vi "scanner v1.9.3.vi"() -> ()   [LabVIEW 2015]
uses:
  <vilib>/Analysis/Matrix/Datatypes/RealMatrix.ctl
  libs/Controls/String.ctl
  libs/Controls/Number.ctl
  libs/Controls/outofrange.ctl
  libs/Controls/loopclock.ctl
  libs/Controls/AcquisitionModuleStates.ctl
  <vilib>/Analysis/6fits.llb/Curve Fitting Criteria.ctl
  <vilib>/Utility/miscctls.llb/LVFormatAndPrecisionTypeDef.ctl
  <vilib>/Utility/file.llb/Write To Spreadsheet File (string).vi
  <vilib>/Utility/file.llb/Write Delimited Spreadsheet (I64).vi
  <vilib>/Utility/file.llb/Write To Spreadsheet File (DBL).vi
  libs/GlobalParameters/SpectraData2.vi
  <vilib>/Utility/file.llb/Read From Spreadsheet File (string).vi
  <vilib>/Analysis/Matrix/NI_Matrix.lvlib
  <vilib>/Analysis/NI_AALPro.lvlib
  Zaber A Series/Zaber A Series.lvlib
  libs/XGL_DPP.lvlib
panel:
  out "Error code 2":i32
  out "x/y":dbl
  out "Waveform Graph":dbl[][](graph)
  out "DPP Configuration":T1={"reset_recovery_time"=300, "edge_peaking_time"=5, "flat_top"=5, "peaking_time"=25, "gain"=1.0, "max_risetime"=35.0, "fast_filter_thr"=100, "zero_peak_freq"=5.0, "inverted_input"=0, "base_offset"=0, "reset_threshold"=1000, "overflow_recovery"=0, "tail_coefficient"=0.0, "energy_filter_thr"=25, "energy_baseline_thr"=25, "max_peaking_time"=0, "edge_flat_top"=1, "time_constant"=0.0, "baseline_samples"=64, "other_param"=0}
  in  "Precision [mm]":dbl=0.1
  out "Port":refnum<visa-resource-name>
  out "MotorsReady":bool
  out "Enum":T2=enum."SaveSpectra"
  out "init1Dset":dbl[][](array[numeric])
  out "3D":bool
  out "MAP":bool
  out "queue mode":bool
  out "scan mode":bool
  in  "Data folder path":path=path "d:/Users/XRF/Desktop/Scan DATA"
  out "Speed 2":T3 scale=0.0..30.0
  in  "Tab Control":T4(tab)
  in  "StopMotion":bool
  in  "GoToZ":bool
  in  "GoToY":bool
  in  "GoToX":bool
  in  "GoTo Z [mm]":dbl format="%#.8g"
  in  "GoTo Y [mm]":dbl format="%#.8g"
  in  "GoTo X [mm]":dbl format="%#.8g"
  out "ZnotEqual":bool
  out "ScanReady?":bool
  in  "OpenScanBuilder":bool
  in  "Clear":bool
  in  "LowerRight":bool
  in  "LowerLeft":bool
  in  "UpperRight":bool
  in  "UpperLeft":bool
  in  "Reduced Speed":bool
  in  "Speed Z [mm/s]":dbl(slide) caption="Z Speed\n[mm/s]" min=0.5 max=10.0 step=0.5 scale=0.5..10.0
  in  "XY Speed\n[mm/s]":dbl(slide)=1.0 min=1.0 max=75.0 step=1.0 scale=1.0..20.0
  in  "Away":bool
  in  "Closer":bool
  in  "Right":bool
  in  "Left":bool
  in  "Down":bool
  in  "Up":bool
  out "X [mm]":dbl format="%#.8g"
  out "Y [mm]":dbl format="%#.8g"
  out "Z [mm]":dbl format="%#.3g"
  out "Scan\nCorners":dbl[][](array[numeric])
  in  "QUICKSCAN_Start 2":bool
  in  "Add To Queue 2":bool
  out "Assignment":cluster{"Microstep Size":dbl, "Device":string}[](array[cluster])
  in  "Acceleration [mm/s^2]":dbl=1.0 min=1.0 max=488.0
  out "SpectraPlot":u64[](graph) caption="Waveform Graph"
  in  "APPEARANCE_CursorVis":bool
  in  "APPEARANCE_E/CH":bool
  in  "APPEARANCE_Log/Lin":bool=TRUE
  in  "Tab":enum32{"ACQUISITION", "ROIS", "CALIBRATION"}(tab)
  in  "Configure":bool
  in  "Time per spectrum [ms]":u32=10 max=1000000
  in  "Map points":u32=10
  in  "Acquisition mode":u16(ring) items=["Single spectrum", "Multiple spectra"]
  in  "Acquisition time [s]":fxp<+,64,32>=10.0
  out "Acq. in progress":bool
  in  "Stop":bool
  in  "Get connected":bool
  out "identifier out":string
  in  "IP Address":string="10.96.0.110"
  in  "Add IP":bool
  in  "Init":bool
  out "Real Time [s]":dbl=1.0 min=0.2 step=0.1
  out "Live Time [s]":dbl=1.0 min=0.2 step=0.1
  in  "MEASUREMENT_Start":bool
  out "Elapsed Time":dbl caption="Elapsed Time [s]" format="%#_4g"
  in  "Preset Time [s]":dbl=1.0 min=0.2 step=0.1
  out "Progress":u32 caption="%" min=1 step=1
  out "Library state":bool
  in  "?":bool
  in  "Config. file path":path=path "Configuration files/DefaultParameters.xml"
  out "Error code":i32
  in  "ROI_Load":bool
  in  "ROI_Save":bool
  in  "ROI_Cancel":bool
  in  "ROI_LowCh":u32=1800 caption="Lower Channel"
  in  "ROI_Set":bool
  in  "ROI_Add":bool
  in  "ROI_Remove":bool
  in  "ROI_RemoveAll":bool
  in  "ROI_UpCh":u32=2000 caption="Upper Channel"
  out "ROI_Array":T7(array[cluster]) {"ROI begin channel" step=0.001; "ROI end channel" step=0.001; "Intensity" step=0.001; "Net Intensity" step=0.001; "Gauss Fit" step=0.001; "FWHM [keV]" step=0.001; "Center [keV]" step=0.001}
  out "Intercept":dbl=-0.03941267387944358 caption="Intercept (keV)" format="%#_6f"
  out "Slope":dbl=0.010046367851622875 caption="Slope (keV/channel)" format="%#.6f"
  in  "CALIB_ClearPoints":bool
  in  "CALIB_AddPoint":bool
  in  "CalibArray":T8
  in  "CALIB_Execute":bool
  in  "SpectrumType":u16(ring) items=["Cumulative Spectra", "Max Spectra", "Last Spectra"]
  out "Cumul. LT[s]":dbl=1.0 min=0.0 step=1.0
  in  "Lin/Log":u16(ring) items=["Lin", "Log"]
  in  "Stop Button":bool
  out "/":i32=1 min=0 step=1
  out "current point":i32=1 min=0 step=1
  out "1D graph 1":dbl[](graph) caption="Map2"
  in  "MAP-L":u16(ring) items=["Cu-Ka", "All"]
  out "2D graph 2":dbl[][](graph) caption="A"
  out "2D graph 1":dbl[][](graph) caption="A"
  in  "MAP-R":u16(ring) items=["Cu-Ka", "All"]
  out "1D graph 2":dbl[](graph) caption="Map2"
  out "last point movement duration [ms]":u32
  in  "Free running":bool
  in  "PresetROI":u16(ring)
  in  "Preset type:":enum32{"Live time [s]", "Counts"}(radio)
  in  "Add To Queue":bool
  in  "ScanName:":string caption="Scan Name:"
  in  "Snake?":bool
  in  "PresetVal":dbl caption="Time Preset [s]"
  in  "QUICKSCAN_Start":bool
  in  "Scan order":u16(ring)=1 items=["X->Z->Y"=6, "Y->Z->X"=5, "Z->X->Y"=3, "Y->X->Z"=2, "Z->Y->X"=4, "X->Y->Z"=1]
  out "Z error":T9
  out "Y error":T9
  out "X error":T9
  out "total # of points":i32=1 min=0 step=1
  in  "Scan definition by":T10(radio)
  in  "Z steps":i32=1 min=1 step=1
  in  "step Z [mm]":dbl=1.0 min=0.0 step=0.1
  in  "Z end [mm]":dbl
  in  "Z start [mm]":dbl
  in  "Y steps":i32=1 min=1 step=1
  in  "X steps":i32=1 min=1 step=1
  in  "step Y [mm]":dbl=1.0 min=0.0 step=0.1
  in  "Y end [mm]":dbl=1.0
  in  "Y start [mm]":dbl
  in  "step X [mm]":dbl=1.0 min=0.0 step=0.1
  in  "X end [mm]":dbl=1.0
  in  "X start [mm]":dbl
  in  "Delete":bool
  in  "Text Ring":u16(ring)
  out "estimated duration":string caption="Estimated duration:"
  out "NoOfScans":i32=1 min=0 step=1
  in  "QUEUE_Stop":bool
  in  "QUEUE_Run":bool
  out "ScanQueue":T11(array[cluster])
  in  "Clear_Queue":bool
  out "SumSpectra":u64[](array[numeric])
  out "MaxSpectra":u64[](array[numeric])
  out "Array of positions":dbl[][](array[numeric])
  out "LastSpectra":u32[](graph) caption="Waveform Graph"
  out "maps folder":path
  out "spectra folder":path
  out "roi intensities 2d":dbl[](array[numeric])
  out "Array":dbl[](array[numeric])
  out "2DSet":dbl[][][](array[numeric])
  out "1DSet":dbl[][](array[numeric])
  out "1DPosArray":dbl[](array[numeric])
  out "appended path":path
  out "Numeric":i32
  out "ScanData":T12
  out "ZaberError":errorcluster
  out "ReadoutTiming":u32[](array[numeric])
  out "Loop Speed [1/s]":dbl caption="Elapsed Time [s]" format="%#_2f"
  # "This is for debugging purposes"
  # "Capture position as:"
  # "ROI  Name       Begin           End         Intensity    Net intnsity   Gauss Fit      FWHM         Center\n                         channel      channel                                                              [keV]            [keV]"
  # "Point               Channel      Energy (keV)"
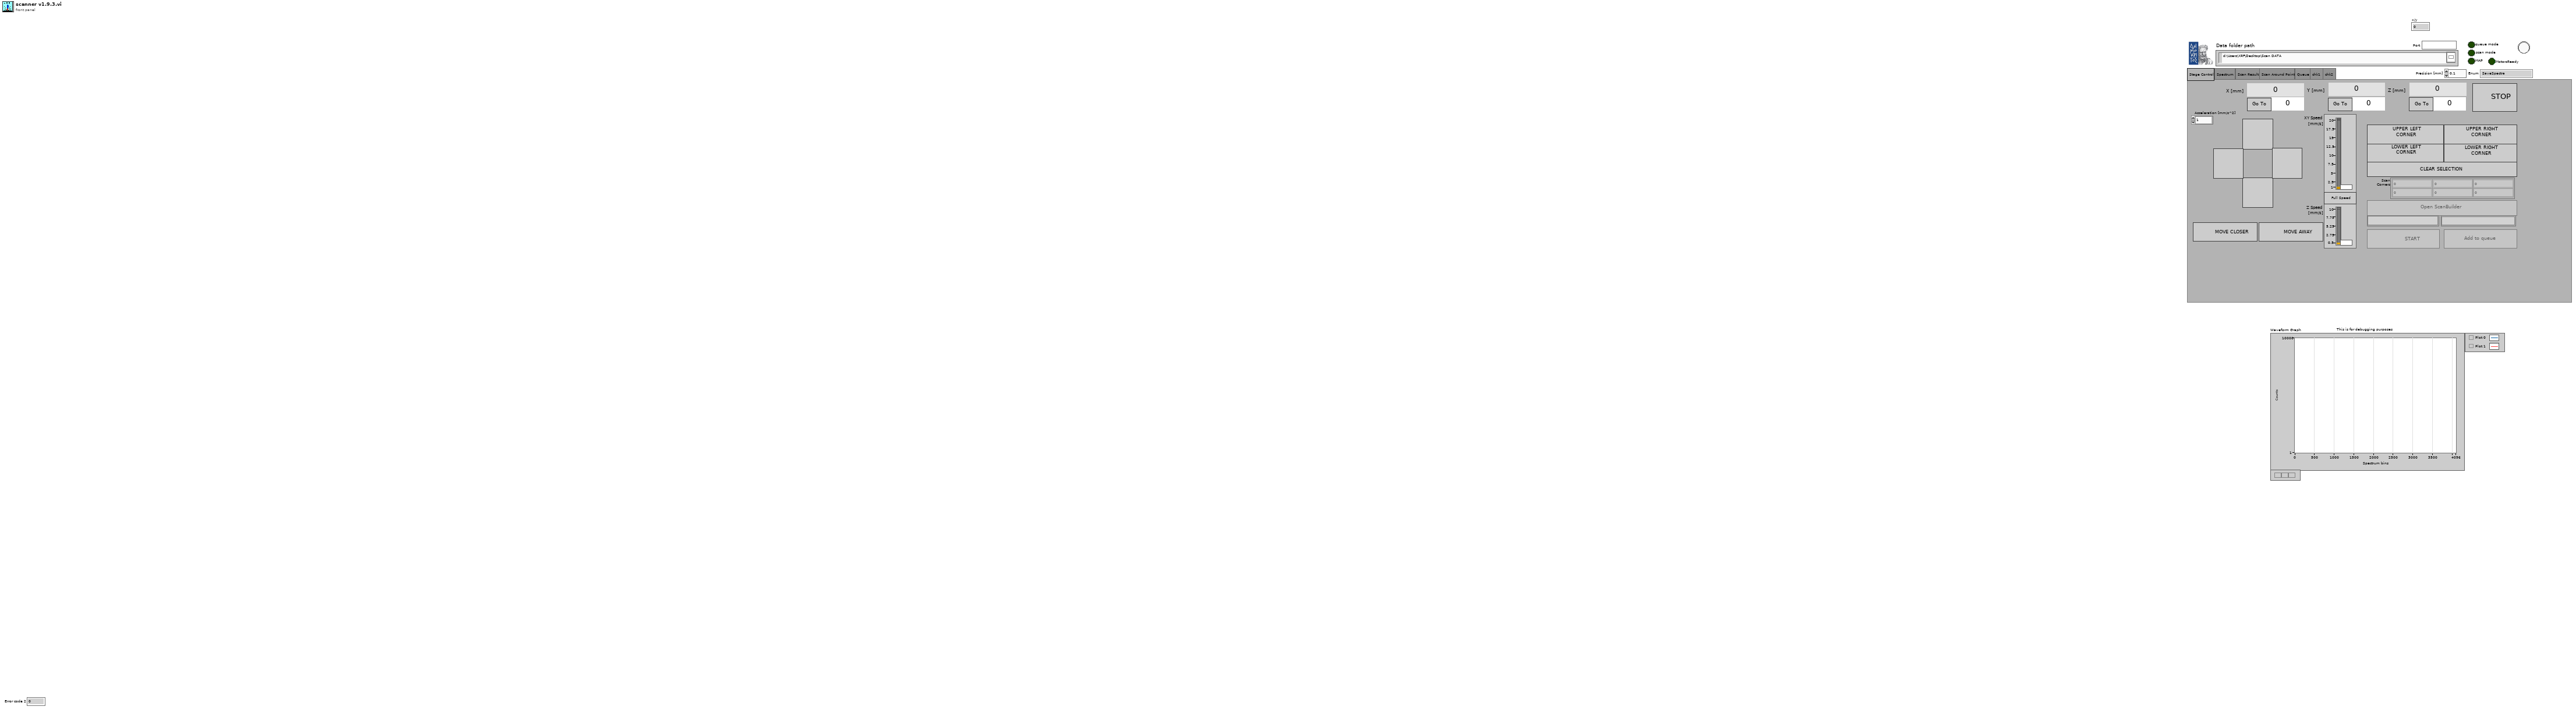
[diagram p1: front panel]
types:
  T1 = cluster{"reset_recovery_time":u32, "edge_peaking_time":u32, "flat_top":u32, "peaking_time":u32, "gain":dbl, "max_risetime":dbl, "fast_filter_thr":u32, "zero_peak_freq":dbl, "inverted_input":u8, "base_offset":u32, "reset_threshold":u32, "overflow_recovery":u32, "tail_coefficient":dbl, "energy_filter_thr":u32, "energy_baseline_thr":u32, "max_peaking_time":u32, "edge_flat_top":u32, "time_constant":dbl, "baseline_samples":u32, "other_param":u32}
  T2 = typedef "AcquisitionModuleStates.ctl" = enum16{"Close", "PrepareMap", "MoveToPoint", "DisplayData", "SaveSpectra", "Acquire", "IDLE", "Initialisation"}
  T3 = typedef "loopclock.ctl" = dbl
  T4 = enum32{"Stage Control", "Spectrum", "Scan Result", "Scan Around Point", "Queue", "chk1", "chk2"}
  T5 = typedef "String.ctl" = string
  T6 = typedef "Number.ctl" = dbl
  T7 = cluster{"ROI name":T5, "ROI begin channel":T6, "ROI end channel":T6, "Intensity":T6, "Net Intensity":T6, "Gauss Fit":T6, "FWHM [keV]":T6, "Center [keV]":T6}[]
  T8 = typedef "NI_Matrix.lvlib/RealMatrix.ctl" = dbl[][]
  T9 = typedef "outofrange.ctl" = bool
  T10 = enum32{"Step size and step number", "Scan boundaries and step size", "Scan boundaries and number of steps"}
  T11 = cluster{"Scan\nCoords \n[mm]":cluster{"X abs start":dbl, "X abs end":dbl, "Y abs start":dbl, "Y abs end":dbl, "Z abs start":dbl, "Z abs end":dbl, "X step":dbl, "Y step":dbl, "Z step":dbl}, "PresetVal":dbl, "Order":u16, "Snake?":bool, "Name":string, "#points":i32, "CtsPreset?":bool, "CtPsetROI":i32}[]
  T12 = cluster{"ScanCoords [mm]":cluster{"X abs start":dbl, "X abs end":dbl, "Y abs start":dbl, "Y abs end":dbl, "Z abs start":dbl, "Z abs end":dbl, "X step":dbl, "Y step":dbl, "Z step":dbl}, "PresetVal":dbl, "Order":u16, "Snake?":bool, "Name":string, "#points":i32, "CtPreset?":bool, "CtPsetROI":i32}
  T13 = cluster{"X min":dbl, "X max":dbl, "Y min":dbl, "Y max":dbl, "Z min":dbl, "Z max":dbl}
  T14 = enum32{"Size Tabs To Contents", "Size All Tabs to Largest Tab", "Fixed Tab Size"}
  T15 = enum8{"Enabled", "Disabled", "Disabled and Grayed Out"}
  T16 = cluster{"ScanCoords [mm]":cluster{"X abs start":dbl, "X abs end":dbl, "Y abs start":dbl, "Y abs end":dbl, "Z abs start":dbl, "Z abs end":dbl, "X step":dbl, "Y step":dbl, "Z step":dbl}, "PresetVal":dbl, "Order":u16, "Snake?":bool, "Name":string, "#points":i32, "ChrgPreset?":bool, "CtPrstROI":i32}
  T17 = cluster{"ROI name":string, "ROI begin channel":i64, "ROI end channel":i64, "Intensity":i64, "Net Intensity":i64, "Gauss Fit":dbl, "FWHM [keV]":dbl, "Center [keV]":dbl}
  T18 = typedef "LVFormatAndPrecisionTypeDef.ctl" = cluster{"Format":u8, "Precision":u8}
  T19 = cluster{"Scan\nCoords \n[mm]":cluster{"X abs start":dbl, "X abs end":dbl, "Y abs start":dbl, "Y abs end":dbl, "Z abs start":dbl, "Z abs end":dbl, "X step":dbl, "Y step":dbl, "Z step":dbl}, "PresetVal":dbl, "Order":u16, "Snake?":bool, "Name":string, "#points":i32, "CtsPreset?":bool, "CtPsetROI":i32}
  T20 = cluster{"X abs start":dbl, "X abs end":dbl, "Y abs start":dbl, "Y abs end":dbl, "Z abs start":dbl, "Z abs end":dbl, "X step":dbl, "Y step":dbl, "Z step":dbl}
  T21 = cluster{"ScanCoords [mm]":cluster{"X abs start":dbl, "X abs end":dbl, "Y abs start":dbl, "Y abs end":dbl, "Z abs start":dbl, "Z abs end":dbl, "X step":dbl, "Y step":dbl, "Z step":dbl}, "PresetVal":dbl, "Order":u16, "Snake?":bool, "Name":string, "#points":i32, "CtPreset?":bool, "CtPsetROI":i32}[]
  T22 = enum16{"Left Button", "Center Button", "Right Button", "Window Close"}
  T23 = cluster{"ScanCoords [mm]":cluster{"X abs start":dbl, "X abs end":dbl, "Y abs start":dbl, "Y abs end":dbl, "Z abs start":dbl, "Z abs end":dbl, "X step":dbl, "Y step":dbl, "Z step":dbl}, "PresetVal":dbl, "Order":u16, "Snake?":bool, "Name":string, "#points":i32, "ChrgPreset?":bool, "CtPsetROI":u16}
  T24 = typedef "LVMinMaxIncTypeDef.ctl" = cluster{"Minimum":dbl, "Maximum":dbl, "Increment":dbl}
  T25 = typedef "LVRangeTypeDef.ctl" = cluster{"Minimum":dbl, "Maximum":dbl, "Increment":dbl, "Minor Increment":dbl, "Start":dbl}
  T26 = typedef "ConfigurationDPP.ctl" = cluster{"reset_recovery_time":u32, "edge_peaking_time":u32, "flat_top":u32, "peaking_time":u32, "gain":dbl, "max_risetime":dbl, "fast_filter_thr":u32, "zero_peak_freq":dbl, "inverted_input":u8, "base_offset":u32, "reset_threshold":u32, "overflow_recovery":u32, "tail_coefficient":dbl, "energy_filter_thr":u32, "energy_baseline_thr":u32, "max_peaking_time":u32, "edge_flat_top":u32, "time_constant":dbl, "baseline_samples":u32, "other_param":u32}
  T27 = cluster{"ROI name":string, "ROI begin channel":i64, "ROI end channel":i64, "Intensity":i64, "Net Intensity":i64, "Gauss Fit":dbl, "FWHM [keV]":dbl, "Center [keV]":dbl}[]
  T28 = typedef "NI_AALPro.lvlib/Curve Fitting Criteria.ctl" = u16
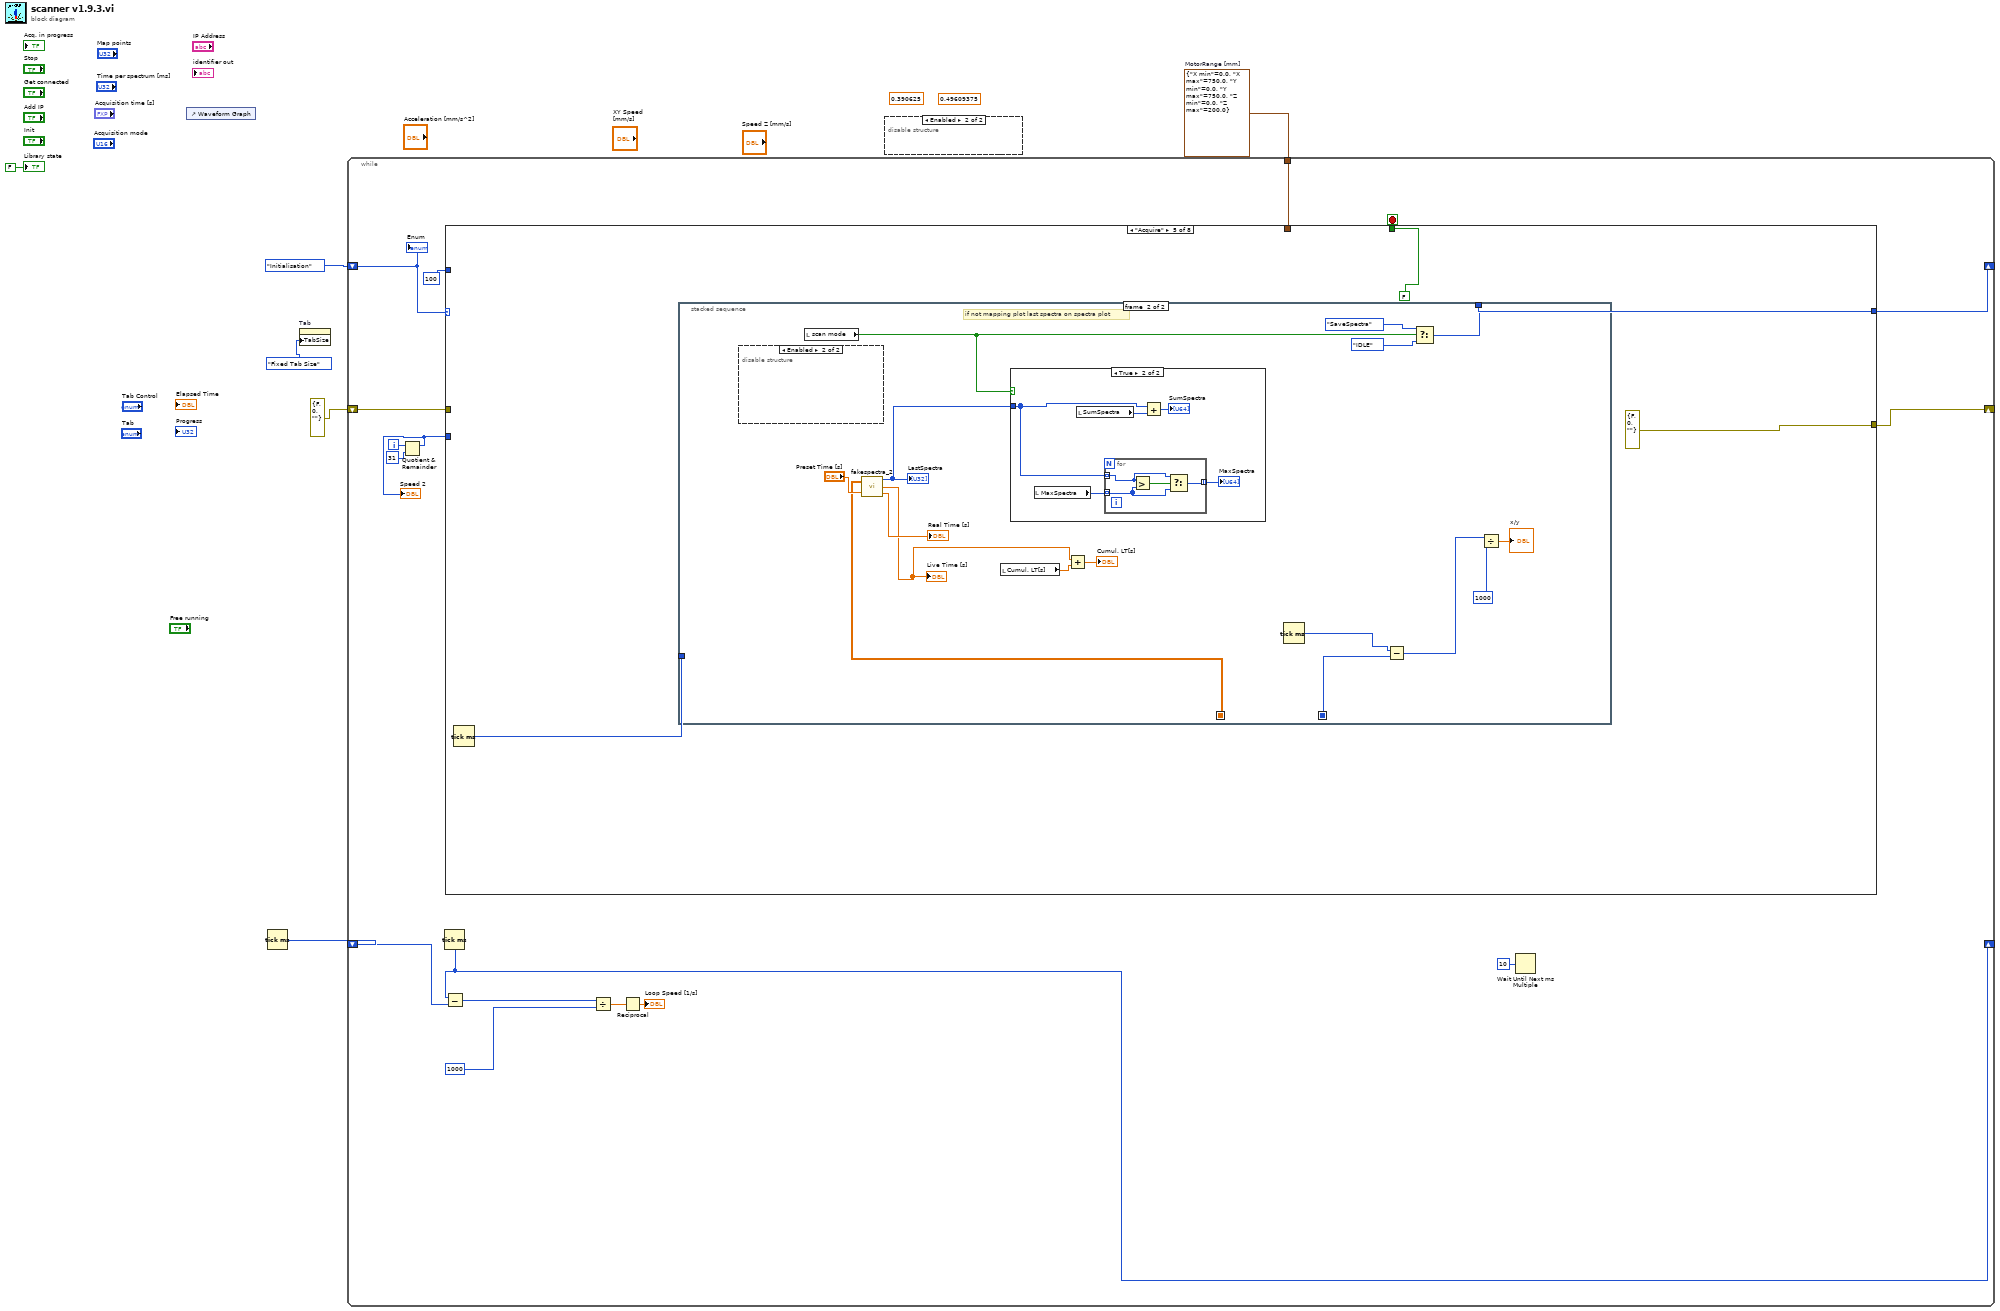
[diagram p0: block diagram]
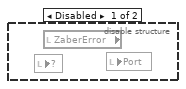
[diagram p2: hidden frame]
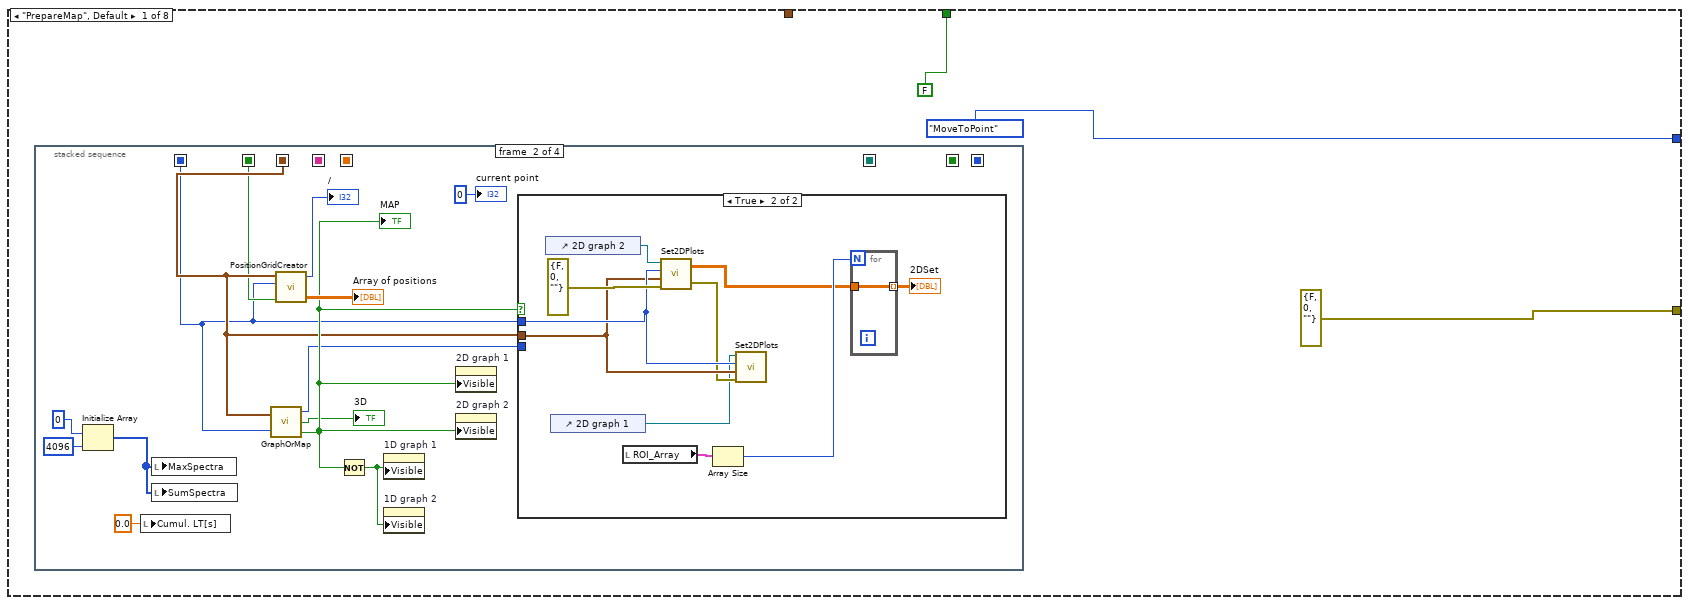
[diagram p3: hidden frame]
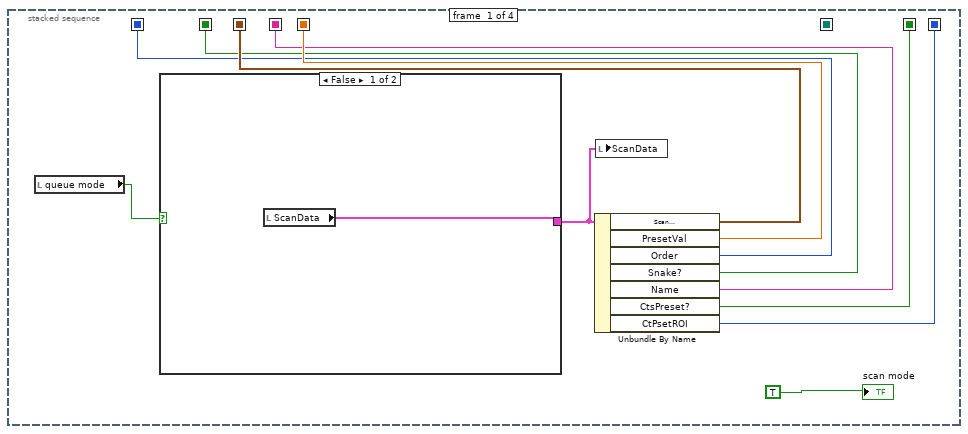
[diagram p4: hidden frame]
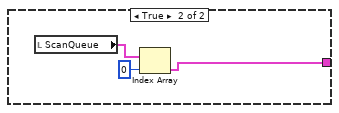
[diagram p5: hidden frame]
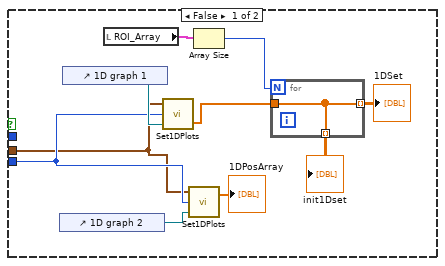
[diagram p6: hidden frame]
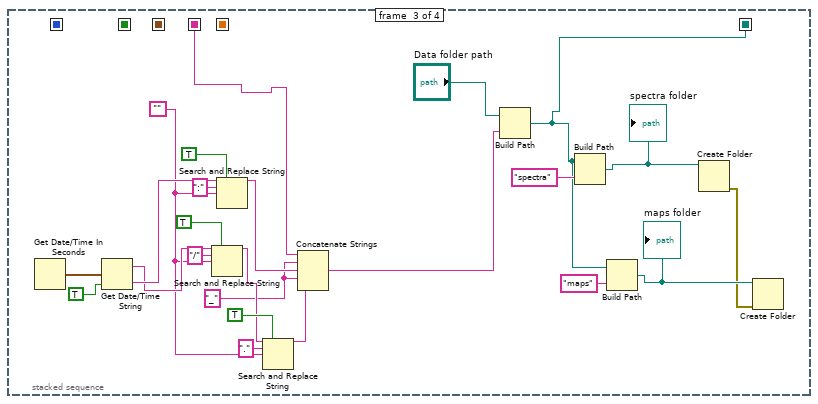
[diagram p7: hidden frame]
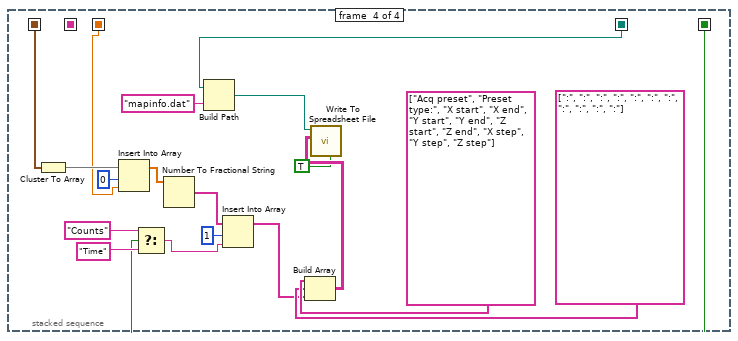
[diagram p8: hidden frame]
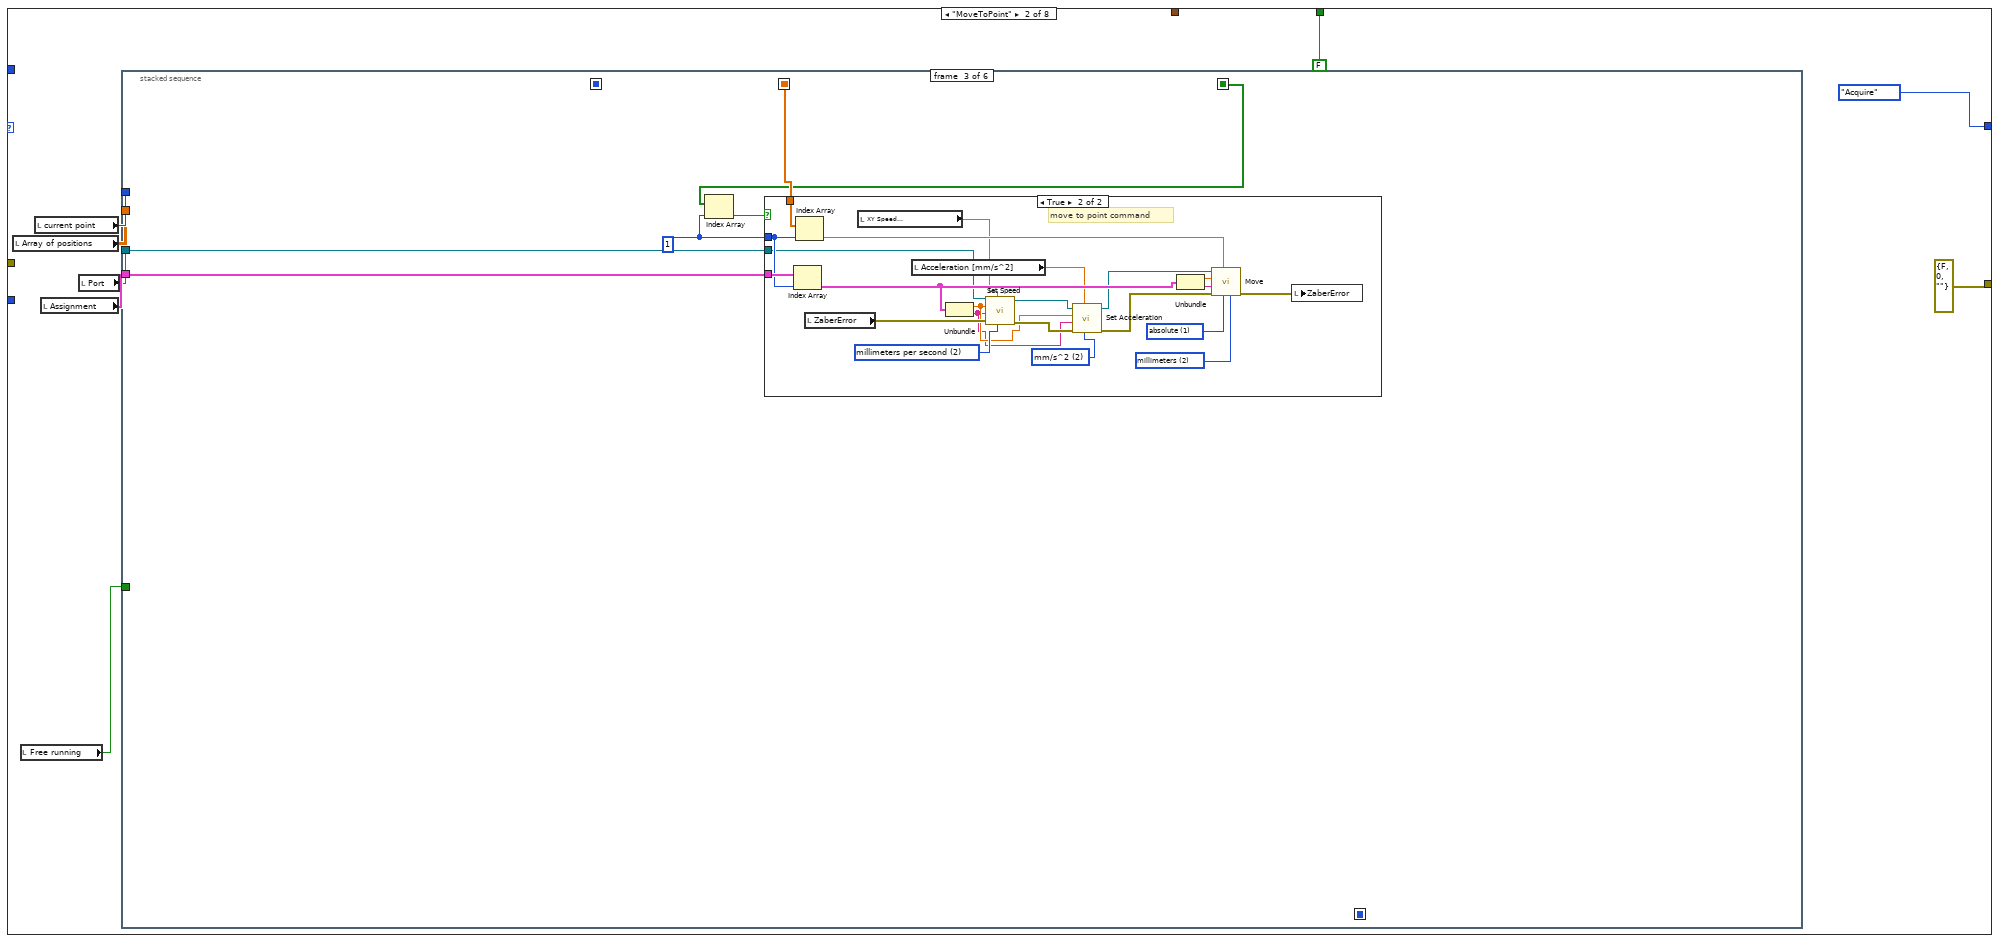
[diagram p9: hidden frame]
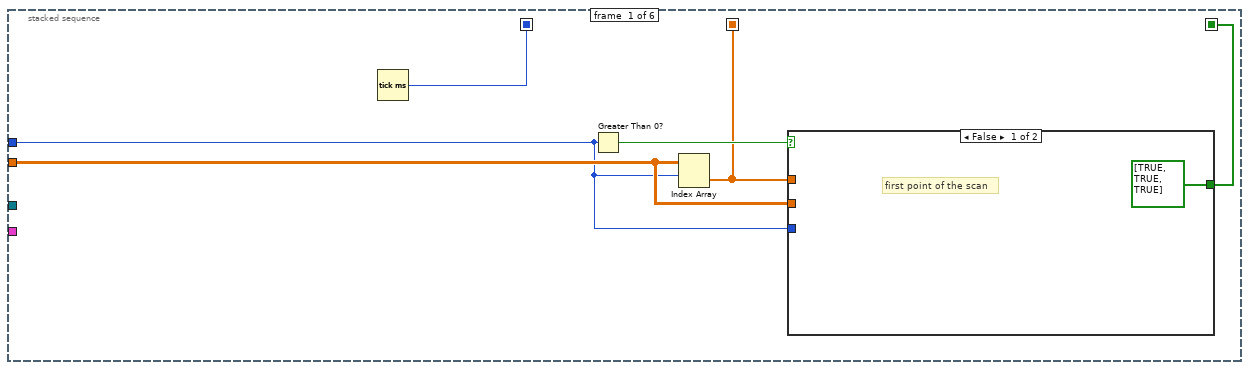
[diagram p10: hidden frame]
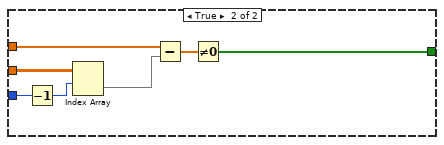
[diagram p11: hidden frame]
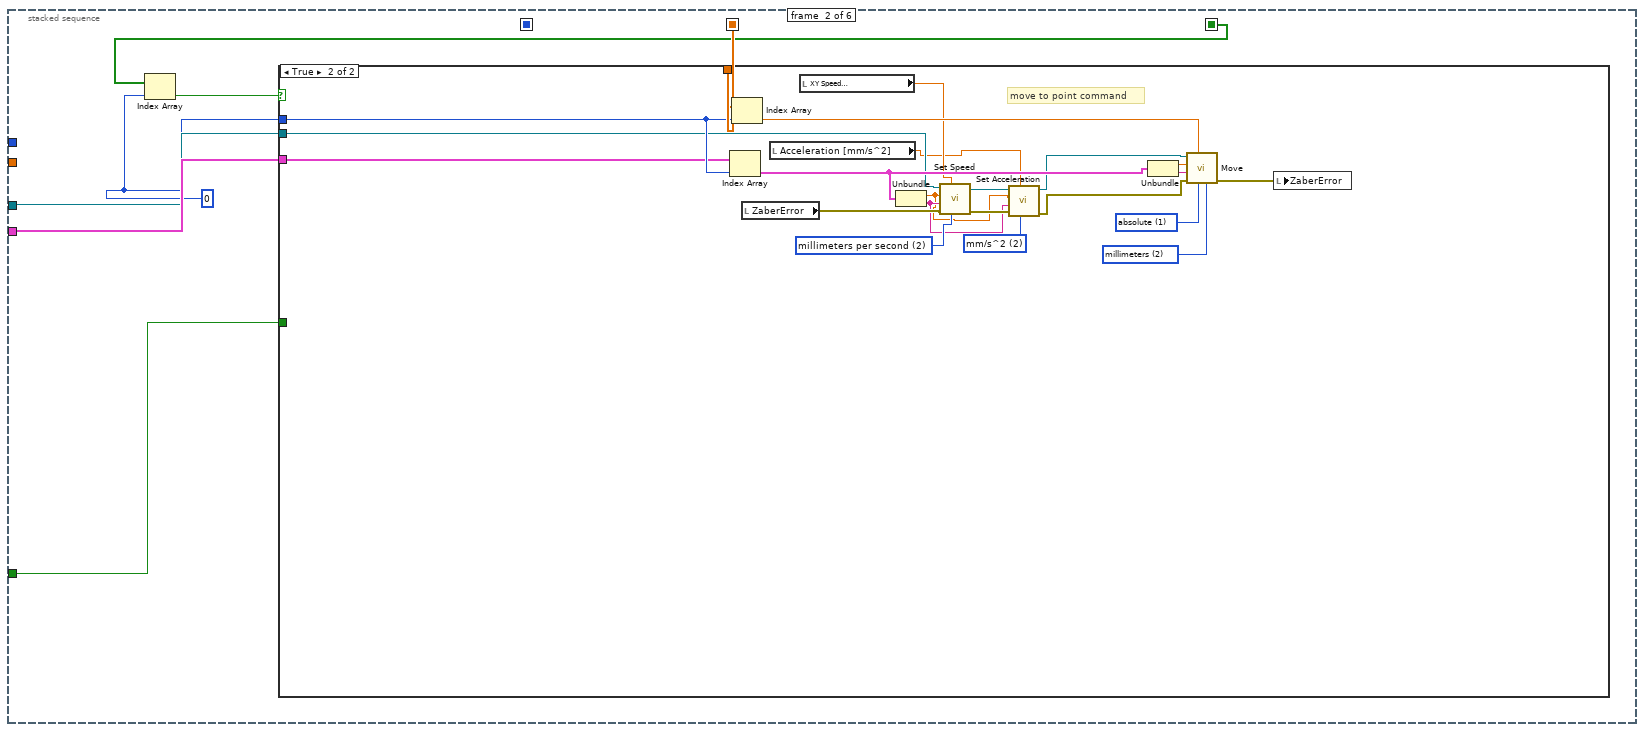
[diagram p12: hidden frame]
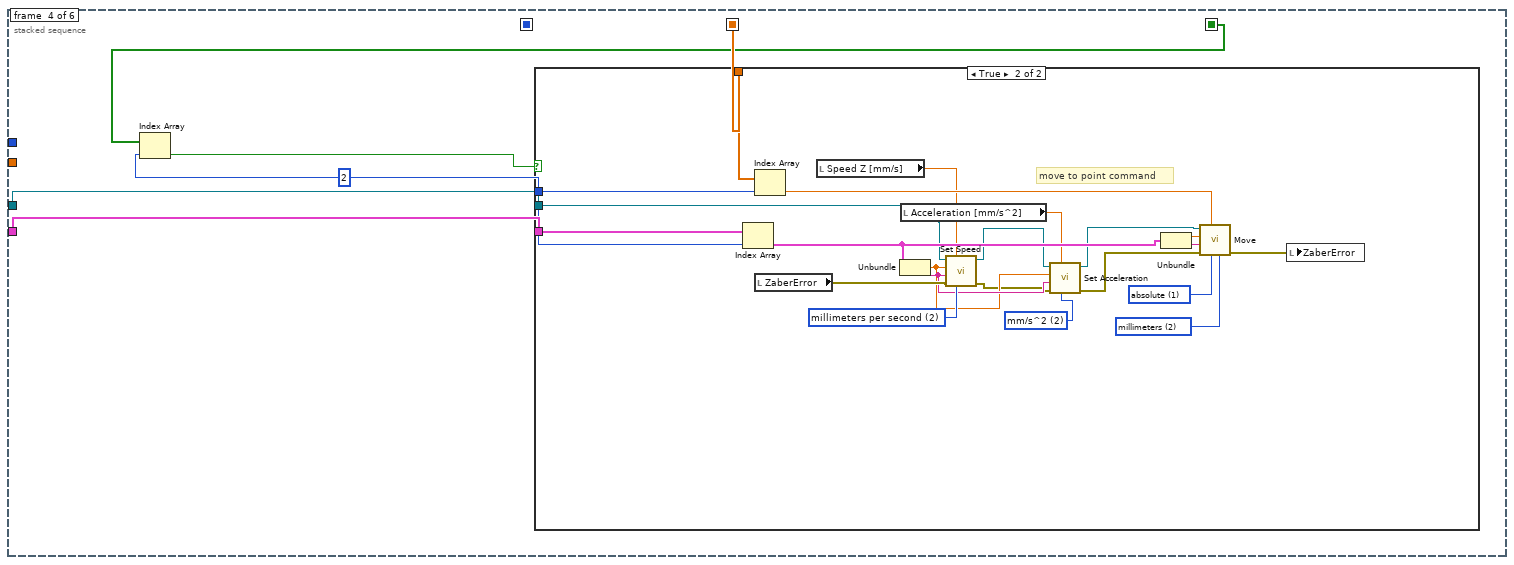
[diagram p15: hidden frame]
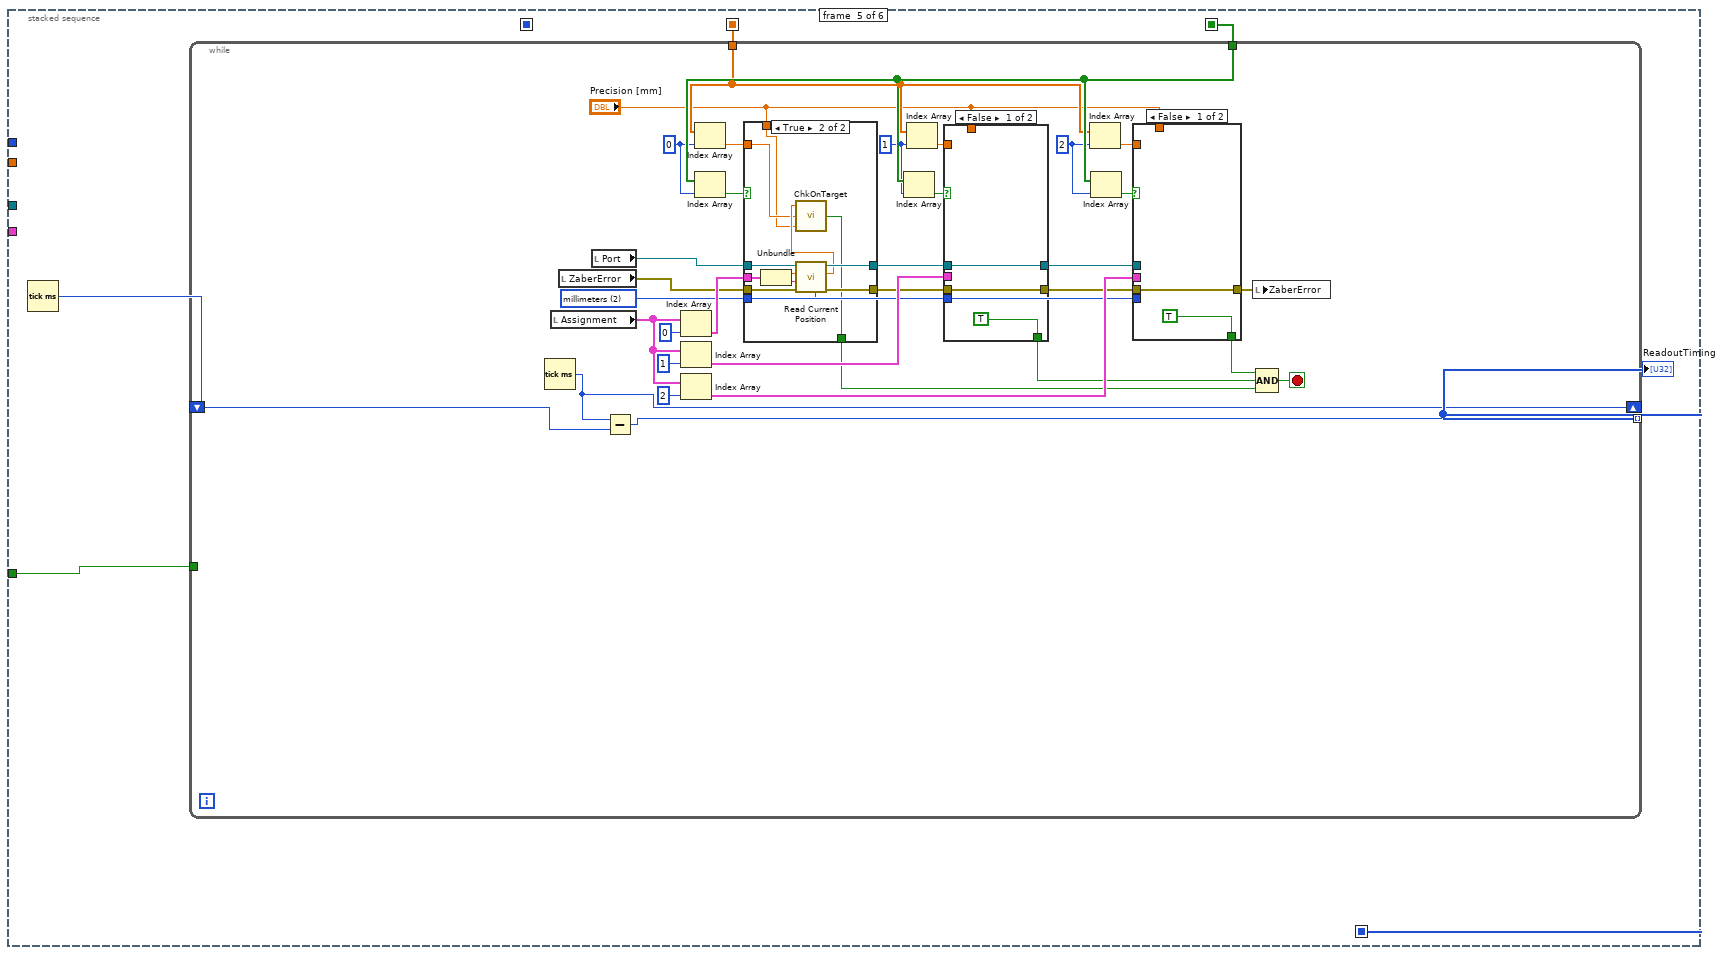
[diagram p17: hidden frame]
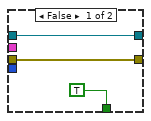
[diagram p18: hidden frame]
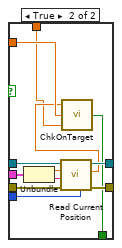
[diagram p19: hidden frame]
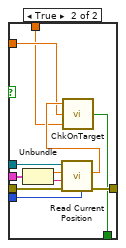
[diagram p20: hidden frame]
diagram:
  (unwired) 0.49609375 ("Microstep Size (0)")
  (unwired) 0.390625 ("Microstep Size (0)")
  w3 = T13 {"X min"=0.0, "X max"=750.0, "Y min"=0.0, "Y max"=750.0, "Z min"=0.0, "Z max"=200.0}  # MotorRange [mm]
  n1 = control-ref of="Waveform Graph"() -> ()  [unwired: 1 out]
  n2 = Tick Count (ms)() -> (millisecond timer value=w6:u32)
  n3 = property on="Tab" class="TabCtl (strict)"("TabSize"=T14."Fixed Tab Size" ("Tab Size")) -> ()  [unwired: 2 in, 2 out]
  n4 = while {
    shift-right: [w11] -> _
    shift-left: AcquisitionModuleStates."Initialisation" ("Enum") -> [w12]
    shift-right: [w19] -> _
    shift-left: w6 -> [w23]
    tunnel: w3 -> [w10]
    shift-right: [w7] -> _
    shift-left: errorcluster {"status"=FALSE, "code"=0, "source"=""} ("error out") -> [w8]
    i -> [w16]
    stop <- w17 stop-if-true
    n5 = Quotient & Remainder(x=w16, y=31) -> (x-y*floor(x/y)=w9:i32)  [unwired: 1 out]
    "Speed 2" <- w9
    n6 = Tick Count (ms)() -> (millisecond timer value=w19:u32)
    n7 = case shown="\"Acquire\"" w12 {
      tunnel: 100 ("LoopTimer [ms]") -> [_ _ _ _ _ w646 _ _]
      tunnel: [FALSE ("VI stop") FALSE ("VI stop") FALSE ("VI stop") FALSE ("VI stop") FALSE ("VI stop") w645 FALSE ("VI stop") TRUE ("VI stop")] -> w17
      tunnel: w9 -> [_ _ _ _ _ _ _ _]
      tunnel: [AcquisitionModuleStates."MoveToPoint" ("Enum") AcquisitionModuleStates."Acquire" ("Enum") AcquisitionModuleStates."IDLE" ("Enum") w556 w589 w644 AcquisitionModuleStates."IDLE" ("Enum") AcquisitionModuleStates."Close" ("Enum")] -> w11
      tunnel: w10 -> [_ _ _ _ _ w642 _ _]
      tunnel: w8 -> [_ _ _ _ _ w641 _ _]
      tunnel: [errorcluster {"status"=FALSE, "code"=0, "source"=""} ("error out") errorcluster {"status"=FALSE, "code"=0, "source"=""} ("error out") errorcluster {"status"=FALSE, "code"=0, "source"=""} ("error out") errorcluster {"status"=FALSE, "code"=0, "source"=""} ("error out") errorcluster {"status"=FALSE, "code"=0, "source"=""} ("error out") w640 errorcluster {"status"=FALSE, "code"=0, "source"=""} ("error out") errorcluster {"status"=FALSE, "code"=0, "source"=""} ("error out")] -> w7
      frame "PrepareMap", Default {
        n8 = stacked-sequence {
          seq-local: [w35 _ _ _] -> [_ w43 _ w114]
          seq-local: [_ _ w78 _] -> [_ _ _ w116]
          seq-local: [w32 _ _ _] -> [_ w42 _ _]
          seq-local: [w30 _ _ _] -> [_ w41 _ _]
          seq-local: [w31 _ _ _] -> [_ _ w77 _]
          seq-local: [w34 _ _ _] -> [_ _ _ w109]
          seq-local: [w28 _ _ _] -> [_ _ _ w101]
          seq-local: [w27 _ _ _] -> [_ _ _ _]
          frame #0 {
            n9 = local read "queue mode"() -> (w36:bool)
            n10 = case shown="False" w36 {
              tunnel: [w37 w38] -> w29
              frame False {
                n11 = local read "ScanData"() -> (w37:T12)
              }
              frame True {
                n12 = local read "ScanQueue"() -> (w40:T11)
                n13 = Index Array(array=w40, index=0) -> (element=w38:T19)
              }
            }
            n14 = Unbundle By Name(w29) -> ("Scan\nCoords \n[mm]"=w35:T20, "PresetVal"=w34:dbl, "Order"=w30:u16, "Snake?"=w32:bool, "Name"=w31:string, "CtsPreset?"=w28:bool, "CtPsetROI"=w27:i32)
            n15 = local write "ScanData"(w29) -> ()
            "scan mode" <- TRUE
          }
          frame #1 {
            n16 = Initialize Array(u64 0, 4096 ("dimension size")) -> (w46:u64[])
            n17 = local write "Cumul. LT[s]"(0.0 ("Cumul. LT[s]")) -> ()
            n18 = local write "MaxSpectra"(w46) -> ()
            n19 = local write "SumSpectra"(w46) -> ()
            n20 = call "GraphOrMap.vi"("ScanCoords [mm]"=w43, "Order selection"=w41) -> ("Axis for graph"=w51:i32, "3D"=→"3D":bool, "MAP"=w52:bool)
            "MAP" <- w52
            n21 = call "PositionGridCreator.vi"("invert?"=w42, "Select order"=w41, "ScanCoords [mm]"=w43) -> ("Array of positions"=→"Array of positions":dbl[][], "total number of steps"=→"/":i32)  [unwired: 1 in, 1 out]
            n22 = Not(x=w52) -> (.not. x?=w53:bool)
            n23 = property on="1D graph 1" class="WFGraph (strict)"("Visible"=w53) -> ()  [unwired: 2 in, 2 out]
            n24 = property on="1D graph 2" class="WFGraph (strict)"("Visible"=w53) -> ()  [unwired: 2 in, 2 out]
            n25 = property on="2D graph 1" class="IntGraph (strict)"("Visible"=w52) -> ()  [unwired: 2 in, 2 out]
            n26 = property on="2D graph 2" class="IntGraph (strict)"("Visible"=w52) -> ()  [unwired: 2 in, 2 out]
            n27 = case shown="True" w52 {
              tunnel: w41 -> [_ w70]
              tunnel: w43 -> [w62 w69]
              tunnel: w51 -> [w63 _]
              frame False {
                n28 = control-ref of="1D graph 2"() -> (w61:refnum<vi>)
                n29 = control-ref of="1D graph 1"() -> (w64:refnum<vi>)
                n30 = local read "ROI_Array"() -> (w60:T7)
                n31 = call "Set1DPlots.vi"("1D graph"=w64, "Axis for graph"=w63, "ScanCoords [mm]"=w62) -> ("InitArray"=w58:dbl[])  [unwired: 1 out]
                n32 = call "Set1DPlots.vi"("1D graph"=w61, "Axis for graph"=w63, "ScanCoords [mm]"=w62) -> ("PosArray"=→"1DPosArray":dbl[])  [unwired: 1 out]
                n33 = Array Size(array=w60) -> (size(s)=w59:i32)
                n34 = for {
                  N: w59 -> [_]
                  tunnel: [w65] -> w57 mode=indexing
                  tunnel: w58 -> [w65]
                  tunnel: [w65] -> w55 mode=indexing
                }
                "1DSet" <- w57
                "init1Dset" <- w55
              }
              frame True {
                n35 = control-ref of="2D graph 2"() -> (w67:refnum<vi>)
                n36 = control-ref of="2D graph 1"() -> (w66:refnum<vi>)
                n37 = local read "ROI_Array"() -> (w75:T7)
                n38 = call "Set2DPlots.vi"("error in (no error)"=errorcluster {"status"=FALSE, "code"=0, "source"=""}, "ScanCoords [mm]"=w69, "Order selection"=w70, "2D graph 3"=w67) -> ("error out"=w68:errorcluster, "initialized array"=w73:dbl[][])
                n39 = Array Size(array=w75) -> (size(s)=w74:i32)
                n40 = call "Set2DPlots.vi"("error in (no error)"=w68, "ScanCoords [mm]"=w69, "Order selection"=w70, "2D graph 3"=w66) -> ()  [unwired: 2 out]
                n41 = for {
                  N: w74 -> [_]
                  tunnel: w73 -> [w76]
                  tunnel: [w76] -> w72 mode=indexing
                }
                "2DSet" <- w72
              }
            }
            "current point" <- 0 ("current point")
          }
          frame #2 {
            w81 = "_"
            w82 = ""
            n42 = Get Date/Time In Seconds() -> (seconds since 1Jan1904=w95:timestamp)
            n43 = Get Date/Time String(seconds (now)=w95, want seconds? (F)=TRUE) -> (date string=w90:string, time string=w93:string)  [unwired: 1 in]
            n44 = Search and Replace String(replace all?=TRUE ("replace all? (F)"), input string=w90, search string="/", replace string=w82) -> (result string=w84:string)  [unwired: 4 in, 3 out]
            n45 = Search and Replace String(replace all?=TRUE ("replace all? (F)"), input string=w93, search string=":", replace string=w82) -> (result string=w92:string)  [unwired: 4 in, 3 out]
            n46 = Search and Replace String(replace all?=TRUE ("replace all? (F)"), input string=w84, search string=".", replace string=w82) -> (result string=w83:string)  [unwired: 4 in, 3 out]
            n47 = Concatenate Strings(w77, w81, w92, w81, w83) -> (w80:string)
            n48 = Build Path(base path="Data folder path", name or relative path=w80) -> (appended path=w78:path)
            n49 = Build Path(base path=w78, name or relative path="spectra") -> (appended path=w97:path)
            "spectra folder" <- w97
            n50 = Build Path(base path=w78, name or relative path="maps") -> (appended path=w96:path)
            "maps folder" <- w96
            n51 = Create Folder(path (use dialog)=w97) -> (error out=w79:errorcluster)  [unwired: 2 in, 2 out]
            n52 = Create Folder(path (use dialog)=w96, error in=w79) -> ()  [unwired: 1 in, 3 out]
          }
          frame #3 {
            n53 = Cluster To Array(cluster=w114) -> (array=w119:dbl[])
            n54 = Insert Into Array(array=w119, index=0, new element=w109) -> (w108:dbl[])
            n55 = Select(t="Counts", s=w101, f="Time") -> (s? t:f=w102:string)
            n56 = Number To Fractional String(number=w108) -> (F-format string=w106:string[])  [unwired: 3 in]
            n57 = Build Path(base path=w116, name or relative path="mapinfo.dat") -> (appended path=w117:path)
            n58 = Insert Into Array(array=w106, index=1, new element=w102) -> (w105:string[])
            n59 = Build Array(string[] ["Acq preset", "Preset type:", "X start", "X end", "Y start", "Y end", "Z start", "Z end", "X step", "Y step", "Z step"], string[] [":", ":", ":", ":", ":", ":", ":", ":", ":", ":", ":"], w105) -> (w113:string[][])
            n60 = call-poly <vilib>:"Write To Spreadsheet File.vi"("transpose? (no:F)"=TRUE, "2D data"=w113, "file path (dialog if empty)"=w117) -> ()  [unwired: 5 in, 1 out]
          }
        }
      }
      frame "MoveToPoint" {
        n61 = local read "Array of positions"() -> (w123:dbl[][])
        n62 = local read "Free running"() -> (w120:bool)
        n63 = local read "current point"() -> (w124:i32)
        n64 = local read "Assignment"() -> (w126:cluster{"Microstep Size":dbl, "Device":string}[])
        n65 = local read "Port"() -> (w125:refnum<visa-resource-name>)
        n66 = stacked-sequence {
          seq-local: [w130 _ _ _ _ _] -> [_ w146 w174 w202 w230 _]
          seq-local: [w129 _ _ _ _ _] -> [_ w145 w172 w200 w231 _]
          seq-local: [_ _ _ _ w228 _] -> [_ _ _ _ _ w323]
          seq-local: [w128 _ _ _ _ _] -> [_ _ _ _ _ w321]
          tunnel: w126 -> [_ w148 w176 w204 _ _]
          tunnel: w125 -> [_ w147 w175 w203 _ _]
          tunnel: w124 -> [w131 _ _ _ _ _]
          tunnel: w123 -> [w132 _ _ _ _ _]
          tunnel: w120 -> [_ w142 _ _ w227 _]
          frame #0 {
            n67 = Tick Count (ms)() -> (millisecond timer value=w128:u32)
            n68 = Greater Than 0?(x=w131) -> (x > 0?=w133:bool)
            n69 = Index Array(array=w132, index (row)=w131) -> (element=w130:dbl[])  [unwired: 1 in]
            n70 = case shown="False" w133 {
              tunnel: w132 -> [_ w141]
              tunnel: w131 -> [_ w140]
              tunnel: w130 -> [_ w137]
              tunnel: [bool[] [TRUE, TRUE, TRUE] w135] -> w129
              frame False {
                # "first point of the scan"
              }
              frame True {
                n71 = Decrement(x=w140) -> (x-1=w139:i32)
                n72 = Index Array(array=w141, index (row)=w139) -> (element=w138:dbl[])  [unwired: 1 in]
                n73 = Subtract(x=w137, y=w138) -> (x-y=w136:dbl[])
                n74 = Not Equal To 0?(x=w136) -> (x != 0?=w135:bool[])
              }
            }
          }
          frame #1 {
            w143 = 0 ("index")
            n75 = Index Array(array=w145, index=w143) -> (element=w144:bool)
            n76 = case shown="True" w144 {
              tunnel: w143 -> [_ w163]
              tunnel: w148 -> [_ w162]
              tunnel: w147 -> [_ w160]
              tunnel: w146 -> [_ w161]
              tunnel: w142 -> [_ _]
              frame False {
              }
              frame True {
                w150 = u16 2 items=["device units", "microns/s^2", "mm/s^2", "inches/s^2", "degrees/s^2"] ("Units (0: data)")
                w158 = u16 2 items=["device speed units", "microns per second", "millimeters per second", "inches per second", "degrees per second"] ("Units (0: device speed units)")
                w168 = u16 2 items=["microsteps", "microns", "millimeters", "inches", "degrees"] ("Units (0: microsteps)")
                w170 = u16 1 items=["relative", "absolute"] ("Movement Type (0: relative)")
                # "move to point command"
                n77 = Index Array(array=w162, index=w163) -> (element=w165:cluster{"Microstep Size":dbl, "Device":string})
                n78 = Index Array(array=w161, index=w163) -> (element=w164:dbl)
                n79 = local read "ZaberError"() -> (w159:errorcluster)
                n80 = local read "Acceleration [mm/s^2]"() -> (w149:dbl)
                n81 = local read "XY Speed\n[mm/s]"() -> (w157:dbl)
                n82 = Unbundle(w165) -> ("Microstep Size"=w151:dbl, "Device"=w152:string)
                n83 = call "Set Speed.vi"("Units (0: data)"=w158, "New Speed"=w157, "error in (no error)"=w159, "Device and Axis"=w152, "Microstep Size (0)"=w151, "VISA resource name"=w160) -> ("error out"=w154:errorcluster, "VISA resource name out"=w156:refnum<visa-resource-name>)  [unwired: 4 in]
                n84 = call "Set Acceleration.vi"("Units (0: data)"=w150, "New Acceleration"=w149, "error in (no error)"=w154, "Device and Axis"=w152, "Microstep Size (0)"=w151, "VISA resource name"=w156) -> ("error out"=w153:errorcluster, "VISA resource name out"=w155:refnum<visa-resource-name>)  [unwired: 4 in]
                n85 = Unbundle(w165) -> ("Microstep Size"=w167:dbl, "Device"=w166:string)
                n86 = call "Move.vi"("Units (0: microsteps)"=w168, "Movement Type (0: relative)"=w170, "Move Distance (0)"=w164, "error in (no error)"=w153, "Device and Axis"=w166, "Microstep Size (0)"=w167, "VISA resource name"=w155) -> ("error out"=w169:errorcluster)  [unwired: 3 in, 1 out]
                n87 = local write "ZaberError"(w169) -> ()
              }
            }
          }
          frame #2 {
            w173 = 1 ("index")
            n88 = Index Array(array=w172, index=w173) -> (element=w171:bool)
            n89 = case shown="True" w171 {
              tunnel: w176 -> [_ w191]
              tunnel: w175 -> [_ w188]
              tunnel: w174 -> [_ w190]
              tunnel: w173 -> [_ w189]
              frame False {
              }
              frame True {
                w178 = u16 2 items=["device units", "microns/s^2", "mm/s^2", "inches/s^2", "degrees/s^2"] ("Units (0: data)")
                w186 = u16 2 items=["device speed units", "microns per second", "millimeters per second", "inches per second", "degrees per second"] ("Units (0: device speed units)")
                w196 = u16 2 items=["microsteps", "microns", "millimeters", "inches", "degrees"] ("Units (0: microsteps)")
                w198 = u16 1 items=["relative", "absolute"] ("Movement Type (0: relative)")
                # "move to point command"
                n90 = Index Array(array=w191, index=w189) -> (element=w193:cluster{"Microstep Size":dbl, "Device":string})
                n91 = Index Array(array=w190, index=w189) -> (element=w192:dbl)
                n92 = local read "ZaberError"() -> (w187:errorcluster)
                n93 = local read "XY Speed\n[mm/s]"() -> (w185:dbl)
                n94 = local read "Acceleration [mm/s^2]"() -> (w177:dbl)
                n95 = Unbundle(w193) -> ("Microstep Size"=w180:dbl, "Device"=w179:string)
                n96 = call "Set Speed.vi"("Units (0: data)"=w186, "New Speed"=w185, "error in (no error)"=w187, "Device and Axis"=w179, "Microstep Size (0)"=w180, "VISA resource name"=w188) -> ("error out"=w184:errorcluster, "VISA resource name out"=w182:refnum<visa-resource-name>)  [unwired: 4 in]
                n97 = call "Set Acceleration.vi"("Units (0: data)"=w178, "New Acceleration"=w177, "error in (no error)"=w184, "Device and Axis"=w179, "Microstep Size (0)"=w180, "VISA resource name"=w182) -> ("error out"=w183:errorcluster, "VISA resource name out"=w181:refnum<visa-resource-name>)  [unwired: 4 in]
                n98 = Unbundle(w193) -> ("Microstep Size"=w195:dbl, "Device"=w194:string)
                n99 = call "Move.vi"("Units (0: microsteps)"=w196, "Movement Type (0: relative)"=w198, "Move Distance (0)"=w192, "error in (no error)"=w183, "Device and Axis"=w194, "Microstep Size (0)"=w195, "VISA resource name"=w181) -> ("error out"=w197:errorcluster)  [unwired: 3 in, 1 out]
                n100 = local write "ZaberError"(w197) -> ()
              }
            }
          }
          frame #3 {
            w201 = 2 ("index")
            n101 = Index Array(array=w200, index=w201) -> (element=w199:bool)
            n102 = case shown="True" w199 {
              tunnel: w204 -> [_ w219]
              tunnel: w203 -> [_ w213]
              tunnel: w202 -> [_ w218]
              tunnel: w201 -> [_ w217]
              frame False {
              }
              frame True {
                w212 = u16 2 items=["device units", "microns/s^2", "mm/s^2", "inches/s^2", "degrees/s^2"] ("Units (0: data)")
                w215 = u16 2 items=["device speed units", "microns per second", "millimeters per second", "inches per second", "degrees per second"] ("Units (0: device speed units)")
                w224 = u16 2 items=["microsteps", "microns", "millimeters", "inches", "degrees"] ("Units (0: microsteps)")
                w226 = u16 1 items=["relative", "absolute"] ("Movement Type (0: relative)")
                # "move to point command"
                n103 = Index Array(array=w219, index=w217) -> (element=w221:cluster{"Microstep Size":dbl, "Device":string})
                n104 = Index Array(array=w218, index=w217) -> (element=w220:dbl)
                n105 = local read "ZaberError"() -> (w216:errorcluster)
                n106 = local read "Speed Z [mm/s]"() -> (w214:dbl)
                n107 = Unbundle(w221) -> ("Microstep Size"=w210:dbl, "Device"=w211:string)
                n108 = local read "Acceleration [mm/s^2]"() -> (w205:dbl)
                n109 = call "Set Speed.vi"("Units (0: data)"=w215, "New Speed"=w214, "error in (no error)"=w216, "Device and Axis"=w211, "Microstep Size (0)"=w210, "VISA resource name"=w213) -> ("error out"=w207:errorcluster, "VISA resource name out"=w209:refnum<visa-resource-name>)  [unwired: 4 in]
                n110 = call "Set Acceleration.vi"("Units (0: data)"=w212, "New Acceleration"=w205, "error in (no error)"=w207, "Device and Axis"=w211, "Microstep Size (0)"=w210, "VISA resource name"=w209) -> ("error out"=w206:errorcluster, "VISA resource name out"=w208:refnum<visa-resource-name>)  [unwired: 4 in]
                n111 = Unbundle(w221) -> ("Microstep Size"=w223:dbl, "Device"=w222:string)
                n112 = call "Move.vi"("Units (0: microsteps)"=w224, "Movement Type (0: relative)"=w226, "Move Distance (0)"=w220, "error in (no error)"=w206, "Device and Axis"=w222, "Microstep Size (0)"=w223, "VISA resource name"=w208) -> ("error out"=w225:errorcluster)  [unwired: 3 in, 1 out]
                n113 = local write "ZaberError"(w225) -> ()
              }
            }
          }
          frame #4 {
            n114 = Tick Count (ms)() -> (millisecond timer value=w229:u32)
            n115 = while {
              tunnel: w231 -> [w250]
              tunnel: w230 -> [w246]
              shift-right: [w234] -> _
              shift-left: w229 -> [w235]
              tunnel: [w233] -> w228 mode=indexing
              tunnel: w227 -> [_]
              stop <- w236 stop-if-true
              w244 = 2 ("index")
              w242 = 1 ("index")
              w241 = 0 ("index")
              w261 = u16 2 items=["microsteps", "microns", "millimeters", "inches"] ("Units (0: microsteps)")
              n116 = Tick Count (ms)() -> (millisecond timer value=w234:u32)
              n117 = local read "Assignment"() -> (w262:cluster{"Microstep Size":dbl, "Device":string}[])
              n118 = local read "ZaberError"() -> (w252:errorcluster)
              n119 = local read "Port"() -> (w251:refnum<visa-resource-name>)
              n120 = Subtract(x=w234, y=w235) -> (x-y=w233:u32)
              n121 = Index Array(array=w262, index=0) -> (element=w263:cluster{"Microstep Size":dbl, "Device":string})
              n122 = Index Array(array=w262, index=1) -> (element=w264:cluster{"Microstep Size":dbl, "Device":string})
              n123 = Index Array(array=w262, index=2) -> (element=w265:cluster{"Microstep Size":dbl, "Device":string})
              n124 = Index Array(array=w246, index=w241) -> (element=w240:dbl)
              n125 = Index Array(array=w250, index=w241) -> (element=w247:bool)
              n126 = case shown="True" w247 {
                tunnel: w263 -> [_ w278]
                tunnel: w261 -> [_ w277]
                tunnel: [w268 w276] -> w254
                tunnel: [w267 w275] -> w253
                tunnel: w252 -> [w267 w274]
                tunnel: w251 -> [w268 w273]
                tunnel: w240 -> [_ w271]
                tunnel: [TRUE w269] -> w237
                tunnel: "Precision [mm]" -> [_ w270]
                frame False {
                }
                frame True {
                  n127 = Unbundle(w278) -> ("Microstep Size"=w279:dbl, "Device"=w280:string)
                  n128 = call "Read Current Position.vi"("Units (0: microsteps)"=w277, "error in (no error)"=w274, "Device and Axis"=w280, "Microstep Size (0)"=w279, "VISA resource name"=w273) -> ("error out"=w275:errorcluster, "Position"=w272:dbl, "VISA resource name out"=w276:refnum<visa-resource-name>)  [unwired: 4 in]
                  n129 = call "ChkOnTarget.vi"("Prec"=w270, "TargetPos"=w271, "CurrPos"=w272) -> ("In Range?"=w269:bool)
                }
              }
              n130 = Index Array(array=w250, index=w242) -> (element=w248:bool)
              n131 = Index Array(array=w246, index=w242) -> (element=w243:dbl)
              n132 = case shown="False" w248 {
                tunnel: w264 -> [_ w294]
                tunnel: w261 -> [_ w292]
                tunnel: [w283 w291] -> w256
                tunnel: [w282 w290] -> w255
                tunnel: w254 -> [w283 w289]
                tunnel: w253 -> [w282 w288]
                tunnel: w243 -> [_ w287]
                tunnel: [TRUE w284] -> w238
                tunnel: "Precision [mm]" -> [_ w285]
                frame False {
                }
                frame True {
                  n133 = Unbundle(w294) -> ("Microstep Size"=w293:dbl, "Device"=w295:string)
                  n134 = call "Read Current Position.vi"("Units (0: microsteps)"=w292, "error in (no error)"=w288, "Device and Axis"=w295, "Microstep Size (0)"=w293, "VISA resource name"=w289) -> ("error out"=w290:errorcluster, "Position"=w286:dbl, "VISA resource name out"=w291:refnum<visa-resource-name>)  [unwired: 4 in]
                  n135 = call "ChkOnTarget.vi"("Prec"=w285, "TargetPos"=w287, "CurrPos"=w286) -> ("In Range?"=w284:bool)
                }
              }
              n136 = Index Array(array=w246, index=w244) -> (element=w245:dbl)
              n137 = Index Array(array=w250, index=w244) -> (element=w249:bool)
              n138 = case shown="False" w249 {
                tunnel: w265 -> [_ w308]
                tunnel: w261 -> [_ w305]
                tunnel: [w297 w304] -> w257
                tunnel: w256 -> [_ w303]
                tunnel: w255 -> [w297 w302]
                tunnel: w245 -> [_ w300]
                tunnel: [TRUE w298] -> w239
                tunnel: "Precision [mm]" -> [_ w299]
                frame False {
                }
                frame True {
                  n139 = Unbundle(w308) -> ("Microstep Size"=w306:dbl, "Device"=w307:string)
                  n140 = call "Read Current Position.vi"("Units (0: microsteps)"=w305, "error in (no error)"=w302, "Device and Axis"=w307, "Microstep Size (0)"=w306, "VISA resource name"=w303) -> ("error out"=w304:errorcluster, "Position"=w301:dbl)  [unwired: 4 in, 1 out]
                  n141 = call "ChkOnTarget.vi"("Prec"=w299, "TargetPos"=w300, "CurrPos"=w301) -> ("In Range?"=w298:bool)
                }
              }
              n142 = local write "ZaberError"(w257) -> ()
              n143 = Compound Arithmetic op=AND(w239, w238, w237) -> (w236:bool)
            }
            "ReadoutTiming" <- w228
          }
          frame #5 {
            n144 = Tick Count (ms)() -> (millisecond timer value=w322:u32)
            n145 = Subtract(x=w322, y=w321) -> (x-y=w315:u32)
            "last point movement duration [ms]" <- w315
            n146 = local read "Data folder path"() -> (w313:path)
            n147 = Build Path(base path=w313, name or relative path="ZaberTiming.csv") -> (appended path=w309:path)
            n148 = local read "Data folder path"() -> (w317:path)
            n149 = Build Array(w315) -> (w314:u32[])
            n150 = Build Path(base path=w317, name or relative path="Timing.csv") -> (appended path=w316:path)
            n151 = call-poly <vilib>:"Write Delimited Spreadsheet.vi"("file path (dialog if empty)"=w309, "1D data"=w323, "append to file? (F)"=TRUE, "delimiter (\\t)"="\r") -> ()  [unwired: 10 in, 2 out]
            n152 = call-poly <vilib>:"Write Delimited Spreadsheet.vi"("file path (dialog if empty)"=w316, "1D data"=w314, "append to file? (F)"=TRUE, "delimiter (\\t)"="\r") -> ()  [unwired: 10 in, 2 out]
          }
        }
      }
      frame "DisplayData" {
        # "build all RIO maps\ndisplay left and right maps\n\nif scan finished:\nsave all maps in text files \nchange map mode flag to FALSE"
        n153 = local read "MAP"() -> (w325:bool)
        n154 = stacked-sequence {
          seq-local: [_ _ w483 _ _] -> [_ _ _ w490 w543]
          tunnel: w325 -> [w328 _ _ w489 _]
          frame #0 {
            n155 = case shown="True" w328 {
              frame False {
                n156 = local read "3D"() -> (w329:bool)
                n157 = case shown="True" w329 {
                  frame False {
                    n158 = local read "ROI_Array"() -> (w333:T7)
                    n159 = local read "LastSpectra"() -> (w334:u32[])
                    n160 = local read "1DSet"() -> (w332:dbl[][])
                    n161 = local read "current point"() -> (w331:i32)
                    n162 = for {
                      tunnel: w333 -> [w346] mode=indexing
                      tunnel: w334 -> [w345]
                      tunnel: w332 -> [w340] mode=indexing
                      tunnel: [w339] -> w330 mode=indexing
                      tunnel: w331 -> [w336]
                      n163 = Unbundle By Name(w346) -> ("ROI begin channel"=w343:T6, "ROI end channel"=w344:T6)
                      n164 = Subtract(x=w344, y=w343) -> (x-y=w342:T6)
                      n165 = local read "Live Time [s]"() -> (w337:dbl)
                      n166 = Array Subset(array=w345, index=w343, length=w342) -> (w341:u32[])
                      n167 = Add Array Elements(numeric array=w341) -> (sum=w338:u32)
                      n168 = Divide(x=w338, y=w337) -> (x/y=w335:dbl)
                      n169 = Replace Array Subset(array=w340, new element=w335, index=w336) -> (w339:dbl[])
                    }
                    n170 = local write "1DSet"(w330) -> ()
                  }
                  frame True {
                    n171 = stacked-sequence {
                      seq-local: [w354 _ _] -> [_ w376 _]
                      seq-local: [w350 _ _] -> [_ w379 _]
                      seq-local: [_ w378 _] -> [_ _ w382]
                      seq-local: [_ w371 _] -> [_ _ w381]
                      frame #0 {
                        n172 = local read "ROI_Array"() -> (w358:T7)
                        n173 = local read "LastSpectra"() -> (w357:u32[])
                        n174 = local read "current point"() -> (w356:i32)
                        n175 = local read "Z steps"() -> (w355:i32)
                        n176 = local read "1DSet"() -> (w349:dbl[][])
                        n177 = Quotient & Remainder(x=w356, y=w355) -> (x-y*floor(x/y)=w353:i32, floor(x/y)=w354:i32)
                        n178 = local read "init1Dset"() -> (w347:dbl[][])
                        n179 = Equal To 0?(x=w353) -> (x = 0?=w350:bool)
                        n180 = Select(t=w347, s=w350, f=w349) -> (s? t:f=w348:dbl[][])
                        n181 = for {
                          tunnel: w358 -> [w370] mode=indexing
                          tunnel: w357 -> [w369]
                          tunnel: w348 -> [w364] mode=indexing
                          tunnel: [w363] -> w351 mode=indexing
                          tunnel: w353 -> [w360]
                          tunnel: [w359] -> w352 mode=indexing
                          n182 = Unbundle By Name(w370) -> ("ROI begin channel"=w367:T6, "ROI end channel"=w368:T6)
                          n183 = Subtract(x=w368, y=w367) -> (x-y=w366:T6)
                          n184 = local read "Live Time [s]"() -> (w361:dbl)
                          n185 = Array Subset(array=w369, index=w367, length=w366) -> (w365:u32[])
                          n186 = Add Array Elements(numeric array=w365) -> (sum=w362:u32)
                          n187 = Divide(x=w362, y=w361) -> (x/y=w359:dbl)
                          n188 = Replace Array Subset(array=w364, new element=w359, index=w360) -> (w363:dbl[])
                        }
                        "Array" <- w352
                        n189 = local write "1DSet"(w351) -> ()
                      }
                      frame #1 {
                        n190 = Greater Than 0?(x=w376) -> (x > 0?=w380:bool)
                        n191 = And(x=w380, y=w379) -> (x .and. y?=w378:bool)
                        n192 = Number To Decimal String(number=w376) -> (decimal integer string=w374:string)  [unwired: 1 in]
                        n193 = local read "maps folder"() -> (w377:path)
                        n194 = Concatenate Strings("line_" ("name or relative path"), w374, ".csv" ("string")) -> (w372:string)
                        n195 = Build Path(base path=w377, name or relative path=w372) -> (appended path=w371:path)
                        "appended path" <- w371
                        "Numeric" <- w376
                      }
                      frame #2 {
                        n196 = case shown="True" w382 {
                          tunnel: w381 -> [_ w383]
                          frame False {
                          }
                          frame True {
                            n197 = local read "1DPosArray"() -> (w384:dbl[])
                            n198 = property on="MAP-L" class="Ring (strict)"() -> ("Strings []"=w390:string[])  [unwired: 2 in, 2 out]
                            n199 = local read "1DSet"() -> (w385:dbl[][])
                            n200 = Build Array (concatenate)(w384, w385) -> (w386:dbl[][])
                            n201 = Number To Fractional String(number=w386) -> (F-format string=w387:string[][])  [unwired: 3 in]
                            n202 = Build Array (concatenate)("position", w390) -> (w391:string[])
                            n203 = Transpose 2D Array(2D array=w387) -> (transposed array=w388:string[][])
                            n204 = Build Array (concatenate)(w391, w388) -> (w393:string[][])
                            n205 = for {
                              tunnel: w393 -> [w396] mode=indexing
                              tunnel: [w395] -> w394 mode=indexing
                              n206 = for {
                                tunnel: w396 -> [w400] mode=indexing
                                tunnel: [w397] -> w395 mode=indexing
                                n207 = Search and Replace String(input string=w400, search string=",", replace string="." ("replace string (\"\")")) -> (result string=w397:string)  [unwired: 5 in, 3 out]
                              }
                            }
                            n208 = call-poly <vilib>:"Write To Spreadsheet File.vi"("delimiter (\\t)"="," ("delimiter (\\t)"), "2D data"=w394, "file path (dialog if empty)"=w383) -> ()  [unwired: 5 in, 1 out]
                          }
                        }
                      }
                    }
                  }
                }
              }
              frame True {
                n209 = local read "ScanData"() -> (w426:T12)
                n210 = Unbundle By Name(w426) -> ("Order"=w401:u16, "ScanCoords [mm].X abs start"=w419:dbl, "ScanCoords [mm].X step"=w418:dbl, "ScanCoords [mm].Y abs start"=w416:dbl, "ScanCoords [mm].Y step"=w417:dbl, "ScanCoords [mm].Z abs start"=w414:dbl, "ScanCoords [mm].Z step"=w415:dbl)
                n211 = local read "Z [mm]"() -> (w402:dbl)
                n212 = local read "X [mm]"() -> (w404:dbl)
                n213 = local read "Y [mm]"() -> (w403:dbl)
                n214 = Subtract(x=w402, y=w414) -> (x-y=w422:dbl)
                n215 = Subtract(x=w403, y=w416) -> (x-y=w421:dbl)
                n216 = Subtract(x=w404, y=w419) -> (x-y=w420:dbl)
                n217 = Divide(x=w422, y=w415) -> (x/y=w425:dbl)
                n218 = Divide(x=w421, y=w417) -> (x/y=w424:dbl)
                n219 = Divide(x=w420, y=w418) -> (x/y=w423:dbl)
                n220 = case shown="6" w401 {
                  tunnel: w423 -> [w441 w443 w445 _ _ w451]
                  tunnel: w424 -> [w440 w442 _ w447 w449 _]
                  tunnel: w425 -> [_ _ w444 w446 w448 w450]
                  tunnel: [w441 w443 w445 w447 w449 w451] -> w413
                  tunnel: [w440 w442 w444 w446 w448 w450] -> w412
                  frame 1, Default {
                  }
                  frame 2 {
                  }
                  frame 3 {
                  }
                  frame 4 {
                  }
                  frame 5 {
                  }
                  frame 6 {
                  }
                }
                n221 = To Long Integer(number=w413) -> (32bit integer=w407:i32)
                n222 = To Long Integer(number=w412) -> (32bit integer=w408:i32)
                n223 = local read "LastSpectra"() -> (w411:u32[])
                n224 = local read "ROI_Array"() -> (w410:T7)
                n225 = local read "2DSet"() -> (w409:dbl[][][])
                n226 = for {
                  tunnel: w410 -> [w439] mode=indexing
                  tunnel: w411 -> [w438]
                  tunnel: w409 -> [w431] mode=indexing
                  tunnel: w408 -> [w433]
                  tunnel: w407 -> [w432]
                  tunnel: [w430] -> w406 mode=indexing
                  tunnel: [w427] -> w405 mode=indexing
                  n227 = Unbundle By Name(w439) -> ("ROI begin channel"=w436:T6, "ROI end channel"=w437:T6)
                  n228 = Subtract(x=w437, y=w436) -> (x-y=w435:T6)
                  n229 = local read "Live Time [s]"() -> (w428:dbl)
                  n230 = Array Subset(array=w438, index=w436, length=w435) -> (w434:u32[])
                  n231 = Add Array Elements(numeric array=w434) -> (sum=w429:u32)
                  n232 = Divide(x=w429, y=w428) -> (x/y=w427:dbl)
                  n233 = Replace Array Subset(array=w431, new element=w427, index (row)=w432, index (col)=w433) -> (w430:dbl[][])
                }
                "roi intensities 2d" <- w405
                n234 = local write "2DSet"(w406) -> ()
              }
            }
          }
          frame #1 {
            n235 = local read "MAP-R"() -> (w453:u16)
            n236 = local read "MAP-L"() -> (w454:u16)
            n237 = local read "MAP"() -> (w452:bool)
            n238 = case shown="True" w452 {
              tunnel: w454 -> [w458 w472]
              tunnel: w453 -> [w457 w470]
              frame False {
                n239 = local read "1DSet"() -> (w459:dbl[][])
                n240 = for {
                  tunnel: w459 -> [w464] mode=indexing
                  tunnel: w458 -> [w466]
                  tunnel: [w464] -> w456
                  i -> [w467]
                  stop <- w465 stop-if-true
                  n241 = Equal?(x=w466, y=w467) -> (x = y?=w465:bool)
                }
                n242 = for {
                  tunnel: w459 -> [w460] mode=indexing
                  tunnel: w457 -> [w462]
                  tunnel: [w460] -> w455
                  i -> [w463]
                  stop <- w461 stop-if-true
                  n243 = Equal?(x=w462, y=w463) -> (x = y?=w461:bool)
                }
                n244 = local write "1D graph 2"(w455) -> ()
                n245 = local write "1D graph 1"(w456) -> ()
              }
              frame True {
                n246 = local read "2DSet"() -> (w473:dbl[][][])
                n247 = local read "2DSet"() -> (w471:dbl[][][])
                n248 = for {
                  tunnel: w473 -> [w478] mode=indexing
                  tunnel: w472 -> [w480]
                  tunnel: [w478] -> w469
                  i -> [w481]
                  stop <- w479 stop-if-true
                  n249 = Equal?(x=w480, y=w481) -> (x = y?=w479:bool)
                }
                n250 = for {
                  tunnel: w471 -> [w474] mode=indexing
                  tunnel: w470 -> [w476]
                  tunnel: [w474] -> w468
                  i -> [w477]
                  stop <- w475 stop-if-true
                  n251 = Equal?(x=w476, y=w477) -> (x = y?=w475:bool)
                }
                n252 = local write "2D graph 2"(w468) -> ()
                n253 = local write "2D graph 1"(w469) -> ()
              }
            }
          }
          frame #2 {
            # "detection of last scan point or user stop"
            n254 = local read "current point"() -> (w486:i32)
            n255 = local read "/"() -> (w487:i32)
            n256 = Increment(x=w486) -> (x+1=w485:i32)
            n257 = Equal?(x=w485, y=w487) -> (x = y?=w482:bool)
            n258 = Or(x=w482, y="Stop Button") -> (x .or. y?=w483:bool)
            n259 = local write "current point"(w485) -> ()
          }
          frame #3 {
            n260 = local read "3D"() -> (w488:bool)
            n261 = case shown="True" w490 {
              tunnel: w489 -> [_ w492]
              tunnel: w488 -> [_ w491]
              frame False {
              }
              frame True {
                # "Map finished"
                n262 = stacked-sequence {
                  tunnel: w492 -> [w495 _]
                  tunnel: w491 -> [w493 _]
                  frame #0 {
                    n263 = local read "maps folder"() -> (w494:path)
                    n264 = case shown="False" w495 {
                      tunnel: w494 -> [w519 w526]
                      tunnel: w493 -> [w496 _]
                      frame False {
                        # "saving 1D data"
                        n265 = local read "1DPosArray"() -> (w518:dbl[])
                        n266 = property on="MAP-L" class="Ring (strict)"() -> ("Strings []"=w511:string[])  [unwired: 2 in, 2 out]
                        n267 = local read "1DSet"() -> (w517:dbl[][])
                        n268 = local read "Z steps"() -> (w501:i32)
                        n269 = local read "/"() -> (w500:i32)
                        n270 = Build Array (concatenate)(w518, w517) -> (w516:dbl[][])
                        n271 = Build Array (concatenate)("position", w511) -> (w510:string[])
                        n272 = Number To Fractional String(number=w516) -> (F-format string=w515:string[][])  [unwired: 3 in]
                        n273 = Divide(x=w500, y=w501) -> (x/y=w505:dbl)
                        n274 = To Word Integer(number=w505) -> (16bit integer=w506:i16)
                        n275 = Transpose 2D Array(2D array=w515) -> (transposed array=w514:string[][])
                        n276 = Number To Decimal String(number=w506) -> (decimal integer string=w503:string)  [unwired: 1 in]
                        n277 = Build Array (concatenate)(w510, w514) -> (w508:string[][])
                        n278 = for {
                          tunnel: w508 -> [w521] mode=indexing
                          tunnel: [w520] -> w507 mode=indexing
                          n279 = for {
                            tunnel: w521 -> [w525] mode=indexing
                            tunnel: [w522] -> w520 mode=indexing
                            n280 = Search and Replace String(input string=w525, search string=",", replace string="." ("replace string (\"\")")) -> (result string=w522:string)  [unwired: 5 in, 3 out]
                          }
                        }
                        n281 = Concatenate Strings("line_" ("name or relative path"), w503, ".csv" ("string")) -> (w497:string)
                        n282 = Select(t=w497, s=w496, f="result.csv" ("name or relative path")) -> (s? t:f=w498:string)
                        n283 = Build Path(base path=w519, name or relative path=w498) -> (appended path=w513:path)
                        n284 = call-poly <vilib>:"Write To Spreadsheet File.vi"("delimiter (\\t)"="," ("delimiter (\\t)"), "2D data"=w507, "file path (dialog if empty)"=w513) -> ()  [unwired: 5 in, 1 out]
                      }
                      frame True {
                        # "saving 2D data"
                        n285 = local read "2DSet"() -> (w528:dbl[][][])
                        n286 = property on="MAP-L" class="Ring (strict)"() -> ("Strings []"=w527:string[])  [unwired: 2 in, 2 out]
                        n287 = for {
                          tunnel: w528 -> [w534] mode=indexing
                          tunnel: w527 -> [w533] mode=indexing
                          tunnel: w526 -> [w529]
                          n288 = Concatenate Strings(w533, ".dat" ("string")) -> (w531:string)
                          n289 = Build Path(base path=w529, name or relative path=w531) -> (appended path=w530:path)
                          n290 = call-poly <vilib>:"Write To Spreadsheet File.vi"("2D data"=w534, "file path (dialog if empty)"=w530) -> ()  [unwired: 6 in, 1 out]
                        }
                      }
                    }
                  }
                  frame #1 {
                    n291 = local read "queue mode"() -> (w535:bool)
                    n292 = local write "scan mode"(FALSE ("map mode")) -> ()
                    n293 = case shown="True" w535 {
                      frame False {
                      }
                      frame True {
                        n294 = local read "ScanQueue"() -> (w542:T11)
                        n295 = Delete From Array(array=w542, length=1, index=0) -> (array with subset deleted=w539:T11)  [unwired: 1 out]
                        n296 = local write "ScanQueue"(w539) -> ()
                        n297 = Array Size(array=w539) -> (size(s)=w538:i32)
                        n298 = Greater Than 0?(x=w538) -> (x > 0?=w537:bool)
                        n299 = local write "queue mode"(w537) -> ()
                      }
                    }
                  }
                }
              }
            }
          }
          frame #4 {
            n300 = case shown="True" w543 {
              frame False {
              }
              frame True {
                n301 = flat-sequence {
                  frame #0 {
                    n302 = local read "Cumul. LT[s]"() -> (w544:dbl)
                    n303 = local read "spectra folder"() -> (w548:path)
                    n304 = local read "SumSpectra"() -> (w546:u64[])
                    n305 = call "SaveSpe.vi"("Live Time"=w544, "Real Time"=0.0, "Spectrum"=w546, "name"="SumSpectra.spe", "data folder path"=w548) -> ()  [unwired: 3 in]
                  }
                  frame #1 {
                    w552 = 0.0 ("Real Time")
                    n306 = local read "spectra folder"() -> (w549:path)
                    n307 = local read "MaxSpectra"() -> (w551:u64[])
                    n308 = call "SaveSpe.vi"("Live Time"=w552, "Real Time"=w552, "Spectrum"=w551, "name"="MaxSpectra.spe", "data folder path"=w549) -> ()  [unwired: 3 in]
                  }
                }
              }
            }
          }
        }
      }
      frame "SaveSpectra" {
        n309 = stacked-sequence {
          frame #0 {
            n310 = local read "scan mode"() -> (w564:bool)
            n311 = case shown="False" w564 {
              tunnel: [w570 w571] -> w563
              frame False {
                n312 = call "Spectrum name"() -> ("Name"=w570:string)  [unwired: 17 in, 2 out]
              }
              frame True {
                n313 = local read "current point"() -> (w581:i32)
                n314 = Increment(x=w581) -> (x+1=w572:i32)
                n315 = Number To Decimal String(number=w572, width (-)=i16 8) -> (decimal integer string=w575:string)
                n316 = call <vilib>:"Space Constant.vi"() -> ("String"=w576:string)
                n317 = Search and Replace String(replace all?=TRUE ("replace all? (F)"), input string=w575, search string=w576, replace string="0" ("replace string (\"\")"), error in=errorcluster {"status"=FALSE, "code"=0, "source"=""} ("error in (no error)")) -> (result string=w573:string)  [unwired: 3 in, 3 out]
                n318 = Concatenate Strings(w573, ".spe" ("string")) -> (w571:string)
              }
            }
            n319 = local read "Data folder path"() -> (w567:path)
            n320 = local read "spectra folder"() -> (w566:path)
            n321 = Select(t=w566, s=w564, f=w567) -> (s? t:f=w565:path)
            n322 = local read "Real Time [s]"() -> (w569:dbl)
            n323 = local read "Live Time [s]"() -> (w568:dbl)
            n324 = local read "LastSpectra"() -> (w562:u32[])
            n325 = local read "X [mm]"() -> (w561:dbl)
            n326 = local read "Y [mm]"() -> (w560:dbl)
            n327 = local read "Z [mm]"() -> (w559:dbl)
            n328 = call "SaveSpe.vi"("Live Time"=w568, "Z"=w559, "Y"=w560, "X"=w561, "Real Time"=w569, "Spectrum"=w562, "name"=w563, "data folder path"=w565) -> ()
          }
          frame #1 {
            n329 = local read "SpectrumType"() -> (w583:u16)
            n330 = case shown="2" w583 {
              tunnel: [w584 w585 w586] -> w582
              frame 0, Default {
                n331 = local read "SumSpectra"() -> (w584:u64[])
              }
              frame 1 {
                n332 = local read "MaxSpectra"() -> (w585:u64[])
              }
              frame 2 {
                n333 = local read "LastSpectra"() -> (w586:u32[])
              }
            }
            n334 = local write "SpectraPlot"(w582) -> ()
          }
        }
        n335 = local read "scan mode"() -> (w554:bool)
        n336 = Select(t=AcquisitionModuleStates."DisplayData" ("Enum"), s=w554, f=AcquisitionModuleStates."IDLE" ("Enum")) -> (s? t:f=w556:T2)
      }
      frame "Acquire" {
        n337 = Tick Count (ms)() -> (millisecond timer value=w587:u32)
        n338 = stacked-sequence {
          seq-local: [w600 _] -> [_ w617]
          seq-local: [w592 _] -> [_ w616]
          tunnel: [_ w626] -> w589
          tunnel: w587 -> [w592 _]
          frame #0 {
            n339 = local read "Stop"() -> (w609:bool)
            n340 = local read "DPP Configuration"() -> (w593:T1)
            n341 = local read "Map points"() -> (w605:u32)
            n342 = local read "Acquisition mode"() -> (w610:u16)
            n343 = local read "identifier out"() -> (w611:string)
            n344 = local read "Acquisition time [s]"() -> (w606:fxp<+,64,32>)
            n345 = local read "Time per spectrum [ms]"() -> (w604:u32)
            n346 = control-ref of="LastSpectra"() -> (w599:refnum<vi>)
            n347 = control-ref of="SpectraPlot"() -> (w597:refnum<vi>)
            n348 = control-ref of="Waveform Graph"() -> (w603:refnum<vi>)
            n349 = global read "SpectraData2.vi" "Waveform Graph"() -> (w600:dbl[][])
            "Waveform Graph" <- w600
            n350 = control-ref of="Acq. in progress"() -> (w607:refnum<vi>)
            n351 = call "SingleSpectrum.vi"("identifier out"=w611, "Acquisition mode"=w610, "DPP Configuration"=w593, "Number of boards in chain"=u8 1, "Boards to configure"=u8 0, "Start acq"=TRUE, "Stop"=w609, "Map points"=w605, "Time per spectrum [ms]"=w604, "reference"=w607, "Acquisition time [s]"=w606, "Waveform Refnum"=w603, "LastSpectra Refnum"=w599, "SpectraPlot Refnum"=w597) -> ("Error code"=w594:i32)  [unwired: 3 in, 2 out]
            n352 = local write "Error code"(w594) -> ()
            n353 = control-ref of="Acq. in progress"() -> ()  [unwired: 1 out]
            n354 = Transpose 2D Array(2D array=w600) -> (transposed array=w591:dbl[][])
            n355 = Reshape Array(w591, 4096 ("dimension size")) -> (w601:dbl[])
            n356 = To Unsigned Long Integer(number=w601) -> (unsigned 32bit integer=w598:u32[])
            n357 = local write "SpectraPlot"(w598) -> ()
            n358 = local write "LastSpectra"(w598) -> ()
          }
          frame #1 {
            # "if not mapping plot last spectra on spectra plot"
            n359 = disable-structure shown="Enabled" {
              frame Disabled {
                n360 = local read "ScanData"() -> (w628:T12)
                n361 = local read "ROI_Array"() -> ()  [unwired: 1 out]
                n362 = Unbundle By Name(w628) -> ()  [unwired: 3 out]
              }
              frame Enabled {
              }
            }
            n363 = local read "scan mode"() -> (w622:bool)
            n364 = call "fakespectra_2.vi"("all rows"=w617, "LT preset"="Preset Time [s]") -> ("Waveform Graph"=w621:u32[], "LT out"=w618:dbl, "RT out"=→"Real Time [s]":dbl)
            "LastSpectra" <- w621
            "Live Time [s]" <- w618
            n365 = local read "Cumul. LT[s]"() -> (w619:dbl)
            n366 = case shown="True" w622 {
              tunnel: w621 -> [w629 w630]
              frame False {
                n367 = local write "SpectraPlot"(w629) -> ()
              }
              frame True {
                n368 = local read "MaxSpectra"() -> (w631:u64[])
                n369 = local read "SumSpectra"() -> (w633:u64[])
                n370 = for {
                  tunnel: w631 -> [w636] mode=indexing
                  tunnel: w630 -> [w637] mode=indexing
                  tunnel: [w635] -> w632 mode=indexing
                  n371 = Greater?(x=w637, y=w636) -> (0:w638:bool)
                  n372 = Select(t=w637, s=w638, f=w636) -> (s? t:f=w635:u64)
                }
                "MaxSpectra" <- w632
                n373 = Add(x=w630, y=w633) -> (x+y=→"SumSpectra":u64[])
              }
            }
            n374 = Add(x=w618, y=w619) -> (x+y=→"Cumul. LT[s]":dbl)
            n375 = Tick Count (ms)() -> (millisecond timer value=w615:u32)
            n376 = Subtract(x=w615, y=w616) -> (x-y=w614:u32)
            n377 = Select(t=AcquisitionModuleStates."SaveSpectra" ("Enum"), s=w622, f=AcquisitionModuleStates."IDLE" ("Enum")) -> (s? t:f=w626:T2)
            n378 = Divide(x=w614, y=u32 1000) -> (x/y=→"x/y":dbl)
          }
        }
      }
      frame "IDLE" {
        n379 = local read "Acquisition mode"() -> (w639:u16)
        n380 = event shown="[14] \"GoToX\": Value Change" {
          selector: _ -> [_ _ _ _ _ _ _ _ _ _ _ _ _ _ _ _ _ _ _ _ _ _ _ _ _ _ _ _ _ _ _ _ _ _ _ _ _ _ _ _ _ _ _ _ _ _ _]
          dyn-events: _ -> [_ _ _ _ _ _ _ _ _ _ _ _ _ _ _ _ _ _ _ _ _ _ _ _ _ _ _ _ _ _ _ _ _ _ _ _ _ _ _ _ _ _ _ _ _ _ _]
          timeout: w646 -> [_ _ _ _ _ _ _ _ _ _ _ _ _ _ _ _ _ _ _ _ _ _ _ _ _ _ _ _ _ _ _ _ _ _ _ _ _ _ _ _ _ _ _ _ _ _ _]
          tunnel: [FALSE ("VI stop") FALSE ("VI stop") FALSE ("VI stop") FALSE ("VI stop") FALSE ("VI stop") FALSE ("VI stop") FALSE ("VI stop") FALSE ("VI stop") FALSE ("VI stop") FALSE ("VI stop") FALSE ("VI stop") FALSE ("VI stop") FALSE ("VI stop") FALSE ("VI stop") FALSE ("VI stop") FALSE ("VI stop") FALSE ("VI stop") FALSE ("VI stop") FALSE ("VI stop") FALSE ("VI stop") FALSE ("VI stop") FALSE ("VI stop") FALSE ("VI stop") FALSE ("VI stop") FALSE ("VI stop") FALSE ("VI stop") FALSE ("VI stop") _ TRUE ("VI stop") _ FALSE ("VI stop") FALSE ("VI stop") FALSE ("VI stop") FALSE ("VI stop") FALSE ("VI stop") FALSE ("VI stop") FALSE ("VI stop") FALSE ("VI stop") FALSE ("VI stop") FALSE ("VI stop") FALSE ("VI stop") _ _ _ FALSE ("VI stop") FALSE ("VI stop") FALSE ("VI stop")] -> w645
          tunnel: [w651 w690 w697 w716 w732 w743 w756 w787 w828 w864 w898 w980 w1026 w1080 w1103 w1126 w1133 w1144 w1179 w1216 w1222 w1279 w1315 w1350 w1394 AcquisitionModuleStates."PrepareMap" ("Enum") w1417 AcquisitionModuleStates."SaveSpectra" ("Enum") AcquisitionModuleStates."Close" ("Enum") w1441 w1449 w1541 w1559 w1576 w1578 w1609 w1624 w1635 w1648 w1651 AcquisitionModuleStates."Acquire" ("Enum") w1684 w1689 w1696 w1704 w1745 w1749] -> w644
          tunnel: AcquisitionModuleStates."IDLE" ("Enum") -> [_ w690 w697 w716 w732 w743 w756 w787 w828 w864 _ _ w1026 w1080 w1103 w1126 w1133 w1144 w1179 w1216 w1222 w1279 w1315 w1350 w1394 _ w1417 _ _ w1441 w1449 w1541 w1559 w1576 w1578 w1609 w1624 w1635 w1648 w1651 _ w1684 w1689 w1696 w1704 w1745 w1749]
          tunnel: w642 -> [_ _ _ _ _ _ _ w764 w808 w851 _ _ _ _ _ _ _ _ _ _ _ _ _ _ _ _ _ _ _ _ _ _ _ _ _ _ _ _ _ _ _ _ _ _ _ _ _]
          tunnel: w641 -> [_ _ _ _ _ _ _ _ _ _ _ _ _ _ _ _ _ _ _ _ _ _ _ _ _ _ _ _ w1424 _ _ _ _ _ _ _ _ _ _ _ _ w1686 w1691 w1698 _ _ _]
          tunnel: [_ _ _ _ _ _ _ _ _ _ _ _ _ _ _ _ _ _ _ _ _ _ _ _ _ _ _ _ w1423 _ _ _ _ _ _ _ _ _ _ _ _ w1683 w1688 w1695 _ _ _] -> w640
          event Timeout {
            n381 = event-data() -> ()  [unwired: 1 in, 1 out]
            n382 = stacked-sequence {
              tunnel: [_ w688] -> w651
              frame #0 {
                w663 = u16 2 items=["microsteps", "microns", "millimeters", "inches"] ("Units (0: microsteps)")
                # "reading manipulator position"
                n383 = local read "Assignment"() -> (w662:cluster{"Microstep Size":dbl, "Device":string}[])
                n384 = local read "ZaberError"() -> (w675:errorcluster)
                n385 = local read "Port"() -> (w676:refnum<visa-resource-name>)
                n386 = Index Array(array=w662, index=0) -> (element=w661:cluster{"Microstep Size":dbl, "Device":string})
                n387 = Index Array(array=w662, index=1) -> (element=w657:cluster{"Microstep Size":dbl, "Device":string})
                n388 = Index Array(array=w662, index=2) -> (element=w653:cluster{"Microstep Size":dbl, "Device":string})
                n389 = Unbundle(w661) -> ("Microstep Size"=w660:dbl, "Device"=w659:string)
                n390 = call "Read Current Position.vi"("Units (0: microsteps)"=w663, "error in (no error)"=w675, "Device and Axis"=w659, "Microstep Size (0)"=w660, "VISA resource name"=w676) -> ("error out"=w674:errorcluster, "Position"=→"X [mm]":dbl, "VISA resource name out"=w673:refnum<visa-resource-name>)  [unwired: 4 in]
                n391 = Unbundle(w657) -> ("Microstep Size"=w658:dbl, "Device"=w656:string)
                n392 = call "Read Current Position.vi"("Units (0: microsteps)"=w663, "error in (no error)"=w674, "Device and Axis"=w656, "Microstep Size (0)"=w658, "VISA resource name"=w673) -> ("error out"=w672:errorcluster, "Position"=→"Y [mm]":dbl, "VISA resource name out"=w671:refnum<visa-resource-name>)  [unwired: 4 in]
                n393 = Unbundle(w653) -> ("Microstep Size"=w655:dbl, "Device"=w654:string)
                n394 = call "Read Current Position.vi"("Units (0: microsteps)"=w663, "error in (no error)"=w672, "Device and Axis"=w654, "Microstep Size (0)"=w655, "VISA resource name"=w671) -> ("error out"=w670:errorcluster, "Position"=→"Z [mm]":dbl)  [unwired: 4 in, 1 out]
                n395 = local write "ZaberError"(w670) -> ()
              }
              frame #1 {
                n396 = local read "scan mode"() -> (w677:bool)
                n397 = local read "queue mode"() -> (w679:bool)
                n398 = Select(t=T15."Disabled" ("Disabled"), s=w677, f=T15."Enabled" ("Disabled")) -> (s? t:f=w682:T15)
                n399 = property on="SpectrumType" class="Ring (strict)"("Visible"=w677) -> ()  [unwired: 2 in, 2 out]
                n400 = local write "QUICKSCAN_Start"(w677) -> ()
                n401 = property on="QUICKSCAN_Start" class="Bool (strict)"("DisabledEnum"=w682) -> ()  [unwired: 2 in, 2 out]
                n402 = local write "QUEUE_Run"(w679) -> ()
                n403 = Select(t=T15."Disabled" ("Disabled"), s=w679, f=T15."Enabled" ("Disabled")) -> (s? t:f=w678:T15)
                n404 = property on="Stop Button" class="Bool"("DisabledEnum"=w678) -> ()  [unwired: 2 in, 2 out]
                n405 = Select(t=AcquisitionModuleStates."PrepareMap" ("Enum"), s=w679, f=AcquisitionModuleStates."IDLE" ("Enum")) -> (s? t:f=w685:T2)
                n406 = Select(t=AcquisitionModuleStates."MoveToPoint" ("Enum"), s=w677, f=w685) -> (s? t:f=w688:T2)
              }
            }
          }
          event "Clear_Queue": Value Change {
            n407 = event-data() -> ()  [unwired: 1 in, 6 out]
            n408 = local read "ScanData"() -> (w693:T12)
            n409 = Initialize Array(w693) -> (w692:T21)  [unwired: 1 in]
            n410 = local write "ScanQueue"(w692) -> ()
          }
          event "Tab Control": Value Change {
            n411 = event-data() -> ("NewVal"=w696:T4)  [unwired: 1 in, 5 out]
            n412 = Equal?(x=w696, y=T4."Queue" ("NewVal")) -> (x = y?=w694:bool)
            n413 = case shown="True" w694 {
              frame False {
              }
              frame True {
                n414 = local read "ScanQueue"() -> (w703:T11)
                n415 = Array Size(array=w703) -> (size(s)=→"NoOfScans":i32)
                n416 = for {
                  tunnel: w703 -> [w714] mode=indexing
                  shift-right: [w711] -> w701
                  shift-left: 0 -> [w710]
                  tunnel: [w705] -> w699 mode=indexing
                  n417 = Unbundle By Name(w714) -> ("Name"=w705:string, "PresetVal"=w712:dbl, "#points"=w713:i32, "CtsPreset?"=w708:bool)
                  n418 = Not(x=w708) -> (.not. x?=w707:bool)
                  n419 = Boolean To (0,1)(Boolean=w707) -> (0, 1=w706:i16)
                  n420 = Compound Arithmetic op=MULTIPLY(w712, w713, w706) -> (w709:dbl)
                  n421 = Add(x=w709, y=w710) -> (x+y=w711:dbl)
                }
                n422 = property on="Text Ring" class="Ring (strict)"("Strings []"=w699) -> ()  [unwired: 2 in, 2 out]
                n423 = call "SecondsToTimeStamp.vi"("Time [s]"=w701) -> ("TimeStamp"=→"estimated duration":string)
              }
            }
          }
          event "Delete": Value Change {
            n424 = event-data() -> ()  [unwired: 1 in, 6 out]
            n425 = flat-sequence {
              frame #0 {
                n426 = local read "ScanQueue"() -> (w721:T11)
                n427 = Delete From Array(array=w721, length=1, index="Text Ring") -> (array with subset deleted=w718:T11)  [unwired: 1 out]
                n428 = for {
                  tunnel: w718 -> [w723] mode=indexing
                  tunnel: [w722] -> w717 mode=indexing
                  n429 = Unbundle By Name(w723) -> ("Name"=w722:string)
                }
                n430 = local write "ScanQueue"(w718) -> ()
                n431 = property on="Text Ring" class="Ring (strict)"("Strings []"=w717) -> ()  [unwired: 2 in, 2 out]
              }
              frame #1 {
                n432 = property on="Tab Control" class="TabCtl (strict)"("Val(Sgnl)"=T4."Queue" ("NewVal")) -> ()  [unwired: 2 in, 2 out]
                n433 = local write "Text Ring"(0) -> ()
              }
            }
          }
          event "QUEUE_Stop": Value Change {
            n434 = event-data() -> ()  [unwired: 1 in, 6 out]
            n435 = call <vilib>:"Three Button Dialog.vi"("Allow user to close window? (TRUE)"=FALSE, "Justify Message (Left)"=enum16{"Left", "Center", "Right"}."Center", "Window Title (\"\")"="Terminate queue" ("Window Title (\"\")"), "message"="Do you want to finish the ongoing scan?") -> ("Which Button?"=w728:T22)  [unwired: 7 in]
            n436 = case shown="\"Left Button\", Default" w728 {
              frame "Left Button", Default {
                # "finish scan"
                n437 = local write "queue mode"(FALSE ("scan mode")) -> ()
                n438 = local write "scan mode"(TRUE ("scan mode")) -> ()
              }
              frame "Center Button" {
                # "stop recent scan"
                n439 = local write "queue mode"(FALSE ("scan mode")) -> ()
                n440 = local write "scan mode"(FALSE ("scan mode")) -> ()
              }
              frame "Right Button" {
              }
              frame "Window Close" {
              }
            }
          }
          event "Scan definition by": Value Change {
            n441 = event-data() -> ("NewVal"=w742:T10)  [unwired: 1 in, 5 out]
            n442 = case shown="\"Scan boundaries and step size\"" w742 {
              tunnel: [w746 w748 w750] -> w740
              tunnel: T15."Enabled" ("Disabled") -> [w746 w747 w750]
              tunnel: [w746 w747 w749] -> w739
              tunnel: T15."Disabled and Grayed Out" ("Disabled") -> [w745 w748 w749]
              tunnel: [w745 w747 w750] -> w737
              frame "Step size and step number", Default {
              }
              frame "Scan boundaries and step size" {
              }
              frame "Scan boundaries and number of steps" {
              }
            }
            n443 = property on="X end [mm]" class="DigNum (strict)"("DisabledEnum"=w737) -> ()  [unwired: 2 in, 2 out]
            n444 = property on="Y end [mm]" class="DigNum (strict)"("DisabledEnum"=w737) -> ()  [unwired: 2 in, 2 out]
            n445 = property on="Z end [mm]" class="DigNum (strict)"("DisabledEnum"=w737) -> ()  [unwired: 2 in, 2 out]
            n446 = property on="X steps" class="DigNum (strict)"("DisabledEnum"=w740) -> ()  [unwired: 2 in, 2 out]
            n447 = property on="Y steps" class="DigNum (strict)"("DisabledEnum"=w740) -> ()  [unwired: 2 in, 2 out]
            n448 = property on="Z steps" class="DigNum (strict)"("DisabledEnum"=w740) -> ()  [unwired: 2 in, 2 out]
            n449 = property on="step X [mm]" class="DigNum (strict)"("DisabledEnum"=w739) -> ()  [unwired: 2 in, 2 out]
            n450 = property on="step Y [mm]" class="DigNum (strict)"("DisabledEnum"=w739) -> ()  [unwired: 2 in, 2 out]
            n451 = property on="step Z [mm]" class="DigNum (strict)"("DisabledEnum"=w739) -> ()  [unwired: 2 in, 2 out]
          }
          event "Preset type:": Value Change {
            n452 = event-data() -> ("NewVal"=w755:enum32{"Live time [s]", "Counts"})  [unwired: 1 in, 5 out]
            n453 = case shown="\"Live time [s]\", Default" w755 {
              tunnel: ["Time Preset [s]" ("Caption.Text") "Counts Preset [cts]" ("Caption.Text")] -> w754
              tunnel: [FALSE TRUE] -> w751
              frame "Live time [s]", Default {
              }
              frame "Counts" {
              }
            }
            n454 = local read "ROI_Array"() -> (w753:T7)
            n455 = for {
              tunnel: w753 -> [w759] mode=indexing
              tunnel: [w758] -> w752 mode=indexing
              n456 = Unbundle By Name(w759) -> ("ROI name"=w758:T5)
            }
            n457 = property on="PresetROI" class="Ring (strict)"("Visible"=w751) -> ()  [unwired: 2 in, 2 out]
            n458 = property on="PresetVal" class="DigNum (strict)"("Caption.Text"=w754) -> ()  [unwired: 2 in, 2 out]
            n459 = property on="PresetROI" class="Ring (strict)"("Strings []"=w752) -> ()  [unwired: 2 in, 2 out]
          }
          event "step X [mm]", "X steps", "X start [mm]", "X end [mm]": Value Change {
            n460 = event-data() -> ()  [unwired: 1 in, 6 out]
            n461 = local read "Scan definition by"() -> (w785:T10)
            n462 = Decrement(x="X steps") -> (x-1=w779:i32)
            n463 = case shown="\"Scan boundaries and step size\"" w785 {
              tunnel: "X start [mm]" -> [w791 w801 w807]
              tunnel: "step X [mm]" -> [w788 w795 _]
              tunnel: w779 -> [w789 _ w804]
              tunnel: [w790 w802 w803] -> w775
              tunnel: "X end [mm]" -> [_ w802 w803]
              tunnel: [w788 w799 w805] -> w766
              tunnel: [w789 w800 w804] -> w771
              frame "Step size and step number", Default {
                n464 = Multiply(x=w788, y=w789) -> (x*y=w792:dbl)
                n465 = Add(x=w791, y=w792) -> (x+y=w790:dbl)
              }
              frame "Scan boundaries and step size" {
                n466 = Subtract(x=w802, y=w801) -> (x-y=w796:dbl)
                n467 = call "quotient.vi"("Y"=w795, "X"=w796) -> ("s? t:f"=w793:dbl, "x = y?"=w794:bool)  [unwired: 1 in]
                n468 = Divide(x=w796, y=w793) -> (x/y=w798:dbl)
                n469 = Absolute Value(x=w793) -> (abs(x)=w797:dbl)
                n470 = Select(t=w795, s=w794, f=w798) -> (s? t:f=w799:dbl)
                n471 = To Long Integer(number=w797) -> (32bit integer=w800:i32)
              }
              frame "Scan boundaries and number of steps" {
                n472 = Subtract(x=w803, y=w807) -> (x-y=w806:dbl)
                n473 = Divide(x=w806, y=w804) -> (x/y=w805:dbl)
              }
            }
            n474 = Increment(x=w771) -> (x+1=w778:i32)
            n475 = local read "X [mm]"() -> (w776:dbl)
            n476 = Add(x=w776, y="X start [mm]") -> (x+y=w768:dbl)
            n477 = Add(x=w776, y=w775) -> (x+y=w767:dbl)
            n478 = Unbundle By Name(w764) -> ("X min"=w777:dbl, "X max"=w774:dbl)
            n479 = local read "Y steps"() -> (w783:i32)
            n480 = Less?(x=w768, y=w777) -> (x < y?=w772:bool)
            n481 = Greater?(x=w767, y=w774) -> (0:w773:bool)
            n482 = local read "Z steps"() -> (w782:i32)
            n483 = Or(x=w772, y=w773) -> (x .or. y?=→"X error":bool)
            n484 = local write "step X [mm]"(w766) -> ()
            n485 = local write "X end [mm]"(w775) -> ()
            n486 = local write "X steps"(w778) -> ()
            n487 = Compound Arithmetic op=MULTIPLY(w778, w783, w782) -> (→"total # of points":i32)
          }
          event "Y start [mm]", "Y end [mm]", "Y steps", "step Y [mm]": Value Change {
            n488 = event-data() -> ()  [unwired: 1 in, 6 out]
            n489 = local read "Scan definition by"() -> (w831:T10)
            n490 = Decrement(x="Y steps") -> (x-1=w825:i32)
            n491 = case shown="\"Scan boundaries and step size\"" w831 {
              tunnel: "Y start [mm]" -> [w835 w844 w850]
              tunnel: "step Y [mm]" -> [w832 w839 _]
              tunnel: w825 -> [w833 _ w847]
              tunnel: [w834 w845 w846] -> w815
              tunnel: "Y end [mm]" -> [_ w845 w846]
              tunnel: [w832 w842 w848] -> w809
              tunnel: [w833 w843 w847] -> w824
              frame "Step size and step number", Default {
                n492 = Multiply(x=w832, y=w833) -> (x*y=w836:dbl)
                n493 = Add(x=w835, y=w836) -> (x+y=w834:dbl)
              }
              frame "Scan boundaries and step size" {
                n494 = Subtract(x=w845, y=w844) -> (x-y=w840:dbl)
                n495 = call "quotient.vi"("Y"=w839, "X"=w840) -> ("s? t:f"=w837:dbl, "x = y?"=w838:bool)  [unwired: 1 in]
                n496 = Divide(x=w840, y=w837) -> (x/y=w841:dbl)
                n497 = Select(t=w839, s=w838, f=w841) -> (s? t:f=w842:dbl)
                n498 = To Long Integer(number=w837) -> (32bit integer=w843:i32)
              }
              frame "Scan boundaries and number of steps" {
                n499 = Subtract(x=w846, y=w850) -> (x-y=w849:dbl)
                n500 = Divide(x=w849, y=w847) -> (x/y=w848:dbl)
              }
            }
            n501 = local read "Y [mm]"() -> (w819:dbl)
            n502 = local write "Y end [mm]"(w815) -> ()
            n503 = local write "step Y [mm]"(w809) -> ()
            n504 = Increment(x=w824) -> (x+1=w823:i32)
            n505 = local read "X steps"() -> (w822:i32)
            n506 = local read "Z steps"() -> (w821:i32)
            n507 = Unbundle By Name(w808) -> ("Y min"=w814:dbl, "Y max"=w813:dbl)
            n508 = Add(x=w819, y="Y start [mm]") -> (x+y=w811:dbl)
            n509 = Add(x=w819, y=w815) -> (x+y=w810:dbl)
            n510 = local write "Y steps"(w823) -> ()
            n511 = Less?(x=w811, y=w814) -> (x < y?=w817:bool)
            n512 = Greater?(x=w810, y=w813) -> (0:w818:bool)
            n513 = Compound Arithmetic op=MULTIPLY(w823, w822, w821) -> (w820:i32)
            n514 = Or(x=w817, y=w818) -> (x .or. y?=→"Y error":bool)
            n515 = local write "total # of points"(w820) -> ()
          }
          event "Z steps", "Z end [mm]", "Z start [mm]", "step Z [mm]": Value Change {
            n516 = event-data() -> ()  [unwired: 1 in, 6 out]
            n517 = local read "Scan definition by"() -> (w865:T10)
            n518 = Decrement(x="Z steps") -> (x-1=w866:i32)
            n519 = case shown="\"Scan boundaries and step size\"" w865 {
              tunnel: "Z start [mm]" -> [w878 w887 w893]
              tunnel: "step Z [mm]" -> [w875 w882 _]
              tunnel: w866 -> [w876 _ w890]
              tunnel: [w877 w888 w889] -> w857
              tunnel: "Z end [mm]" -> [_ w888 w889]
              tunnel: [w875 w885 w891] -> w852
              tunnel: [w876 w886 w890] -> w867
              frame "Step size and step number", Default {
                n520 = Multiply(x=w875, y=w876) -> (x*y=w879:dbl)
                n521 = Add(x=w878, y=w879) -> (x+y=w877:dbl)
              }
              frame "Scan boundaries and step size" {
                n522 = Subtract(x=w888, y=w887) -> (x-y=w883:dbl)
                n523 = call "quotient.vi"("Y"=w882, "X"=w883) -> ("s? t:f"=w880:dbl, "x = y?"=w881:bool)  [unwired: 1 in]
                n524 = Divide(x=w883, y=w880) -> (x/y=w884:dbl)
                n525 = Select(t=w882, s=w881, f=w884) -> (s? t:f=w885:dbl)
                n526 = To Long Integer(number=w880) -> (32bit integer=w886:i32)
              }
              frame "Scan boundaries and number of steps" {
                n527 = Subtract(x=w889, y=w893) -> (x-y=w892:dbl)
                n528 = Divide(x=w892, y=w890) -> (x/y=w891:dbl)
              }
            }
            n529 = Increment(x=w867) -> (x+1=w872:i32)
            n530 = local write "Z end [mm]"(w857) -> ()
            n531 = local write "step Z [mm]"(w852) -> ()
            n532 = local read "Z [mm]"() -> (w858:dbl)
            n533 = local read "Y steps"() -> (w873:i32)
            n534 = local read "X steps"() -> (w874:i32)
            n535 = Unbundle By Name(w851) -> ("Z min"=w860:dbl, "Z max"=w859:dbl)
            n536 = Add(x=w858, y="Z start [mm]") -> (x+y=w854:dbl)
            n537 = Add(x=w858, y=w857) -> (x+y=w853:dbl)
            n538 = Less?(x=w854, y=w860) -> (x < y?=w861:bool)
            n539 = Greater?(x=w853, y=w859) -> (0:w862:bool)
            n540 = Compound Arithmetic op=MULTIPLY(w872, w873, w874) -> (w871:i32)
            n541 = Or(x=w861, y=w862) -> (x .or. y?=→"Z error":bool)
            n542 = local write "Z steps"(w872) -> ()
            n543 = local write "total # of points"(w871) -> ()
          }
          event "QUICKSCAN_Start", "Add To Queue": Value Change {
            n544 = event-data() -> ("CtlRef"=w897:refnum<vi>)  [unwired: 1 in, 5 out]
            n545 = local read "X error"() -> (w904:T9)
            n546 = local read "Y error"() -> (w903:T9)
            n547 = local read "Z error"() -> (w902:T9)
            n548 = property on="Add To Queue" class="Bool"() -> ("Label.Text"=w895:string)  [unwired: 2 in, 2 out]
            n549 = property class="Bool"(reference=w897) -> ("Label.Text"=w896:string)  [unwired: 1 in, 2 out]
            n550 = Not(x=w904) -> (.not. x?=w905:T9)
            n551 = Not(x=w903) -> (.not. x?=w901:T9)
            n552 = Not(x=w902) -> (.not. x?=w900:T9)
            n553 = Equal?(x=w896, y=w895) -> (x = y?=w894:bool)
            n554 = Compound Arithmetic op=AND(w905, w901, w900) -> (w899:T9)
            n555 = case shown="True" w899 {
              tunnel: [AcquisitionModuleStates."IDLE" ("Enum") w909] -> w898
              tunnel: w894 -> [_ w908]
              frame False {
              }
              frame True {
                n556 = stacked-sequence {
                  seq-local: [w915 _ _ _ _] -> [_ w919 _ _ _]
                  seq-local: [_ w918 _ _ _] -> [_ _ w927 _ _]
                  seq-local: [_ _ w926 _ _] -> [_ _ _ w944 _]
                  seq-local: [_ _ _ "PresetVal" _] -> [_ _ _ _ w949]
                  seq-local: [_ _ _ w942 _] -> [_ _ _ _ w948]
                  seq-local: [_ _ _ w935 _] -> [_ _ _ _ w946]
                  tunnel: [_ _ _ _ w950] -> w909
                  tunnel: w908 -> [_ _ _ _ w947]
                  frame #0 {
                    w917 = T20 {"X abs start"=0.0, "X abs end"=0.0, "Y abs start"=0.0, "Y abs end"=0.0, "Z abs start"=0.0, "Z abs end"=0.0, "X step"=0.0, "Y step"=0.0, "Z step"=0.0}  # ScanCoords [mm]
                    n557 = local read "X end [mm]"() -> (w911:dbl)
                    n558 = local read "X start [mm]"() -> (w914:dbl)
                    n559 = local read "X [mm]"() -> (w912:dbl)
                    n560 = Add(x=w912, y=w914) -> (x+y=w913:dbl)
                    n561 = Add(x=w912, y=w911) -> (x+y=w910:dbl)
                    n562 = local read "step X [mm]"() -> (w916:dbl)
                    n563 = Bundle By Name(cluster=w917, "X abs start"=w913, "X abs end"=w910, "X step"=w916) -> (w915:T20)
                  }
                  frame #1 {
                    n564 = local read "Y end [mm]"() -> (w921:dbl)
                    n565 = local read "Y start [mm]"() -> (w924:dbl)
                    n566 = local read "Y [mm]"() -> (w922:dbl)
                    n567 = Add(x=w922, y=w924) -> (x+y=w923:dbl)
                    n568 = Add(x=w922, y=w921) -> (x+y=w920:dbl)
                    n569 = local read "step Y [mm]"() -> (w925:dbl)
                    n570 = Bundle By Name(cluster=w919, "Y abs start"=w923, "Y abs end"=w920, "Y step"=w925) -> (w918:T20)
                  }
                  frame #2 {
                    n571 = local read "Z end [mm]"() -> (w929:dbl)
                    n572 = local read "Z start [mm]"() -> (w932:dbl)
                    n573 = local read "Z [mm]"() -> (w930:dbl)
                    n574 = Add(x=w930, y=w932) -> (x+y=w931:dbl)
                    n575 = Add(x=w930, y=w929) -> (x+y=w928:dbl)
                    n576 = local read "step Z [mm]"() -> (w933:dbl)
                    n577 = Bundle By Name(cluster=w927, "Z abs start"=w931, "Z abs end"=w928, "Z step"=w933) -> (w926:T20)
                  }
                  frame #3 {
                    n578 = local read "total # of points"() -> (w941:i32)
                    n579 = local read "Preset type:"() -> (w937:enum32{"Live time [s]", "Counts"})
                    n580 = Equal?(x=w937, y=enum32{"Live time [s]", "Charge [C]"}."Charge [C]" ("Preset type:")) -> (x = y?=w935:bool)
                    n581 = Bundle By Name(cluster=T16 {"ScanCoords [mm]"={"X abs start"=0.0, "X abs end"=0.0, "Y abs start"=0.0, "Y abs end"=0.0, "Z abs start"=0.0, "Z abs end"=0.0, "X step"=0.0, "Y step"=0.0, "Z step"=0.0}, "PresetVal"=0.0, "Order"=0, "Snake?"=TRUE, "Name"="", "#points"=0, "ChrgPreset?"=TRUE, "CtPrstROI"=0} ("input cluster"), "ScanCoords [mm]"=w944, "PresetVal"="PresetVal", "Order"="Scan order", "Snake?"="Snake?", "Name"="ScanName:", "#points"=w941, "ChrgPreset?"=w935, "CtPrstROI"="PresetROI") -> (w942:T16)
                  }
                  frame #4 {
                    n582 = case shown="False" w947 {
                      tunnel: [AcquisitionModuleStates."IDLE" ("Enum") w968] -> w950
                      tunnel: w949 -> [w955 w967]
                      tunnel: w948 -> [w952 w965]
                      tunnel: w946 -> [w951 w964]
                      frame True {
                        n583 = local read "total # of points"() -> (w959:i32)
                        n584 = call "ScanDurationEstimator2.vi"("#points"=w959, "charge"=w951, "Time [s]"=w955) -> ("concatenated string"=w958:string)
                        n585 = Two Button Dialog(message=w958, 1:"No" ("F button name (\"Cancel\")"), 2:"Yes" ("T button name (\"OK\")")) -> (T button?=w953:bool)
                        n586 = case shown="True" w953 {
                          tunnel: w952 -> [_ w960]
                          frame False {
                          }
                          frame True {
                            n587 = local read "ScanQueue"() -> (w963:T11)
                            n588 = Array Size(array=w963) -> (size(s)=w961:i32)
                            n589 = Insert Into Array(array=w963, index=w961, new element=w960) -> (→"ScanQueue":T11)
                          }
                        }
                      }
                      frame False {
                        n590 = local read "total # of points"() -> (w974:i32)
                        n591 = call "ScanDurationEstimator2.vi"("#points"=w974, "charge"=w964, "Time [s]"=w967) -> ("concatenated string"=w973:string)
                        n592 = Two Button Dialog(message=w973, 1:"No" ("F button name (\"Cancel\")"), 2:"Yes" ("T button name (\"OK\")")) -> (T button?=w966:bool)
                        n593 = Select(t=AcquisitionModuleStates."PrepareMap" ("Enum"), s=w966, f=AcquisitionModuleStates."IDLE" ("Enum")) -> (s? t:f=w968:T2)
                        "ScanData" <- w965
                      }
                    }
                  }
                }
              }
            }
          }
          event "QUICKSCAN_Start 2", "Add To Queue 2": Value Change {
            n594 = event-data() -> ("CtlRef"=w979:refnum<vi>)  [unwired: 1 in, 5 out]
            n595 = local read "ScanReady?"() -> (w975:bool)
            n596 = property on="Add To Queue 2" class="Bool"() -> ("Label.Text"=w976:string)  [unwired: 2 in, 2 out]
            n597 = property class="Bool"(reference=w979) -> ("Label.Text"=w978:string)  [unwired: 1 in, 2 out]
            n598 = Equal?(x=w978, y=w976) -> (x = y?=w977:bool)
            n599 = stacked-sequence {
              seq-local: [w986 _] -> [_ w992]
              seq-local: [w983 _] -> [_ w991]
              seq-local: [w985 _] -> [_ w990]
              seq-local: [w984 _] -> [_ w989]
              tunnel: [_ w993] -> w980
              tunnel: w977 -> [_ w988]
              tunnel: w975 -> [_ w987]
              frame #0 {
                n600 = local read "ScanData"() -> (w983:T12)
                n601 = Unbundle By Name(w983) -> ("PresetVal"=w986:dbl, "CtPreset?"=w985:bool, "#points"=w984:i32)
                n602 = local write "ScanReady?"(FALSE ("ScanReady?")) -> ()
              }
              frame #1 {
                n603 = case shown="False" w988 {
                  tunnel: [AcquisitionModuleStates."IDLE" ("Enum") w1011] -> w993
                  tunnel: w992 -> [w999 w1010]
                  tunnel: w991 -> [w996 _]
                  tunnel: w990 -> [w995 w1009]
                  tunnel: w989 -> [w994 w1008]
                  tunnel: w987 -> [_ w1007]
                  frame True {
                    n604 = call "ScanDurationEstimator2.vi"("#points"=w994, "charge"=w995, "Time [s]"=w999) -> ("concatenated string"=w1002:string)
                    n605 = Two Button Dialog(message=w1002, 1:"No" ("F button name (\"Cancel\")"), 2:"Yes" ("T button name (\"OK\")")) -> (T button?=w997:bool)
                    n606 = case shown="True" w997 {
                      tunnel: w996 -> [_ w1004]
                      frame False {
                      }
                      frame True {
                        n607 = local read "ScanQueue"() -> (w1006:T11)
                        n608 = Array Size(array=w1006) -> (size(s)=w1005:i32)
                        n609 = Insert Into Array(array=w1006, index=w1005, new element=w1004) -> (w1003:T11)
                        n610 = local write "ScanQueue"(w1003) -> ()
                      }
                    }
                  }
                  frame False {
                    n611 = case shown="True" w1007 {
                      tunnel: [AcquisitionModuleStates."IDLE" ("Enum") w1017] -> w1011
                      tunnel: w1010 -> [_ w1016]
                      tunnel: w1009 -> [_ w1014]
                      tunnel: w1008 -> [_ w1013]
                      frame False {
                      }
                      frame True {
                        n612 = call "ScanDurationEstimator2.vi"("#points"=w1013, "charge"=w1014, "Time [s]"=w1016) -> ("concatenated string"=w1022:string)
                        n613 = Two Button Dialog(message=w1022, 1:"No" ("F button name (\"Cancel\")"), 2:"Yes" ("T button name (\"OK\")")) -> (T button?=w1015:bool)
                        n614 = Select(t=AcquisitionModuleStates."PrepareMap" ("Enum"), s=w1015, f=AcquisitionModuleStates."IDLE" ("Enum")) -> (s? t:f=w1017:T2)
                      }
                    }
                  }
                }
              }
            }
          }
          event "Up": Value Change {
            n615 = event-data() -> ("NewVal"=w1028:bool)  [unwired: 1 in, 5 out]
            n616 = local read "Assignment"() -> (w1023:cluster{"Microstep Size":dbl, "Device":string}[])
            n617 = Index Array(array=w1023, index=1) -> (element=w1024:cluster{"Microstep Size":dbl, "Device":string})
            n618 = case shown="True" w1028 {
              tunnel: w1024 -> [_ w1045]
              frame False {
                # "stop command"
                n619 = local read "Port"() -> (w1031:refnum<visa-resource-name>)
                n620 = local read "ZaberError"() -> (w1030:errorcluster)
                n621 = call "Stop.vi"("error in (no error)"=w1030, "VISA resource name"=w1031) -> ("error out"=w1029:errorcluster)  [unwired: 8 in, 1 out]
                n622 = local write "ZaberError"(w1029) -> ()
              }
              frame True {
                w1043 = u16 2 items=["device units", "microns/s^2", "mm/s^2", "inches/s^2", "degrees/s^2"] ("Units (0: data)")
                w1033 = u16 2 items=["device speed units", "microns per second", "millimeters per second", "inches per second", "degrees per second"] ("Units (0: device speed units)")
                # "move at specified velocity command"
                n623 = local read "ZaberError"() -> (w1041:errorcluster)
                n624 = local read "Acceleration [mm/s^2]"() -> (w1042:dbl)
                n625 = local read "Port"() -> (w1040:refnum<visa-resource-name>)
                n626 = local read "XY Speed\n[mm/s]"() -> (w1044:dbl)
                n627 = Negate(x=w1044) -> (-x=w1032:dbl)
                n628 = Unbundle(w1045) -> ("Microstep Size"=w1037:dbl, "Device"=w1036:string)
                n629 = call "Set Acceleration.vi"("Units (0: data)"=w1043, "New Acceleration"=w1042, "error in (no error)"=w1041, "Device and Axis"=w1036, "Microstep Size (0)"=w1037, "VISA resource name"=w1040) -> ("error out"=w1039:errorcluster, "VISA resource name out"=w1038:refnum<visa-resource-name>)  [unwired: 4 in]
                n630 = call "Move at Velocity.vi"("Units (0: device speed units)"=w1033, "Velocity"=w1032, "error in (no error)"=w1039, "Device and Axis"=w1036, "Microstep Size (0)"=w1037, "VISA resource name"=w1038) -> ("error out"=w1034:errorcluster, "VISA resource name out"=w1035:refnum<visa-resource-name>)  [unwired: 4 in]
                n631 = while {
                  shift-right: [w1050] -> _
                  shift-left: w1035 -> [w1053]
                  shift-right: [w1051] -> w1046
                  shift-left: w1034 -> [w1052]
                  tunnel: w1045 -> [w1049]
                  stop <- w1056 stop-if-true
                  w1055 = u16 2 items=["microsteps", "microns", "millimeters", "inches"] ("Units (0: microsteps)")
                  n632 = Unbundle(w1049) -> ("Microstep Size"=w1048:dbl, "Device"=w1047:string)
                  n633 = Wait (ms)(milliseconds to wait=u32 100) -> ()  [unwired: 1 out]
                  n634 = call "Read Current Position.vi"("Units (0: microsteps)"=w1055, "error in (no error)"=w1052, "Device and Axis"=w1047, "Microstep Size (0)"=w1048, "VISA resource name"=w1053) -> ("error out"=w1051:errorcluster, "Position"=w1054:dbl, "VISA resource name out"=w1050:refnum<visa-resource-name>)  [unwired: 4 in]
                  n635 = Not(x="Up") -> (.not. x?=w1056:bool)
                  n636 = local write "Y [mm]"(w1054) -> ()
                }
                n637 = local write "ZaberError"(w1046) -> ()
              }
            }
          }
          event "GoToY": Value Change {
            w1060 = u16 2 items=["device units", "microns/s^2", "mm/s^2", "inches/s^2", "degrees/s^2"] ("Units (0: data)")
            w1069 = u16 2 items=["device speed units", "microns per second", "millimeters per second", "inches per second", "degrees per second"] ("Units (0: device speed units)")
            w1075 = u16 2 items=["microsteps", "microns", "millimeters", "inches", "degrees"] ("Units (0: microsteps)")
            w1078 = u16 1 items=["relative", "absolute"] ("Movement Type (0: relative)")
            n638 = event-data() -> ()  [unwired: 1 in, 6 out]
            n639 = local read "Assignment"() -> (w1074:cluster{"Microstep Size":dbl, "Device":string}[])
            n640 = Index Array(array=w1074, index=1) -> (element=w1071:cluster{"Microstep Size":dbl, "Device":string})
            n641 = local read "Port"() -> (w1067:refnum<visa-resource-name>)
            n642 = local read "ZaberError"() -> (w1070:errorcluster)
            n643 = local read "XY Speed\n[mm/s]"() -> (w1068:dbl)
            n644 = Unbundle(w1071) -> ("Microstep Size"=w1066:dbl, "Device"=w1065:string)
            n645 = local read "Acceleration [mm/s^2]"() -> (w1059:dbl)
            n646 = call "Set Speed.vi"("Units (0: data)"=w1069, "New Speed"=w1068, "error in (no error)"=w1070, "Device and Axis"=w1065, "Microstep Size (0)"=w1066, "VISA resource name"=w1067) -> ("error out"=w1064:errorcluster, "VISA resource name out"=w1062:refnum<visa-resource-name>)  [unwired: 4 in]
            n647 = call "Set Acceleration.vi"("Units (0: data)"=w1060, "New Acceleration"=w1059, "error in (no error)"=w1064, "Device and Axis"=w1065, "Microstep Size (0)"=w1066, "VISA resource name"=w1062) -> ("error out"=w1063:errorcluster, "VISA resource name out"=w1061:refnum<visa-resource-name>)  [unwired: 4 in]
            n648 = Unbundle(w1071) -> ("Microstep Size"=w1073:dbl, "Device"=w1072:string)
            n649 = call "Move.vi"("Units (0: microsteps)"=w1075, "Movement Type (0: relative)"=w1078, "Move Distance (0)"="GoTo Y [mm]", "error in (no error)"=w1063, "Device and Axis"=w1072, "Microstep Size (0)"=w1073, "VISA resource name"=w1061) -> ("error out"=w1076:errorcluster)  [unwired: 3 in, 1 out]
            n650 = local write "ZaberError"(w1076) -> ()
          }
          event "GoToX": Value Change {
            w1083 = u16 2 items=["device units", "microns/s^2", "mm/s^2", "inches/s^2", "degrees/s^2"] ("Units (0: data)")
            w1094 = u16 2 items=["device speed units", "microns per second", "millimeters per second", "inches per second", "degrees per second"] ("Units (0: device speed units)")
            w1098 = u16 2 items=["microsteps", "microns", "millimeters", "inches", "degrees"] ("Units (0: microsteps)")
            w1100 = u16 1 items=["relative", "absolute"] ("Movement Type (0: relative)")
            # "move to point command"
            n651 = event-data() -> ()  [unwired: 1 in, 6 out]
            n652 = local read "Assignment"() -> (w1093:cluster{"Microstep Size":dbl, "Device":string}[])
            n653 = local read "XY Speed\n[mm/s]"() -> (w1096:dbl)
            n654 = local read "Port"() -> (w1095:refnum<visa-resource-name>)
            n655 = Index Array(array=w1093, index=0) -> (element=w1090:cluster{"Microstep Size":dbl, "Device":string})
            n656 = local read "ZaberError"() -> (w1097:errorcluster)
            n657 = Unbundle(w1090) -> ("Microstep Size"=w1085:dbl, "Device"=w1084:string)
            n658 = local read "Acceleration [mm/s^2]"() -> (w1082:dbl)
            n659 = call "Set Speed.vi"("Units (0: data)"=w1094, "New Speed"=w1096, "error in (no error)"=w1097, "Device and Axis"=w1084, "Microstep Size (0)"=w1085, "VISA resource name"=w1095) -> ("error out"=w1087:errorcluster, "VISA resource name out"=w1089:refnum<visa-resource-name>)  [unwired: 4 in]
            n660 = call "Set Acceleration.vi"("Units (0: data)"=w1083, "New Acceleration"=w1082, "error in (no error)"=w1087, "Device and Axis"=w1084, "Microstep Size (0)"=w1085, "VISA resource name"=w1089) -> ("error out"=w1086:errorcluster, "VISA resource name out"=w1088:refnum<visa-resource-name>)  [unwired: 4 in]
            n661 = Unbundle(w1090) -> ("Microstep Size"=w1092:dbl, "Device"=w1091:string)
            n662 = call "Move.vi"("Units (0: microsteps)"=w1098, "Movement Type (0: relative)"=w1100, "Move Distance (0)"="GoTo X [mm]", "error in (no error)"=w1086, "Device and Axis"=w1091, "Microstep Size (0)"=w1092, "VISA resource name"=w1088) -> ("error out"=w1099:errorcluster)  [unwired: 3 in, 1 out]
            n663 = local write "ZaberError"(w1099) -> ()
          }
          event "GoToZ": Value Change {
            w1112 = u16 2 items=["device units", "microns/s^2", "mm/s^2", "inches/s^2", "degrees/s^2"] ("Units (0: data)")
            w1114 = u16 2 items=["device speed units", "microns per second", "millimeters per second", "inches per second", "degrees per second"] ("Units (0: device speed units)")
            w1121 = u16 2 items=["microsteps", "microns", "millimeters", "inches", "degrees"] ("Units (0: microsteps)")
            w1124 = u16 1 items=["relative", "absolute"] ("Movement Type (0: relative)")
            # "move to point command"
            n664 = event-data() -> ()  [unwired: 1 in, 6 out]
            n665 = local read "Assignment"() -> (w1120:cluster{"Microstep Size":dbl, "Device":string}[])
            n666 = local read "ZaberError"() -> (w1113:errorcluster)
            n667 = Index Array(array=w1120, index=2) -> (element=w1119:cluster{"Microstep Size":dbl, "Device":string})
            n668 = local read "Speed Z [mm/s]"() -> (w1115:dbl)
            n669 = local read "Port"() -> (w1116:refnum<visa-resource-name>)
            n670 = Unbundle(w1119) -> ("Microstep Size"=w1106:dbl, "Device"=w1107:string)
            n671 = call "Set Speed.vi"("Units (0: data)"=w1114, "New Speed"=w1115, "error in (no error)"=w1113, "Device and Axis"=w1107, "Microstep Size (0)"=w1106, "VISA resource name"=w1116) -> ("error out"=w1109:errorcluster, "VISA resource name out"=w1111:refnum<visa-resource-name>)  [unwired: 4 in]
            n672 = local read "Acceleration [mm/s^2]"() -> (w1105:dbl)
            n673 = call "Set Acceleration.vi"("Units (0: data)"=w1112, "New Acceleration"=w1105, "error in (no error)"=w1109, "Device and Axis"=w1107, "Microstep Size (0)"=w1106, "VISA resource name"=w1111) -> ("error out"=w1108:errorcluster, "VISA resource name out"=w1110:refnum<visa-resource-name>)  [unwired: 4 in]
            n674 = Unbundle(w1119) -> ("Microstep Size"=w1118:dbl, "Device"=w1117:string)
            n675 = call "Move.vi"("Units (0: microsteps)"=w1121, "Movement Type (0: relative)"=w1124, "Move Distance (0)"="GoTo Z [mm]", "error in (no error)"=w1108, "Device and Axis"=w1117, "Microstep Size (0)"=w1118, "VISA resource name"=w1110) -> ("error out"=w1123:errorcluster)  [unwired: 3 in, 1 out]
            n676 = local write "ZaberError"(w1123) -> ()
          }
          event "StopMotion": Value Change {
            # "stop command"
            n677 = event-data() -> ()  [unwired: 1 in, 6 out]
            n678 = local read "Assignment"() -> (w1131:cluster{"Microstep Size":dbl, "Device":string}[])
            n679 = local read "ZaberError"() -> (w1129:errorcluster)
            n680 = local read "Port"() -> (w1130:refnum<visa-resource-name>)
            n681 = for {
              tunnel: w1131 -> [w1135] mode=indexing
              shift-right: [w1136] -> _
              shift-left: w1130 -> [w1139]
              shift-right: [w1137] -> w1128
              shift-left: w1129 -> [w1138]
              n682 = Unbundle(w1135) -> ("Device"=w1134:string)  [unwired: 1 out]
              n683 = call "Stop.vi"("error in (no error)"=w1138, "Device and Axis"=w1134, "VISA resource name"=w1139) -> ("error out"=w1137:errorcluster, "VISA resource name out"=w1136:refnum<visa-resource-name>)  [unwired: 7 in]
            }
            n684 = local write "ZaberError"(w1128) -> ()
          }
          event "Down": Value Change {
            n685 = event-data() -> ("NewVal"=w1143:bool)  [unwired: 1 in, 5 out]
            n686 = local read "Assignment"() -> (w1140:cluster{"Microstep Size":dbl, "Device":string}[])
            n687 = Index Array(array=w1140, index=1) -> (element=w1141:cluster{"Microstep Size":dbl, "Device":string})
            n688 = case shown="True" w1143 {
              tunnel: w1141 -> [_ w1161]
              frame False {
                # "stop command"
                n689 = local read "Port"() -> (w1148:refnum<visa-resource-name>)
                n690 = local read "ZaberError"() -> (w1147:errorcluster)
                n691 = call "Stop.vi"("error in (no error)"=w1147, "VISA resource name"=w1148) -> ("error out"=w1146:errorcluster)  [unwired: 8 in, 1 out]
                n692 = local write "ZaberError"(w1146) -> ()
              }
              frame True {
                w1160 = u16 2 items=["device units", "microns/s^2", "mm/s^2", "inches/s^2", "degrees/s^2"] ("Units (0: data)")
                w1151 = u16 2 items=["device speed units", "microns per second", "millimeters per second", "inches per second", "degrees per second"] ("Units (0: device speed units)")
                # "move at specified velocity command"
                n693 = local read "Acceleration [mm/s^2]"() -> (w1159:dbl)
                n694 = local read "ZaberError"() -> (w1157:errorcluster)
                n695 = local read "Port"() -> (w1158:refnum<visa-resource-name>)
                n696 = local read "XY Speed\n[mm/s]"() -> (w1152:dbl)
                n697 = Unbundle(w1161) -> ("Microstep Size"=w1149:dbl, "Device"=w1150:string)
                n698 = call "Set Acceleration.vi"("Units (0: data)"=w1160, "New Acceleration"=w1159, "error in (no error)"=w1157, "Device and Axis"=w1150, "Microstep Size (0)"=w1149, "VISA resource name"=w1158) -> ("error out"=w1155:errorcluster, "VISA resource name out"=w1156:refnum<visa-resource-name>)  [unwired: 4 in]
                n699 = call "Move at Velocity.vi"("Units (0: device speed units)"=w1151, "Velocity"=w1152, "error in (no error)"=w1155, "Device and Axis"=w1150, "Microstep Size (0)"=w1149, "VISA resource name"=w1156) -> ("error out"=w1153:errorcluster, "VISA resource name out"=w1154:refnum<visa-resource-name>)  [unwired: 4 in]
                n700 = while {
                  shift-right: [w1167] -> _
                  shift-left: w1154 -> [w1170]
                  shift-right: [w1168] -> w1162
                  shift-left: w1153 -> [w1169]
                  tunnel: w1161 -> [w1163]
                  stop <- w1173 stop-if-true
                  w1172 = u16 2 items=["microsteps", "microns", "millimeters", "inches"] ("Units (0: microsteps)")
                  n701 = Wait (ms)(milliseconds to wait=u32 100) -> ()  [unwired: 1 out]
                  n702 = Unbundle(w1163) -> ("Microstep Size"=w1165:dbl, "Device"=w1164:string)
                  n703 = call "Read Current Position.vi"("Units (0: microsteps)"=w1172, "error in (no error)"=w1169, "Device and Axis"=w1164, "Microstep Size (0)"=w1165, "VISA resource name"=w1170) -> ("error out"=w1168:errorcluster, "Position"=w1171:dbl, "VISA resource name out"=w1167:refnum<visa-resource-name>)  [unwired: 4 in]
                  n704 = Not(x="Down") -> (.not. x?=w1173:bool)
                  n705 = local write "Y [mm]"(w1171) -> ()
                }
                n706 = local write "ZaberError"(w1162) -> ()
              }
            }
          }
          event "Closer": Value Change {
            n707 = event-data() -> ("NewVal"=w1176:bool)  [unwired: 1 in, 5 out]
            n708 = local read "Assignment"() -> (w1175:cluster{"Microstep Size":dbl, "Device":string}[])
            n709 = Index Array(array=w1175, index=2) -> (element=w1177:cluster{"Microstep Size":dbl, "Device":string})
            n710 = case shown="True" w1176 {
              tunnel: w1177 -> [_ w1196]
              frame False {
                # "stop command"
                n711 = local read "Port"() -> (w1183:refnum<visa-resource-name>)
                n712 = local read "ZaberError"() -> (w1182:errorcluster)
                n713 = call "Stop.vi"("error in (no error)"=w1182, "VISA resource name"=w1183) -> ("error out"=w1181:errorcluster)  [unwired: 8 in, 1 out]
                n714 = local write "ZaberError"(w1181) -> ()
              }
              frame True {
                w1184 = u16 2 items=["device units", "microns/s^2", "mm/s^2", "inches/s^2", "degrees/s^2"] ("Units (0: data)")
                w1195 = u16 2 items=["device speed units", "microns per second", "millimeters per second", "inches per second", "degrees per second"] ("Units (0: device speed units)")
                # "move at specified velocity command"
                n715 = local read "Speed Z [mm/s]"() -> (w1192:dbl)
                n716 = local read "ZaberError"() -> (w1194:errorcluster)
                n717 = local read "Port"() -> (w1193:refnum<visa-resource-name>)
                n718 = local read "Acceleration [mm/s^2]"() -> (w1187:dbl)
                n719 = Unbundle(w1196) -> ("Microstep Size"=w1189:dbl, "Device"=w1188:string)
                n720 = call "Set Speed.vi"("Units (0: data)"=w1195, "New Speed"=w1192, "error in (no error)"=w1194, "Device and Axis"=w1188, "Microstep Size (0)"=w1189, "VISA resource name"=w1193) -> ("error out"=w1190:errorcluster, "VISA resource name out"=w1191:refnum<visa-resource-name>)  [unwired: 4 in]
                n721 = call "Set Acceleration.vi"("Units (0: data)"=w1184, "New Acceleration"=w1187, "error in (no error)"=w1190, "Device and Axis"=w1188, "Microstep Size (0)"=w1189, "VISA resource name"=w1191) -> ("error out"=w1186:errorcluster, "VISA resource name out"=w1185:refnum<visa-resource-name>)  [unwired: 4 in]
                n722 = while {
                  shift-right: [w1203] -> _
                  shift-left: w1185 -> [w1206]
                  shift-right: [w1204] -> w1197
                  shift-left: w1186 -> [w1205]
                  tunnel: w1196 -> [w1198]
                  stop <- w1208 stop-if-true
                  w1207 = u16 2 items=["microsteps", "microns", "millimeters", "inches"] ("Units (0: microsteps)")
                  n723 = Wait (ms)(milliseconds to wait=u32 100) -> ()  [unwired: 1 out]
                  n724 = Unbundle(w1198) -> ("Microstep Size"=w1200:dbl, "Device"=w1199:string)
                  n725 = call "Read Current Position.vi"("Units (0: microsteps)"=w1207, "error in (no error)"=w1205, "Device and Axis"=w1199, "Microstep Size (0)"=w1200, "VISA resource name"=w1206) -> ("error out"=w1204:errorcluster, "Position"=w1202:dbl, "VISA resource name out"=w1203:refnum<visa-resource-name>)  [unwired: 4 in]
                  n726 = Not(x="Closer") -> (.not. x?=w1208:bool)
                  n727 = local write "Z [mm]"(w1202) -> ()
                }
                n728 = local write "ZaberError"(w1197) -> ()
              }
            }
          }
          event "OpenScanBuilder": Value Change {
            n729 = event-data() -> ()  [unwired: 1 in, 6 out]
            n730 = local read "Scan\nCorners"() -> (w1215:dbl[][])
            n731 = local read "ROI_Array"() -> (w1210:T7)
            n732 = call "ScanBuilder.vi"("Selected\nScan\nCorners"=w1215, "ROI_Array 2"=w1210) -> ("Do?"=w1213:bool, "ScanData"=w1214:T23)
            "ScanReady?" <- w1213
            n733 = case shown="True" w1213 {
              tunnel: w1214 -> [_ w1220]
              tunnel: [w1218 w1219] -> w1212
              tunnel: [w1218 w1219] -> w1211
              frame False {
                w1218 = T15."Disabled and Grayed Out" ("Disabled")
              }
              frame True {
                w1219 = T15."Enabled" ("Disabled")
                n734 = local write "ScanData"(w1220) -> ()
              }
            }
            n735 = property on="QUICKSCAN_Start 2" class="Bool"("DisabledEnum"=w1211) -> ()  [unwired: 2 in, 2 out]
            n736 = property on="Add To Queue 2" class="Bool"("DisabledEnum"=w1212) -> ()  [unwired: 2 in, 2 out]
          }
          event "UpperLeft", "Clear", "LowerRight", "LowerLeft", "UpperRight": Value Change {
            n737 = event-data() -> ("CtlRef"=w1221:refnum<vi>)  [unwired: 1 in, 5 out]
            n738 = stacked-sequence {
              seq-local: [w1228 _ _] -> [_ w1242 w1263]
              tunnel: w1221 -> [w1227 w1250 _]
              frame #0 {
                n739 = property class="Bool"(reference=w1227) -> ("Label.Text"=w1226:string)  [unwired: 1 in, 2 out]
                n740 = Equal?(x=w1226, y="Clear") -> (x = y?=w1224:bool)
                n741 = case shown="False" w1224 {
                  tunnel: [w1229 FALSE] -> w1228
                  frame False {
                    n742 = local read "Scan\nCorners"() -> (w1234:dbl[][])
                    n743 = local read "X [mm]"() -> (w1239:dbl)
                    n744 = local read "Y [mm]"() -> (w1238:dbl)
                    n745 = local read "Z [mm]"() -> (w1237:dbl)
                    n746 = Array Size(array=w1234) -> (size(s)=w1235:i32[])
                    n747 = Build Array(w1239, w1238, w1237) -> (w1233:dbl[])
                    n748 = Index Array(array=w1235, index=0) -> (element=w1231:i32)
                    n749 = Insert Into Array(array=w1234, index (row)=w1231, new element=w1233) -> (w1232:dbl[][])  [unwired: 1 in]
                    n750 = Equal?(x=w1231, y=1) -> (x = y?=w1229:bool)
                    n751 = local write "Scan\nCorners"(w1232) -> ()
                  }
                  frame True {
                  }
                }
              }
              frame #1 {
                w1244 = T15."Disabled and Grayed Out" ("Disabled")
                n752 = property class="Bool"(reference=w1250) -> ("Label.Text"=w1249:string)  [unwired: 1 in, 2 out]
                n753 = Select(t=w1244, s=w1242, f=T15."Enabled" ("Disabled")) -> (s? t:f=w1241:T15)
                n754 = case shown="\"Clear\", Default" w1249 {
                  tunnel: [w1252 w1254 w1255 w1260 w1262] -> w1248
                  tunnel: [w1252 w1253 w1256 w1260 w1262] -> w1247
                  tunnel: [w1251 w1254 w1256 w1260 w1262] -> w1246
                  tunnel: [w1252 w1254 w1256 w1260 w1261] -> w1245
                  tunnel: w1244 -> [w1252 w1254 w1256 _ w1262]
                  tunnel: w1241 -> [w1251 w1253 w1255 _ w1261]
                  frame "UpperRight" {
                  }
                  frame "LowerLeft" {
                  }
                  frame "LowerRight" {
                  }
                  frame "Clear", Default {
                    w1260 = T15."Enabled" ("Disabled")
                    n755 = local write "ZnotEqual"(FALSE ("ZnotEqual")) -> ()
                    n756 = property on="OpenScanBuilder" class="Bool"("DisabledEnum"=T15."Disabled and Grayed Out" ("Disabled")) -> ()  [unwired: 2 in, 2 out]
                    "Scan\nCorners" <- dbl[][] []
                  }
                  frame "UpperLeft" {
                  }
                }
                n757 = property on="UpperLeft" class="Bool"("DisabledEnum"=w1248) -> ()  [unwired: 2 in, 2 out]
                n758 = property on="UpperRight" class="Bool"("DisabledEnum"=w1247) -> ()  [unwired: 2 in, 2 out]
                n759 = property on="LowerLeft" class="Bool"("DisabledEnum"=w1246) -> ()  [unwired: 2 in, 2 out]
                n760 = property on="LowerRight" class="Bool"("DisabledEnum"=w1245) -> ()  [unwired: 2 in, 2 out]
              }
              frame #2 {
                n761 = case shown="True" w1263 {
                  frame False {
                  }
                  frame True {
                    w1273 = 2 ("disabled index (col)")
                    n762 = local read "Scan\nCorners"() -> (w1274:dbl[][])
                    n763 = property on="OpenScanBuilder" class="Bool"("DisabledEnum"=T15."Enabled" ("Disabled")) -> ()  [unwired: 2 in, 2 out]
                    n764 = Delete From Array(array=w1274, length=w1273, index (col)=w1273) -> (deleted portion=w1272:dbl[][])  [unwired: 1 in, 1 out]
                    n765 = Reshape Array(w1272, 2 ("dimension size")) -> (w1270:dbl[])
                    n766 = Index Array(array=w1270, index=0) -> (element=w1267:dbl)
                    n767 = Index Array(array=w1270, index=1) -> (element=w1266:dbl)
                    n768 = Not Equal?(x=w1267, y=w1266) -> (x != y?=→"ZnotEqual":bool)
                  }
                }
              }
            }
          }
          event "Left": Value Change {
            n769 = event-data() -> ("NewVal"=w1276:bool)  [unwired: 1 in, 5 out]
            n770 = local read "Assignment"() -> (w1275:cluster{"Microstep Size":dbl, "Device":string}[])
            n771 = Index Array(array=w1275, index=0) -> (element=w1277:cluster{"Microstep Size":dbl, "Device":string})
            n772 = case shown="True" w1276 {
              tunnel: w1277 -> [_ w1296]
              frame False {
                # "stop command"
                n773 = local read "Port"() -> (w1283:refnum<visa-resource-name>)
                n774 = local read "ZaberError"() -> (w1282:errorcluster)
                n775 = call "Stop.vi"("error in (no error)"=w1282, "VISA resource name"=w1283) -> ("error out"=w1281:errorcluster)  [unwired: 8 in, 1 out]
                n776 = local write "ZaberError"(w1281) -> ()
              }
              frame True {
                w1295 = u16 2 items=["device units", "microns/s^2", "mm/s^2", "inches/s^2", "degrees/s^2"] ("Units (0: data)")
                w1285 = u16 2 items=["device speed units", "microns per second", "millimeters per second", "inches per second", "degrees per second"] ("Units (0: device speed units)")
                # "move at specified velocity command"
                n777 = local read "ZaberError"() -> (w1292:errorcluster)
                n778 = local read "XY Speed\n[mm/s]"() -> (w1297:dbl)
                n779 = local read "Port"() -> (w1293:refnum<visa-resource-name>)
                n780 = Negate(x=w1297) -> (-x=w1284:dbl)
                n781 = local read "Acceleration [mm/s^2]"() -> (w1294:dbl)
                n782 = Unbundle(w1296) -> ("Microstep Size"=w1287:dbl, "Device"=w1286:string)
                n783 = call "Set Acceleration.vi"("Units (0: data)"=w1295, "New Acceleration"=w1294, "error in (no error)"=w1292, "Device and Axis"=w1286, "Microstep Size (0)"=w1287, "VISA resource name"=w1293) -> ("error out"=w1290:errorcluster, "VISA resource name out"=w1291:refnum<visa-resource-name>)  [unwired: 4 in]
                n784 = call "Move at Velocity.vi"("Units (0: device speed units)"=w1285, "Velocity"=w1284, "error in (no error)"=w1290, "Device and Axis"=w1286, "Microstep Size (0)"=w1287, "VISA resource name"=w1291) -> ("error out"=w1288:errorcluster, "VISA resource name out"=w1289:refnum<visa-resource-name>)  [unwired: 4 in]
                n785 = while {
                  shift-right: [w1304] -> _
                  shift-left: w1289 -> [w1307]
                  shift-right: [w1305] -> w1298
                  shift-left: w1288 -> [w1306]
                  tunnel: w1296 -> [w1301]
                  stop <- w1309 stop-if-true
                  w1308 = u16 2 items=["microsteps", "microns", "millimeters", "inches"] ("Units (0: microsteps)")
                  n786 = Unbundle(w1301) -> ("Microstep Size"=w1300:dbl, "Device"=w1299:string)
                  n787 = Wait (ms)(milliseconds to wait=u32 100) -> ()  [unwired: 1 out]
                  n788 = call "Read Current Position.vi"("Units (0: microsteps)"=w1308, "error in (no error)"=w1306, "Device and Axis"=w1299, "Microstep Size (0)"=w1300, "VISA resource name"=w1307) -> ("error out"=w1305:errorcluster, "Position"=w1303:dbl, "VISA resource name out"=w1304:refnum<visa-resource-name>)  [unwired: 4 in]
                  n789 = Not(x="Left") -> (.not. x?=w1309:bool)
                  n790 = local write "X [mm]"(w1303) -> ()
                }
                n791 = local write "ZaberError"(w1298) -> ()
              }
            }
          }
          event "Right": Value Change {
            n792 = event-data() -> ("NewVal"=w1312:bool)  [unwired: 1 in, 5 out]
            n793 = local read "Assignment"() -> (w1311:cluster{"Microstep Size":dbl, "Device":string}[])
            n794 = Index Array(array=w1311, index=0) -> (element=w1313:cluster{"Microstep Size":dbl, "Device":string})
            n795 = case shown="True" w1312 {
              tunnel: w1313 -> [_ w1332]
              frame False {
                # "stop command"
                n796 = local read "Port"() -> (w1319:refnum<visa-resource-name>)
                n797 = local read "ZaberError"() -> (w1318:errorcluster)
                n798 = call "Stop.vi"("error in (no error)"=w1318, "VISA resource name"=w1319) -> ("error out"=w1317:errorcluster)  [unwired: 8 in, 1 out]
                n799 = local write "ZaberError"(w1317) -> ()
              }
              frame True {
                w1331 = u16 2 items=["device units", "microns/s^2", "mm/s^2", "inches/s^2", "degrees/s^2"] ("Units (0: data)")
                w1321 = u16 2 items=["device speed units", "microns per second", "millimeters per second", "inches per second", "degrees per second"] ("Units (0: device speed units)")
                # "move at specified velocity command"
                n800 = local read "Acceleration [mm/s^2]"() -> (w1330:dbl)
                n801 = local read "ZaberError"() -> (w1329:errorcluster)
                n802 = local read "XY Speed\n[mm/s]"() -> (w1320:dbl)
                n803 = local read "Port"() -> (w1328:refnum<visa-resource-name>)
                n804 = Unbundle(w1332) -> ("Microstep Size"=w1323:dbl, "Device"=w1322:string)
                n805 = call "Set Acceleration.vi"("Units (0: data)"=w1331, "New Acceleration"=w1330, "error in (no error)"=w1329, "Device and Axis"=w1322, "Microstep Size (0)"=w1323, "VISA resource name"=w1328) -> ("error out"=w1327:errorcluster, "VISA resource name out"=w1326:refnum<visa-resource-name>)  [unwired: 4 in]
                n806 = call "Move at Velocity.vi"("Units (0: device speed units)"=w1321, "Velocity"=w1320, "error in (no error)"=w1327, "Device and Axis"=w1322, "Microstep Size (0)"=w1323, "VISA resource name"=w1326) -> ("error out"=w1324:errorcluster, "VISA resource name out"=w1325:refnum<visa-resource-name>)  [unwired: 4 in]
                n807 = while {
                  shift-right: [w1339] -> _
                  shift-left: w1325 -> [w1342]
                  shift-right: [w1340] -> w1333
                  shift-left: w1324 -> [w1341]
                  tunnel: w1332 -> [w1334]
                  stop <- w1344 stop-if-true
                  w1343 = u16 2 items=["microsteps", "microns", "millimeters", "inches"] ("Units (0: microsteps)")
                  n808 = Wait (ms)(milliseconds to wait=u32 100) -> ()  [unwired: 1 out]
                  n809 = Unbundle(w1334) -> ("Microstep Size"=w1336:dbl, "Device"=w1335:string)
                  n810 = call "Read Current Position.vi"("Units (0: microsteps)"=w1343, "error in (no error)"=w1341, "Device and Axis"=w1335, "Microstep Size (0)"=w1336, "VISA resource name"=w1342) -> ("error out"=w1340:errorcluster, "Position"=w1338:dbl, "VISA resource name out"=w1339:refnum<visa-resource-name>)  [unwired: 4 in]
                  n811 = Not(x="Right") -> (.not. x?=w1344:bool)
                  n812 = local write "X [mm]"(w1338) -> ()
                }
                n813 = local write "ZaberError"(w1333) -> ()
              }
            }
          }
          event "Away": Value Change {
            n814 = event-data() -> ("NewVal"=w1347:bool)  [unwired: 1 in, 5 out]
            n815 = local read "Assignment"() -> (w1346:cluster{"Microstep Size":dbl, "Device":string}[])
            n816 = Index Array(array=w1346, index=2) -> (element=w1348:cluster{"Microstep Size":dbl, "Device":string})
            n817 = case shown="True" w1347 {
              tunnel: w1348 -> [_ w1367]
              frame False {
                # "stop command"
                n818 = local read "Port"() -> (w1354:refnum<visa-resource-name>)
                n819 = local read "ZaberError"() -> (w1353:errorcluster)
                n820 = call "Stop.vi"("error in (no error)"=w1353, "VISA resource name"=w1354) -> ("error out"=w1352:errorcluster)  [unwired: 8 in, 1 out]
                n821 = local write "ZaberError"(w1352) -> ()
              }
              frame True {
                w1356 = u16 2 items=["device units", "microns/s^2", "mm/s^2", "inches/s^2", "degrees/s^2"] ("Units (0: data)")
                w1365 = u16 2 items=["device speed units", "microns per second", "millimeters per second", "inches per second", "degrees per second"] ("Units (0: device speed units)")
                # "move at specified velocity command"
                n822 = local read "Speed Z [mm/s]"() -> (w1368:dbl)
                n823 = local read "ZaberError"() -> (w1364:errorcluster)
                n824 = local read "Port"() -> (w1363:refnum<visa-resource-name>)
                n825 = Negate(x=w1368) -> (-x=w1366:dbl)
                n826 = local read "Acceleration [mm/s^2]"() -> (w1355:dbl)
                n827 = Unbundle(w1367) -> ("Microstep Size"=w1358:dbl, "Device"=w1357:string)
                n828 = call "Set Speed.vi"("Units (0: data)"=w1365, "New Speed"=w1366, "error in (no error)"=w1364, "Device and Axis"=w1357, "Microstep Size (0)"=w1358, "VISA resource name"=w1363) -> ("error out"=w1360:errorcluster, "VISA resource name out"=w1362:refnum<visa-resource-name>)  [unwired: 4 in]
                n829 = call "Set Acceleration.vi"("Units (0: data)"=w1356, "New Acceleration"=w1355, "error in (no error)"=w1360, "Device and Axis"=w1357, "Microstep Size (0)"=w1358, "VISA resource name"=w1362) -> ("error out"=w1359:errorcluster, "VISA resource name out"=w1361:refnum<visa-resource-name>)  [unwired: 4 in]
                n830 = while {
                  shift-right: [w1375] -> _
                  shift-left: w1361 -> [w1378]
                  shift-right: [w1376] -> w1369
                  shift-left: w1359 -> [w1377]
                  tunnel: w1367 -> [w1372]
                  stop <- w1380 stop-if-true
                  w1379 = u16 2 items=["microsteps", "microns", "millimeters", "inches"] ("Units (0: microsteps)")
                  n831 = Unbundle(w1372) -> ("Microstep Size"=w1371:dbl, "Device"=w1370:string)
                  n832 = Wait (ms)(milliseconds to wait=u32 100) -> ()  [unwired: 1 out]
                  n833 = call "Read Current Position.vi"("Units (0: microsteps)"=w1379, "error in (no error)"=w1377, "Device and Axis"=w1370, "Microstep Size (0)"=w1371, "VISA resource name"=w1378) -> ("error out"=w1376:errorcluster, "Position"=w1374:dbl, "VISA resource name out"=w1375:refnum<visa-resource-name>)  [unwired: 4 in]
                  n834 = Not(x="Away") -> (.not. x?=w1380:bool)
                  n835 = local write "Z [mm]"(w1374) -> ()
                }
                n836 = local write "ZaberError"(w1369) -> ()
              }
            }
          }
          event "Reduced Speed": Value Change {
            n837 = event-data() -> ("NewVal"=w1396:bool)  [unwired: 1 in, 5 out]
            n838 = case shown="False" w1396 {
              tunnel: [1.0 ("Minimum") 0.1 ("Minimum")] -> w1393
              tunnel: [75.0 ("Minimum") 7.5 ("Minimum")] -> w1392
              tunnel: [1.0 ("Minimum") 0.1 ("Minimum")] -> w1391
              tunnel: [0.5 ("Minimum") 0.05 ("Minimum")] -> w1384
              tunnel: [10.0 ("Minimum") 1.0 ("Minimum")] -> w1383
              tunnel: [0.5 ("Minimum") 0.05 ("Minimum")] -> w1382
              frame False {
                # "full speed"
              }
              frame True {
                # "reduced speed"
              }
            }
            n839 = property on="Speed Z [mm/s]" class="Slide (strict)"() -> ("Data Range"=w1386:T24, "Scale.Range"=w1385:T25)  [unwired: 2 in, 2 out]
            n840 = property on="XY Speed\n[mm/s]" class="Slide (strict)"() -> ("Data Range"=w1398:T24, "Scale.Range"=w1390:T25)  [unwired: 2 in, 2 out]
            n841 = Bundle By Name(cluster=w1398, "Minimum"=w1393, "Maximum"=w1392, "Increment"=w1391) -> (w1397:T24)
            n842 = Bundle By Name(cluster=w1390, "Minimum"=w1393, "Maximum"=w1392, "Increment"=w1391) -> (w1389:T25)
            n843 = Bundle By Name(cluster=w1386, "Minimum"=w1384, "Maximum"=w1383, "Increment"=w1382) -> (w1388:T24)
            n844 = Bundle By Name(cluster=w1385, "Minimum"=w1384, "Maximum"=w1383, "Increment"=w1382) -> (w1387:T25)
            n845 = property on="XY Speed\n[mm/s]" class="Slide (strict)"("Data Range"=w1397, "Scale.Range"=w1389) -> ()  [unwired: 2 in, 2 out]
            n846 = property on="Speed Z [mm/s]" class="Slide (strict)"("Data Range"=w1388, "Scale.Range"=w1387) -> ()  [unwired: 2 in, 2 out]
          }
          event "QUEUE_Run": Value Change {
            w1413 = TRUE ("QUEUE_Run")
            n847 = event-data() -> ()  [unwired: 1 in, 6 out]
            n848 = local write "QUEUE_Run"(w1413) -> ()
            "queue mode" <- w1413
          }
          event "SpectrumType": Value Change {
            n849 = event-data() -> ()  [unwired: 1 in, 6 out]
            n850 = case shown="0, Default" "SpectrumType" {
              tunnel: [w1418 w1419 w1420] -> w1414
              frame 0, Default {
                n851 = local read "SumSpectra"() -> (w1418:u64[])
              }
              frame 1 {
                n852 = local read "MaxSpectra"() -> (w1419:u64[])
              }
              frame 2 {
                n853 = local read "LastSpectra"() -> (w1420:u32[])
              }
            }
            "SpectraPlot" <- w1414
          }
          event Value Change {
            n854 = event-data() -> ()  [unwired: 1 in, 6 out]
          }
          event Panel Close? {
            n855 = event-data() -> ()  [unwired: 1 in, 4 out]
            n856 = local read "Library state"() -> (w1425:bool)
            n857 = case shown="True" w1425 {
              selector: w1425 -> [w1429 _]
              tunnel: w1424 -> [w1430 w1435]
              tunnel: [w1430 w1434] -> w1423
              tunnel: [w1429 w1431] -> w1422
              frame False {
              }
              frame True {
                n858 = call "Close Library.vi"("error in (no error)"=w1435) -> ("error out"=w1438:errorcluster, "function return"=w1432:bool)  [unwired: 9 in]
                n859 = Not(x=w1432) -> (.not. x?=w1431:bool)
                n860 = local write "identifier out"("" ("identifier out")) -> ()
                n861 = call "CheckError.vi"("error in (no error)"=w1438, "ret_val"=w1432) -> ("error out"=w1437:errorcluster)
                n862 = call "reset Last Error.vi"("error in (no error)"=w1437) -> ("error out"=w1434:errorcluster)  [unwired: 9 in, 1 out]
                n863 = Unbundle By Name(w1434) -> ("code"=→"Error code":i32)
              }
            }
            n864 = local write "Library state"(w1422) -> ()
            n865 = event-data("Discard?"=TRUE) -> ()  [unwired: 1 in, 1 out]
          }
          event "Configure": Value Change {
            n866 = event-data() -> ()  [unwired: 1 in, 6 out]
            n867 = call "Load_XML2.vi"("XML File Path 2"="Config. file path") -> ("DPP Configuration"=→"DPP Configuration":T26)  [unwired: 10 in]
            n868 = local read "DPP Configuration"() -> (w1448:T1)
            n869 = local read "identifier out"() -> (w1445:string)
            n870 = call "configure.vi"("DPP Configuration"=w1448, "Board"=u16 0, "identifier"=w1445) -> ("function return"=w1443:u32, "error out"=w1444:errorcluster)  [unwired: 3 in]
            n871 = Not Equal To 0?(x=w1443) -> (x != 0?=w1442:bool)
            n872 = Unbundle By Name(w1444) -> ("code"=w1447:i32)
            n873 = Unbundle By Name(w1444) -> ()  [unwired: 1 out]
            n874 = call "CheckError.vi"("error in (no error)"=w1444, "ret_val"=w1442) -> ()  [unwired: 1 out]
            n875 = local write "Error code 2"(w1447) -> ()
          }
          event "ROI_Add": Value Change {
            n876 = event-data() -> ()  [unwired: 1 in, 5 out]
            n877 = stacked-sequence {
              seq-local: [_ w1459 _ _ _] -> [_ _ w1510 _ _]
              seq-local: [_ w1458 _ _ _] -> [_ _ w1509 _ _]
              frame #0 {
                w1454 = TRUE ("Cursor.Visible")
                w1456 = T15."Enabled" ("Disabled")
                n878 = control-ref of="SpectraPlot"() -> (w1451:refnum<vi>)
                n879 = property class="WFGraph (strict)"(reference=w1451, "Active Cursor"=u32 0, "Cursor.Visible"=w1454, "Active Cursor"=u32 1, "Cursor.Visible"=w1454) -> ()  [unwired: 1 in, 2 out]
                n880 = property on="ROI_Add" class="Bool"("DisabledEnum"=T15."Disabled and Grayed Out" ("Disabled")) -> ()  [unwired: 2 in, 2 out]
                n881 = property on="ROI_Set" class="Bool (strict)"("DisabledEnum"=w1456) -> ()  [unwired: 2 in, 2 out]
                n882 = property on="ROI_Cancel" class="Bool (strict)"("DisabledEnum"=w1456) -> ()  [unwired: 2 in, 2 out]
                n883 = property on="SpectraPlot" class="WFGraph (strict)"() -> ("Value"=w1455:u64[])  [unwired: 2 in, 2 out]
                n884 = property on="SpectraPlot" class="WFGraph (strict)"("Val(Sgnl)"=w1455) -> ()  [unwired: 2 in, 2 out]
              }
              frame #1 {
                n885 = while {
                  tunnel: [w1462] -> w1459
                  tunnel: [w1460] -> w1458
                  stop <- w1461 stop-if-true
                  n886 = event shown="[1] \"SpectraPlot\": Mouse Up" {
                    selector: _ -> [_ _ _ _ _]
                    dyn-events: _ -> [_ _ _ _ _]
                    timeout: 10 -> [_ _ _ _ _]
                    tunnel: [TRUE TRUE TRUE FALSE TRUE] -> w1462
                    tunnel: [FALSE FALSE FALSE TRUE TRUE] -> w1461
                    tunnel: [_ _ _ _ w1506] -> w1460
                    event Timeout {
                      n887 = event-data() -> ()  [unwired: 1 in, 2 out]
                    }
                    event "SpectraPlot": Mouse Up {
                      n888 = event-data() -> ()  [unwired: 1 in, 1 out]
                      n889 = local read "Intercept"() -> (w1468:dbl)
                      n890 = control-ref of="SpectraPlot"() -> (w1470:refnum<vi>)
                      n891 = property class="WFGraph (strict)"(reference=w1470, "Active Cursor"=u32 1, "Active Cursor"=u32 0) -> ("Cursor.Cursor X"=w1476:dbl, "Cursor.Cursor X"=w1475:dbl)  [unwired: 1 in, 2 out]
                      n892 = local read "Slope"() -> (w1469:dbl)
                      n893 = local read "APPEARANCE_E/CH"() -> (w1474:bool)
                      n894 = case shown="False" w1474 {
                        tunnel: [w1486 w1492] -> w1472
                        tunnel: [w1485 w1491] -> w1471
                        tunnel: w1469 -> [_ w1488]
                        tunnel: w1468 -> [_ w1487]
                        tunnel: w1476 -> [w1486 w1490]
                        tunnel: w1475 -> [w1485 w1489]
                        frame False {
                        }
                        frame True {
                          n895 = call "SUB_EnergyToChannel.vi"("Intercept"=w1487, "Slope"=w1488, "Energy"=w1490) -> ("Channel"=w1492:u32)
                          n896 = call "SUB_EnergyToChannel.vi"("Intercept"=w1487, "Slope"=w1488, "Energy"=w1489) -> ("Channel"=w1491:u32)
                        }
                      }
                      n897 = Less?(x=w1472, y=w1471) -> (x < y?=w1473:bool)
                      n898 = case shown="False" w1473 {
                        tunnel: w1472 -> [w1481 w1484]
                        tunnel: w1471 -> [w1482 w1483]
                        tunnel: [w1482 w1484] -> w1467
                        tunnel: [w1481 w1483] -> w1466
                        frame False {
                        }
                        frame True {
                        }
                      }
                      n899 = local write "ROI_LowCh"(w1467) -> ()
                      n900 = local write "ROI_UpCh"(w1466) -> ()
                    }
                    event "ROI_LowCh", "ROI_UpCh": Value Change {
                      n901 = event-data() -> ()  [unwired: 1 in, 1 out]
                      n902 = local read "Intercept"() -> (w1496:dbl)
                      n903 = local read "Slope"() -> (w1501:dbl)
                      n904 = call "SUB_ChannelToEnergy.vi"("Intercept"=w1496, "Channel"="ROI_UpCh", "Slope"=w1501) -> ("Energy"=w1498:dbl)
                      n905 = call "SUB_ChannelToEnergy.vi"("Intercept"=w1496, "Channel"="ROI_LowCh", "Slope"=w1501) -> ("Energy"=w1497:dbl)
                      n906 = control-ref of="SpectraPlot"() -> (w1495:refnum<vi>)
                      n907 = property class="WFGraph (strict)"(reference=w1495, "Active Cursor"=u32 1, "Cursor.Cursor X"=w1498, "Active Cursor"=u32 0, "Cursor.Cursor X"=w1497) -> ()  [unwired: 1 in, 2 out]
                    }
                    event "ROI_Cancel": Mouse Up {
                      n908 = event-data() -> ()  [unwired: 1 in, 7 out]
                    }
                    event "ROI_Set": Mouse Up {
                      n909 = event-data() -> ()  [unwired: 1 in, 1 out]
                      n910 = call "Prompt User for Input"() -> ("ROI name"=w1506:string)  [unwired: 17 in, 2 out]
                    }
                  }
                }
              }
              frame #2 {
                n911 = case shown="True" w1510 {
                  tunnel: w1509 -> [_ w1513]
                  frame False {
                  }
                  frame True {
                    n912 = local read "ROI_LowCh"() -> (w1511:u32)
                    n913 = local read "ROI_UpCh"() -> (w1512:u32)
                    n914 = local read "Intercept"() -> (w1516:dbl)
                    n915 = local read "SpectraPlot"() -> (w1529:u64[])
                    n916 = Reshape Array(w1529, 2048 ("dimension size")) -> (w1528:u64[])
                    n917 = local read "Slope"() -> (w1515:dbl)
                    n918 = call "SUB_FitROI.vi"("Array"=w1528, "Lower"=w1511, "Upper"=w1512) -> ("Net"=w1521:i32, "centroid"=w1519:dbl, "FWHM"=w1517:dbl, "Integral"=w1520:i32, "sum"=w1522:dbl)  [unwired: 1 in]
                    n919 = call "SUB_ChannelToEnergy.vi"("Intercept"=w1516, "Channel"=w1519, "Slope"=w1515) -> ("Energy"=w1518:dbl)
                    n920 = call "SUB_ChannelToEnergy.vi"("Intercept"=w1516, "Channel"=w1517, "Slope"=w1515) -> ("Energy"=w1514:dbl)
                    n921 = Bundle By Name(cluster=T17 {"ROI name"="", "ROI begin channel"=0, "ROI end channel"=0, "Intensity"=0, "Net Intensity"=0, "Gauss Fit"=0.0, "FWHM [keV]"=0.0, "Center [keV]"=0.0} ("input cluster"), "ROI name"=w1513, "ROI begin channel"=w1511, "ROI end channel"=w1512, "Intensity"=w1520, "Net Intensity"=w1521, "Gauss Fit"=w1522, "FWHM [keV]"=w1514, "Center [keV]"=w1518) -> (w1524:T17)
                    n922 = local read "ROI_Array"() -> (w1523:T7)
                    n923 = Insert Into Array(array=w1523, new element=w1524) -> (→"ROI_Array":T7)  [unwired: 1 in]
                  }
                }
              }
              frame #3 {
                w1530 = T15."Disabled and Grayed Out" ("Disabled")
                w1531 = T15."Enabled" ("Disabled")
                w1535 = FALSE ("Cursor.Visible")
                n924 = property on="ROI_Remove" class="Bool"("DisabledEnum"=w1531) -> ()  [unwired: 2 in, 2 out]
                n925 = property on="ROI_Add" class="Bool"("DisabledEnum"=w1531) -> ()  [unwired: 2 in, 2 out]
                n926 = property on="ROI_RemoveAll" class="Bool"("DisabledEnum"=w1531) -> ()  [unwired: 2 in, 2 out]
                n927 = property on="ROI_Cancel" class="Bool (strict)"("DisabledEnum"=w1530) -> ()  [unwired: 2 in, 2 out]
                n928 = property on="ROI_Set" class="Bool (strict)"("DisabledEnum"=w1530) -> ()  [unwired: 2 in, 2 out]
                n929 = control-ref of="SpectraPlot"() -> (w1532:refnum<vi>)
                n930 = property class="WFGraph (strict)"(reference=w1532, "Active Cursor"=u32 1, "Cursor.Visible"=w1535, "Active Cursor"=u32 0, "Cursor.Visible"=w1535) -> ()  [unwired: 1 in, 2 out]
              }
              frame #4 {
                n931 = local read "ROI_Array"() -> (w1537:T7)
                n932 = for {
                  tunnel: w1537 -> [w1539] mode=indexing
                  tunnel: [w1538] -> w1536 mode=indexing
                  n933 = Unbundle By Name(w1539) -> ("ROI name"=w1538:T5)
                }
                n934 = property on="MAP-L" class="Ring (strict)"("Strings []"=w1536) -> ()  [unwired: 2 in, 2 out]
                n935 = property on="MAP-R" class="Ring (strict)"("Strings []"=w1536) -> ()  [unwired: 2 in, 2 out]
              }
            }
          }
          event "ROI_Save": Value Change {
            n936 = event-data() -> ("OldVal"=w1540:bool)  [unwired: 1 in, 5 out]
            n937 = case shown="True" w1540 {
              frame False {
              }
              frame True {
                n938 = local read "ROI_Array"() -> (w1550:T7)
                n939 = for {
                  tunnel: w1550 -> [w1556] mode=indexing
                  tunnel: [w1555] -> w1549 mode=indexing
                  tunnel: [w1553] -> w1547 mode=indexing
                  tunnel: [w1551] -> w1548 mode=indexing
                  n940 = Unbundle By Name(w1556) -> ("ROI name"=w1555:T5, "ROI begin channel"=w1554:T6, "ROI end channel"=w1552:T6)
                  n941 = Number To Decimal String(number=w1552) -> (decimal integer string=w1551:string)  [unwired: 1 in]
                  n942 = Number To Decimal String(number=w1554) -> (decimal integer string=w1553:string)  [unwired: 1 in]
                }
                n943 = Build Array(w1549, w1547, w1548) -> (w1546:T5[][])
                n944 = call "File Dialog"("pattern (all files)"="*.roi") -> ("selected path"=w1544:path)  [unwired: 11 in, 3 out]
                n945 = Transpose 2D Array(2D array=w1546) -> (transposed array=w1545:T5[][])
                n946 = call-poly <vilib>:"Write To Spreadsheet File.vi"("2D data"=w1545, "file path (dialog if empty)"=w1544) -> ()  [unwired: 6 in, 1 out]
              }
            }
          }
          event "ROI_Load": Value Change {
            n947 = event-data() -> ("NewVal"=w1557:bool)  [unwired: 1 in, 5 out]
            n948 = case shown="True" w1557 {
              frame False {
              }
              frame True {
                n949 = call-poly <vilib>:"Read From Spreadsheet File.vi"() -> ("all rows"=w1560:string[][])  [unwired: 7 in, 4 out]
                n950 = for {
                  tunnel: w1560 -> [w1573] mode=indexing
                  tunnel: [w1572] -> w1561 mode=indexing
                  tunnel: [w1571] -> w1562 mode=indexing
                  n951 = Index Array(array=w1573, index=0) -> (element=w1571:string)
                  n952 = Index Array(array=w1573, index=1) -> (element=w1567:string)
                  n953 = Index Array(array=w1573, index=2) -> (element=w1566:string)
                  n954 = Decimal String To Number(string=w1567) -> (number=w1565:i32)  [unwired: 2 in, 1 out]
                  n955 = Decimal String To Number(string=w1566) -> (number=w1564:i32)  [unwired: 2 in, 1 out]
                  n956 = Bundle By Name(cluster=T17 {"ROI name"="", "ROI begin channel"=0, "ROI end channel"=0, "Intensity"=0, "Net Intensity"=0, "Gauss Fit"=0.0, "FWHM [keV]"=0.0, "Center [keV]"=0.0} ("input cluster"), "ROI name"=w1571, "ROI begin channel"=w1565, "ROI end channel"=w1564) -> (w1572:T17)
                }
                n957 = property on="MAP-L" class="Ring (strict)"("Strings []"=w1562) -> ()  [unwired: 2 in, 2 out]
                n958 = property on="MAP-R" class="Ring (strict)"("Strings []"=w1562) -> ()  [unwired: 2 in, 2 out]
                n959 = local write "ROI_Array"(w1561) -> ()
              }
            }
          }
          event "Lin/Log": Value Change {
            n960 = event-data() -> ("NewVal"=w1574:u16)  [unwired: 1 in, 5 out]
            n961 = property on="1D graph 1" class="WFGraph (strict)"("YScale.Mapping Mode"=w1574) -> ()  [unwired: 2 in, 2 out]
            n962 = property on="1D graph 2" class="WFGraph (strict)"("YScale.Mapping Mode"=w1574) -> ()  [unwired: 2 in, 2 out]
            n963 = property on="2D graph 2" class="IntGraph (strict)"("ZScale.Mapping Mode"=w1574) -> ()  [unwired: 2 in, 2 out]
            n964 = property on="2D graph 1" class="IntGraph (strict)"("ZScale.Mapping Mode"=w1574) -> ()  [unwired: 2 in, 2 out]
          }
          event "MAP-L", "MAP-R": Value Change {
            n965 = event-data() -> ()  [unwired: 1 in, 6 out]
            n966 = local read "MAP"() -> (w1581:bool)
            n967 = case shown="True" w1581 {
              tunnel: "MAP-L" -> [w1583 w1599]
              tunnel: "MAP-R" -> [w1582 w1596]
              frame False {
                n968 = local read "1DSet"() -> (w1585:dbl[][])
                n969 = for {
                  tunnel: w1585 -> [w1591] mode=indexing
                  tunnel: w1583 -> [w1593]
                  tunnel: [w1591] -> w1586
                  i -> [w1594]
                  stop <- w1592 stop-if-true
                  n970 = Equal?(x=w1593, y=w1594) -> (x = y?=w1592:bool)
                }
                "1D graph 1" <- w1586
                n971 = for {
                  tunnel: w1585 -> [w1587] mode=indexing
                  tunnel: w1582 -> [w1589]
                  tunnel: [w1587] -> w1584
                  i -> [w1590]
                  stop <- w1588 stop-if-true
                  n972 = Equal?(x=w1589, y=w1590) -> (x = y?=w1588:bool)
                }
                "1D graph 2" <- w1584
              }
              frame True {
                n973 = local read "2DSet"() -> (w1600:dbl[][][])
                n974 = local read "2DSet"() -> (w1597:dbl[][][])
                n975 = for {
                  tunnel: w1600 -> [w1605] mode=indexing
                  tunnel: w1599 -> [w1607]
                  tunnel: [w1605] -> w1598
                  i -> [w1608]
                  stop <- w1606 stop-if-true
                  n976 = Equal?(x=w1607, y=w1608) -> (x = y?=w1606:bool)
                }
                "2D graph 1" <- w1598
                n977 = for {
                  tunnel: w1597 -> [w1601] mode=indexing
                  tunnel: w1596 -> [w1603]
                  tunnel: [w1601] -> w1595
                  i -> [w1604]
                  stop <- w1602 stop-if-true
                  n978 = Equal?(x=w1603, y=w1604) -> (x = y?=w1602:bool)
                }
                "2D graph 2" <- w1595
              }
            }
          }
          event "ROI_Remove": Value Change {
            n979 = event-data() -> ()  [unwired: 1 in, 5 out]
            n980 = stacked-sequence {
              frame #0 {
                n981 = call "Prompt User for Input2"() -> ("ROI to delete (first is 0)"=w1614:dbl, "OK"=w1612:bool)  [unwired: 17 in, 1 out]
                n982 = local read "ROI_Array"() -> (w1611:T7)
                n983 = case shown="False" w1612 {
                  tunnel: w1614 -> [_ w1619]
                  tunnel: w1611 -> [w1615 w1617]
                  tunnel: [w1615 w1616] -> w1613
                  frame False {
                  }
                  frame True {
                    n984 = Delete From Array(array=w1617, length=1, index=w1619) -> (array with subset deleted=w1616:T7)  [unwired: 1 out]
                  }
                }
                n985 = local write "ROI_Array"(w1613) -> ()
              }
              frame #1 {
                n986 = local read "ROI_Array"() -> (w1621:T7)
                n987 = for {
                  tunnel: w1621 -> [w1623] mode=indexing
                  tunnel: [w1622] -> w1620 mode=indexing
                  n988 = Unbundle By Name(w1623) -> ("ROI name"=w1622:T5)
                }
                n989 = property on="MAP-L" class="Ring (strict)"("Strings []"=w1620) -> ()  [unwired: 2 in, 2 out]
                n990 = property on="MAP-R" class="Ring (strict)"("Strings []"=w1620) -> ()  [unwired: 2 in, 2 out]
              }
            }
          }
          event "ROI_RemoveAll": Value Change {
            n991 = event-data() -> ()  [unwired: 1 in, 5 out]
            n992 = Two Button Dialog(message="Do you really want to remove all ROIs?", 1:"No" ("F button name (\"Cancel\")"), 2:"Yes" ("T button name (\"OK\")")) -> (T button?=w1625:bool)
            n993 = case shown="True" w1625 {
              frame False {
              }
              frame True {
                w1634 = T15."Disabled and Grayed Out" ("Disabled")
                n994 = property on="ROI_RemoveAll" class="Bool"("DisabledEnum"=w1634) -> ()  [unwired: 2 in, 2 out]
                n995 = property on="ROI_Remove" class="Bool"("DisabledEnum"=w1634) -> ()  [unwired: 2 in, 2 out]
                n996 = Initialize Array(T17 {"ROI name"="", "ROI begin channel"=0, "ROI end channel"=0, "Intensity"=0, "Net Intensity"=0, "Gauss Fit"=0.0, "FWHM [keV]"=0.0, "Center [keV]"=0.0} ("input cluster")) -> (w1632:T27)  [unwired: 1 in]
                n997 = local write "ROI_Array"(w1632) -> ()
                n998 = Initialize Array("") -> (w1630:string[])  [unwired: 1 in]
                n999 = property on="MAP-L" class="Ring (strict)"("Strings []"=w1630) -> ()  [unwired: 2 in, 2 out]
                n1000 = property on="MAP-R" class="Ring (strict)"("Strings []"=w1630) -> ()  [unwired: 2 in, 2 out]
              }
            }
          }
          event "CALIB_AddPoint": Value Change {
            n1001 = event-data() -> ()  [unwired: 1 in, 5 out]
            n1002 = call "Enter the peak energy in keV."() -> ("Energy [keV]"=w1644:dbl)  [unwired: 17 in, 2 out]
            n1003 = property on="SpectraPlot" class="WFGraph (strict)"("Active Cursor"=u32 2) -> ("Cursor.Cursor X"=w1636:dbl)  [unwired: 2 in, 2 out]
            n1004 = Array Size(array="CalibArray") -> (size(s)=w1640:i32[])
            n1005 = Index Array(array=w1640, index=0) -> (element=w1645:i32)
            n1006 = Increment(x=w1645) -> (x+1=w1638:i32)
            n1007 = To Double Precision Float(number=w1638) -> (double precision float=w1643:dbl)
            n1008 = Build Array(w1643, w1636, w1644) -> (w1642:dbl[])
            n1009 = Insert Into Array(array="CalibArray", new element=w1642) -> (w1641:T8)  [unwired: 2 in]
            n1010 = local write "CalibArray"(w1641) -> ()
          }
          event "CALIB_ClearPoints": Value Change {
            n1011 = event-data() -> ()  [unwired: 1 in, 5 out]
            n1012 = local write "CalibArray"(T8 [] ("SIRIUS1_CalibArray")) -> ()
          }
          event "CALIB_Execute": Value Change {
            n1013 = event-data() -> ()  [unwired: 1 in, 5 out]
            n1014 = local read "CalibArray"() -> (w1652:T8)
            n1015 = Array Size(array=w1652) -> (size(s)=w1656:i32[])
            n1016 = Index Array(array=w1656, index=0) -> (element=w1655:i32)
            n1017 = Less Or Equal?(x=w1655, y=1) -> (x <= y?=w1653:bool)
            n1018 = case shown="False" w1653 {
              tunnel: w1652 -> [w1666 _]
              tunnel: w1655 -> [w1663 _]
              frame False {
                n1019 = for {
                  N: w1663 -> [_]
                  tunnel: [w1669] -> w1665 mode=indexing
                  tunnel: [w1668] -> w1664 mode=indexing
                  tunnel: w1666 -> [w1667]
                  i -> [w1670]
                  n1020 = Index Array(array=w1667, index (row) #1=w1670, index (col) #1=1 ("index (col)"), index (row) #2=w1670, index (col) #2=2 ("index (col)")) -> (element #1=w1669:dbl, element #2=w1668:dbl)
                }
                n1021 = Two Button Dialog(message="Calibration will done" ("warning IN"), 1:"Cancel" ("Cancel text"), 2:"Proceed" ("OK text")) -> (T button?=w1659:bool)
                n1022 = case shown="True" w1659 {
                  tunnel: w1665 -> [_ w1677]
                  tunnel: w1664 -> [_ w1676]
                  frame False {
                  }
                  frame True {
                    w1678 = T28 0 items=["Least Square", "Least Absolute Residual", "Bisquare"] ("method")
                    n1023 = call <vilib>:"Linear Fit Coefficients.vi"("Y"=w1676, "X"=w1677, "method"=w1678) -> ("slope"=→"Slope":dbl, "intercept"=→"Intercept":dbl)  [unwired: 10 in, 1 out]
                    n1024 = local write "APPEARANCE_E/CH"(TRUE ("Energy/channels")) -> ()
                  }
                }
              }
              frame True {
                n1025 = One Button Dialog(message="Calibration cannot be done: not enough points!") -> ()  [unwired: 1 in, 1 out]
              }
            }
          }
          event "MEASUREMENT_Start": Value Change {
            n1026 = event-data() -> ()  [unwired: 1 in, 5 out]
          }
          event "Init": Value Change {
            n1027 = event-data() -> ()  [unwired: 1 in, 6 out]
            n1028 = control-ref of="Init"() -> ()  [unwired: 1 out]
            n1029 = call "LibraryInit.vi"("error in (no error)"=w1686) -> ("error out"=w1683:errorcluster, "Library Initialized"=w1685:bool)  [unwired: 7 in]
            n1030 = local write "Library state"(w1685) -> ()
            n1031 = Unbundle By Name(w1683) -> ("code"=w1682:i32)
            n1032 = Unbundle By Name(w1683) -> ()  [unwired: 1 out]
            n1033 = local write "Error code"(w1682) -> ()
          }
          event "Add IP": Value Change {
            n1034 = event-data() -> ()  [unwired: 1 in, 6 out]
            n1035 = control-ref of="Add IP"() -> ()  [unwired: 1 out]
            n1036 = local read "IP Address"() -> (w1690:string)
            n1037 = call "add to query.vi"("error in (no error)"=w1691, "address"=w1690) -> ("error out"=w1692:errorcluster, "function return"=w1693:bool)  [unwired: 7 in, 1 out]
            n1038 = call "CheckError.vi"("error in (no error)"=w1692, "ret_val"=w1693) -> ("error out"=w1688:errorcluster)
            n1039 = Unbundle By Name(w1688) -> ("code"=w1687:i32)
            n1040 = local write "Error code"(w1687) -> ()
          }
          event "Get connected": Value Change {
            n1041 = event-data() -> ()  [unwired: 1 in, 6 out]
            n1042 = control-ref of="Get connected"() -> ()  [unwired: 1 out]
            n1043 = call "get ids.vi"("error in (no error)"=w1698, "id_size"=u32 16 ("char_size"), "nb"=u32 0, "identifier"="") -> ("error out"=w1700:errorcluster, "identifier out"=w1697:string, "function return"=w1701:bool)  [unwired: 3 in, 2 out]
            n1044 = call "CheckError.vi"("error in (no error)"=w1700, "ret_val"=w1701) -> ("error out"=w1695:errorcluster)
            n1045 = local write "identifier out"(w1697) -> ()
            n1046 = Unbundle By Name(w1695) -> ("code"=w1694:i32)
            n1047 = local write "Error code"(w1694) -> ()
          }
          event "APPEARANCE_E/CH": Value Change {
            n1048 = event-data() -> ("NewVal"=w1706:bool)  [unwired: 1 in, 4 out]
            n1049 = flat-sequence {
              tunnel: [w1717] -> w1711
              tunnel: [w1716] -> w1710
              tunnel: [w1712] -> w1709
              tunnel: [w1713] -> w1708
              tunnel: [w1714] -> w1707
              tunnel: w1706 -> [w1712]
              tunnel: w1711 -> [w1728]
              tunnel: w1710 -> [w1727]
              tunnel: w1709 -> [w1726]
              tunnel: w1708 -> [w1719]
              tunnel: w1707 -> [w1718]
              frame #0 {
                n1050 = control-ref of="SpectraPlot"() -> (w1713:refnum<vi>)
                n1051 = property class="WFGraph (strict)"(reference=w1713, "Active Cursor"=u32 2) -> ("Cursor.Cursor X"=w1714:dbl)  [unwired: 1 in, 2 out]
                n1052 = local read "Intercept"() -> (w1716:dbl)
                n1053 = local read "Slope"() -> (w1717:dbl)
              }
              frame #1 {
                n1054 = case shown="False" w1726 {
                  tunnel: ["Channels" ("X Scale.Name Label.Text") "Energy (keV)"] -> w1725
                  tunnel: [T18 {"Format"=0, "Precision"=0} ("X Scale.Display Format") T18 {"Format"=0, "Precision"=2} ("X Scale.Display Format")] -> w1724
                  tunnel: [0.0 ("Energy 1st channel (keV)") w1739] -> w1722
                  tunnel: [1.0 ("Energy step (keV)") w1738] -> w1723
                  tunnel: [w1732 w1741] -> w1721
                  tunnel: w1727 -> [w1730 w1739]
                  tunnel: w1728 -> [w1729 w1738]
                  tunnel: w1718 -> [w1731 w1740]
                  frame False {
                    # "energy -> channels"
                    n1055 = Subtract(x=w1731, y=w1730) -> (x-y=w1733:dbl)
                    n1056 = Divide(x=w1733, y=w1729) -> (x/y=w1732:dbl)
                  }
                  frame True {
                    # "channels -> energy"
                    n1057 = Multiply(x=w1740, y=w1738) -> (x*y=w1742:dbl)
                    n1058 = Add(x=w1739, y=w1742) -> (x+y=w1741:dbl)
                  }
                }
                n1059 = property class="WFGraph (strict)"(reference=w1719, "XScale.NameLbl.Text"=w1725, "XScale.Format & Precision"=w1724, "XScale.Multiplier"=w1723, "XScale.Offset"=w1722, "Active Cursor"=u32 2, "Cursor.Cursor X"=w1721) -> ()  [unwired: 1 in, 2 out]
              }
            }
          }
          event "APPEARANCE_CursorVis": Value Change {
            n1060 = event-data() -> ("NewVal"=w1746:bool)  [unwired: 1 in]
            n1061 = property on="SpectraPlot" class="WFGraph (strict)"("Cursor Palette Vis"=w1746, "Active Cursor"=u32 2, "Cursor.Visible"=w1746) -> ()  [unwired: 2 in, 2 out]
          }
          event "APPEARANCE_Log/Lin": Value Change {
            n1062 = event-data() -> ("NewVal"=w1751:bool)  [unwired: 1 in]
            n1063 = Boolean To (0,1)(Boolean=w1751) -> (0, 1=w1750:i16)
            n1064 = property on="SpectraPlot" class="WFGraph (strict)"("YScale.Mapping Mode"=w1750) -> ()  [unwired: 2 in, 2 out]
          }
        }
        n1065 = case shown="1" w639 {
          frame 0, Default {
            w648 = T15."Disabled and Grayed Out" ("Disabled")
            n1066 = property on="Map points" class="DigNum (strict)"("DisabledEnum"=w648) -> ()  [unwired: 2 in, 2 out]
            n1067 = property on="Time per spectrum [ms]" class="DigNum (strict)"("DisabledEnum"=w648) -> ()  [unwired: 2 in, 2 out]
            n1068 = property on="Acquisition time [s]" class="DigNum (strict)"("DisabledEnum"=T15."Enabled" ("Disabled")) -> ()  [unwired: 2 in, 2 out]
          }
          frame 1 {
            w649 = T15."Enabled" ("Disabled")
            n1069 = property on="Acquisition time [s]" class="DigNum (strict)"("DisabledEnum"=T15."Disabled and Grayed Out" ("Disabled")) -> ()  [unwired: 2 in, 2 out]
            n1070 = property on="Time per spectrum [ms]" class="DigNum (strict)"("DisabledEnum"=w649) -> ()  [unwired: 2 in, 2 out]
            n1071 = property on="Map points" class="DigNum (strict)"("DisabledEnum"=w649) -> ()  [unwired: 2 in, 2 out]
          }
        }
      }
      frame "Initialisation" {
        n1072 = stacked-sequence {
          frame #0 {
            w1757 = T15."Enabled" ("Disabled")
            w1760 = T15."Disabled and Grayed Out" ("Disabled")
            w1756 = FALSE ("batch mode")
            n1073 = local write "ScanReady?"(w1756) -> ()
            n1074 = local write "scan mode"(w1756) -> ()
            n1075 = local write "queue mode"(w1756) -> ()
            n1076 = local write "QUICKSCAN_Start"(w1756) -> ()
            n1077 = local write "ZnotEqual"(w1756) -> ()
            n1078 = local write "Scan\nCorners"(dbl[][] []) -> ()
            n1079 = property on="OpenScanBuilder" class="Bool"("DisabledEnum"=T15."Disabled and Grayed Out" ("Disabled")) -> ()  [unwired: 2 in, 2 out]
            n1080 = property on="Scan definition by" class="RadioBtnsControl (strict)"("Val(Sgnl)"=T10."Scan boundaries and step size" ("Value (Signaling)")) -> ()  [unwired: 2 in, 2 out]
            n1081 = local write "X [mm]"(250.0 ("X [mm]")) -> ()
            n1082 = local write "Y [mm]"(150.0 ("Y [mm]")) -> ()
            n1083 = local write "Z [mm]"(45.0 ("Z [mm]")) -> ()
            n1084 = property on="QUICKSCAN_Start 2" class="Bool"("DisabledEnum"=w1760) -> ()  [unwired: 2 in, 2 out]
            n1085 = property on="Add To Queue 2" class="Bool"("DisabledEnum"=w1760) -> ()  [unwired: 2 in, 2 out]
            n1086 = control-ref of="This VI"() -> (w1765:refnum<vi>)
            n1087 = property class="VI"(reference=w1765, "Edit Mode"=TRUE ("Edit Mode On Open")) -> ()  [unwired: 1 in, 2 out]
            n1088 = property on="UpperLeft" class="Bool"("DisabledEnum"=w1757) -> ()  [unwired: 2 in, 2 out]
            n1089 = property on="UpperRight" class="Bool"("DisabledEnum"=w1757) -> ()  [unwired: 2 in, 2 out]
            n1090 = property on="LowerLeft" class="Bool"("DisabledEnum"=w1757) -> ()  [unwired: 2 in, 2 out]
            n1091 = property on="LowerRight" class="Bool"("DisabledEnum"=w1757) -> ()  [unwired: 2 in, 2 out]
          }
          frame #1 {
            n1092 = property on="APPEARANCE_CursorVis" class="Bool (strict)"() -> ("Value"=w1768:bool)  [unwired: 2 in, 2 out]
            n1093 = property on="APPEARANCE_Log/Lin" class="Bool (strict)"() -> ("Value"=w1769:bool)  [unwired: 2 in, 2 out]
            n1094 = property on="APPEARANCE_E/CH" class="Bool (strict)"() -> ("Value"=w1770:bool)  [unwired: 2 in, 2 out]
            n1095 = property on="APPEARANCE_CursorVis" class="Bool (strict)"("Val(Sgnl)"=w1768) -> ()  [unwired: 2 in, 2 out]
            n1096 = property on="APPEARANCE_Log/Lin" class="Bool (strict)"("Val(Sgnl)"=w1769) -> ()  [unwired: 2 in, 2 out]
            n1097 = property on="Preset type:" class="RadioBtnsControl (strict)"("Val(Sgnl)"=enum32{"Live time [s]", "Counts"}."Live time [s]" ("Value (Signaling)")) -> ()  [unwired: 2 in, 2 out]
            n1098 = property on="APPEARANCE_E/CH" class="Bool (strict)"("Val(Sgnl)"=w1770) -> ()  [unwired: 2 in, 2 out]
          }
          frame #2 {
            w1780 = 1.0 ("New Speed")
            w1781 = 10.0 ("New Speed")
            w1784 = u16 2 items=["device units", "microns/s", "mm/s", "inches/s", "degrees/s"] ("Units (0: data)")
            # "setting default speed"
            n1099 = call "Zaber_Init.vi"() -> ("Assignment"=w1785:cluster{"Microstep Size":dbl, "Device":string}[], "Axes Ass"=→"MotorsReady":bool, "VISA resource name out"=w1793:refnum<visa-resource-name>)
            "Assignment" <- w1785
            n1100 = Index Array(array=w1785, index=2) -> (element=w1772:cluster{"Microstep Size":dbl, "Device":string})
            n1101 = Index Array(array=w1785, index=1) -> (element=w1774:cluster{"Microstep Size":dbl, "Device":string})
            n1102 = Index Array(array=w1785, index=0) -> (element=w1779:cluster{"Microstep Size":dbl, "Device":string})
            n1103 = local read "ZaberError"() -> (w1794:errorcluster)
            n1104 = Unbundle(w1779) -> ("Microstep Size"=w1778:dbl, "Device"=w1777:string)
            n1105 = call "Set Speed.vi"("Units (0: data)"=w1784, "New Speed"=w1781, "error in (no error)"=w1794, "Device and Axis"=w1777, "Microstep Size (0)"=w1778, "VISA resource name"=w1793) -> ("error out"=w1790:errorcluster, "VISA resource name out"=w1789:refnum<visa-resource-name>)  [unwired: 4 in]
            n1106 = Unbundle(w1774) -> ("Microstep Size"=w1775:dbl, "Device"=w1776:string)
            n1107 = call "Set Speed.vi"("Units (0: data)"=w1784, "New Speed"=w1781, "error in (no error)"=w1790, "Device and Axis"=w1776, "Microstep Size (0)"=w1775, "VISA resource name"=w1789) -> ("error out"=w1787:errorcluster, "VISA resource name out"=w1788:refnum<visa-resource-name>)  [unwired: 4 in]
            n1108 = local write "XY Speed\n[mm/s]"(w1781) -> ()
            n1109 = Unbundle(w1772) -> ("Microstep Size"=w1773:dbl, "Device"=w1771:string)
            n1110 = call "Set Speed.vi"("Units (0: data)"=w1784, "New Speed"=w1780, "error in (no error)"=w1787, "Device and Axis"=w1771, "Microstep Size (0)"=w1773, "VISA resource name"=w1788) -> ("error out"=w1783:errorcluster, "VISA resource name out"=→"Port":refnum<visa-resource-name>)  [unwired: 4 in]
            n1111 = local write "Speed Z [mm/s]"(w1780) -> ()
            n1112 = local write "ZaberError"(w1783) -> ()
          }
        }
      }
      frame "Close" {
        n1113 = local read "ZaberError"() -> (w1798:errorcluster)
        n1114 = local read "Port"() -> (w1799:refnum<visa-resource-name>)
        n1115 = call "Close.vi"("error in (no error)"=w1798, "VISA resource name"=w1799) -> ("error out"=→"ZaberError":errorcluster)  [unwired: 9 in]
      }
    }
    n1116 = Subtract(x=w19, y=w23) -> (x-y=w21:u32)
    n1117 = Divide(x=w21, y=u32 1000) -> (x/y=w22:dbl)
    n1118 = Reciprocal(x=w22) -> (1/x=→"Loop Speed [1/s]":dbl)
    n1119 = Wait Until Next ms Multiple(millisecond multiple=u32 10) -> ()  [unwired: 1 out]
    "Enum" <- w12
  }
  n1120 = disable-structure shown="Enabled" {
    frame Disabled {
      n1121 = local read item#-1() -> ()  [unwired: 1 in]
      n1122 = local read "ZaberError"() -> ()  [unwired: 1 out]
      n1123 = local read "Port"() -> ()  [unwired: 1 in]
    }
    frame Enabled {
    }
  }
  "Library state" <- FALSE ("Library state")
